vi "Periodic Tasks.vi"(8 "error in":errorcluster) -> ()   [LabVIEW 2020]
doc: "This VI runs in parallel to other tasks. It can contain as many user-defined periodic loops as you need. These can carry out PID or other sorts of timed response."
uses:
  State Machine.ctl
  Auto State Machine.ctl
  <vilib>/Rock Robotics/WPI/DriverStation/WPI_DriverStationRobotMode2.ctl
  <vilib>/Rock Robotics/WPI/DriverStation/WPI_DriverStationAllianceInfo.ctl
  <vilib>/Rock Robotics/WPI/ThirdParty/Phoenix-LabVIEW/Motor Controller/Controls/CTRE_Phoenix_MotorControl_NeutralMode.ctl
  <vilib>/Rock Robotics/WPI/ThirdParty/Phoenix-LabVIEW/Motor Controller/Controls/CTRE_Phoenix_MotorControl_ControlMode.ctl
  <vilib>/Rock Robotics/WPI/Solenoid/WPI_SolenoidValue.ctl
  <vilib>/Rock Robotics/WPI/Utilities/WPI_GetSetVariantRefNum.vi
  <vilib>/Rock Robotics/WPI/ThirdParty/Phoenix-LabVIEW/Motor Controller/Get/CTRE_Phoenix_MotorController_GetSupplyAndStatorCurrent_Enhanced.vi
  Lime.vi
  <vilib>/Rock Robotics/Network Tables/NT Read Number.vi
  <vilib>/Rock Robotics/WPI/ThirdParty/Phoenix-LabVIEW/Motor Controller/Get/CTRE_Phoenix_MotorController_GetSelectedSensorData.vi
  <vilib>/Rock Robotics/WPI/ThirdParty/Phoenix-LabVIEW/Motor Controller/Sensor/CTRE_Phoenix_MotorControl_SetIntegratedSensorPosition_TalonFX.vi
  <vilib>/Rock Robotics/WPI/ThirdParty/Phoenix-LabVIEW/Motor Controller/Get/CTRE_Phoenix_MotorController_IntegratedSensorData_TalonFX.vi
  <vilib>/Rock Robotics/WPI/Solenoid/WPI_SolenoidSetEnum.vi
  <vilib>/Rock Robotics/Network Tables/NT Read String.vi
  <vilib>/Rock Robotics/WPI/RobotDrive/WPI_RobotDriveMecanumDrive_Cartesian.vi
  <vilib>/Rock Robotics/Network Tables/NT Write Number.vi
  <vilib>/Rock Robotics/WPI/ThirdParty/Phoenix-LabVIEW/Pigeon IMU/CTRE_PigeonIMU_GetYPR.vi
  <vilib>/addons/control/pid/pid.llb/PID (DBL).vi
  <vilib>/Rock Robotics/Network Tables/NT Write Boolean.vi
  <vilib>/Rock Robotics/Network Tables/NT Read Boolean.vi
  <vilib>/addons/control/pid/NI_PID_pid.lvlib
panel:
  in  "setpoint 8":dbl=80.0 format="%.2f"
  in  "PID gains 9":T1={"proportional gain (Kc)"=1.0, "integral time (Ti, min)"=0.016, "derivative time (Td, min)"=0.0} {"derivative time (Td, min)" format="%.3f"; "integral time (Ti, min)" format="%.3f"; "proportional gain (Kc)" format="%.3f"}
  out "Yaw 9":dbl=80.3759765625
  in  "setpoint 7":dbl=80.0 format="%.2f"
  in  "PID gains 8":T1={"proportional gain (Kc)"=1.0, "integral time (Ti, min)"=0.016, "derivative time (Td, min)"=0.0} {"derivative time (Td, min)" format="%.3f"; "integral time (Ti, min)" format="%.3f"; "proportional gain (Kc)" format="%.3f"}
  out "Yaw 8":dbl=78.8818359375
  in  "Total Time":dbl=0.9 format="%#_13g"
  in  "Time Low":dbl=0.6 format="%#_13g"
  in  "x 3":dbl=0.5
  in  "setpoint 6":dbl=60.0 format="%.2f"
  in  "PID gains 7":T1={"proportional gain (Kc)"=1.0, "integral time (Ti, min)"=0.016, "derivative time (Td, min)"=0.0} {"derivative time (Td, min)" format="%.3f"; "integral time (Ti, min)" format="%.3f"; "proportional gain (Kc)" format="%.3f"}
  out "Yaw 7":dbl=60.029296875
  in  "setpoint 5":dbl=80.0 format="%.2f"
  in  "PID gains 6":T1={"proportional gain (Kc)"=1.0, "integral time (Ti, min)"=0.016, "derivative time (Td, min)"=0.0} {"derivative time (Td, min)" format="%.3f"; "integral time (Ti, min)" format="%.3f"; "proportional gain (Kc)" format="%.3f"}
  out "Yaw 6":dbl=80.3759765625
  in  "LL Deadband":dbl=4.0
  in  "Steering K 4":dbl=0.01
  in  "Min Steer 3":dbl=0.2
  in  "Aim Deadband 3":dbl=0.5
  in  "Steering K 2":dbl=0.02
  in  "Min Steer":dbl=0.2
  in  "Aim Deadband":dbl=0.01
  in  "setpoint 4":dbl format="%.2f"
  in  "PID gains 5":T1={"proportional gain (Kc)"=1.0, "integral time (Ti, min)"=0.016, "derivative time (Td, min)"=0.0} {"derivative time (Td, min)" format="%.3f"; "integral time (Ti, min)" format="%.3f"; "proportional gain (Kc)" format="%.3f"}
  out "Yaw 5":dbl=1.3623046875
  in  "Steering K 3":dbl=0.01
  in  "Min Steer 2":dbl=0.1
  in  "Aim Deadband 2":dbl=0.01
  in  "setpoint 2":dbl format="%.2f"
  in  "PID gains 3":T1={"proportional gain (Kc)"=1.0, "integral time (Ti, min)"=0.016, "derivative time (Td, min)"=0.0} {"derivative time (Td, min)" format="%.3f"; "integral time (Ti, min)" format="%.3f"; "proportional gain (Kc)" format="%.3f"}
  out "Yaw 3":dbl=1.3623046875
  in  "setpoint":dbl format="%.2f"
  in  "PID gains 2":T1={"proportional gain (Kc)"=1.0, "integral time (Ti, min)"=0.016, "derivative time (Td, min)"=0.0} {"derivative time (Td, min)" format="%.3f"; "integral time (Ti, min)" format="%.3f"; "proportional gain (Kc)" format="%.3f"}
  out "Yaw 2":dbl=0.263671875
  in  "Time Target (s)":dbl=0.1
  out "Timer":dbl
  out "Yaw":dbl
  in  "Oncontact 2 RPM 3":dbl=1100.0
  in  "Oncontact 2 RPM 2":dbl=1100.0
  in  "Auto On Contact RPM":dbl=1100.0
  out "Present (s)":dbl
  in  "Shooter Speed while intake":dbl=0.4
  out "Mag Current":dbl
  in  "Current Limit":dbl=25.0
  out "Mag Limit":bool
  out "Missed Mag":bool=TRUE
  in  "PID gains":T1={"proportional gain (Kc)"=1.0, "integral time (Ti, min)"=0.01, "derivative time (Td, min)"=0.0} {"derivative time (Td, min)" format="%.3f"; "integral time (Ti, min)" format="%.3f"; "proportional gain (Kc)" format="%.3f"}
  in  "Desired Mag Position":dbl format="%.2f"
  out "BB2":bool=TRUE
  out "BB1":bool
  out "Position":i32=403426
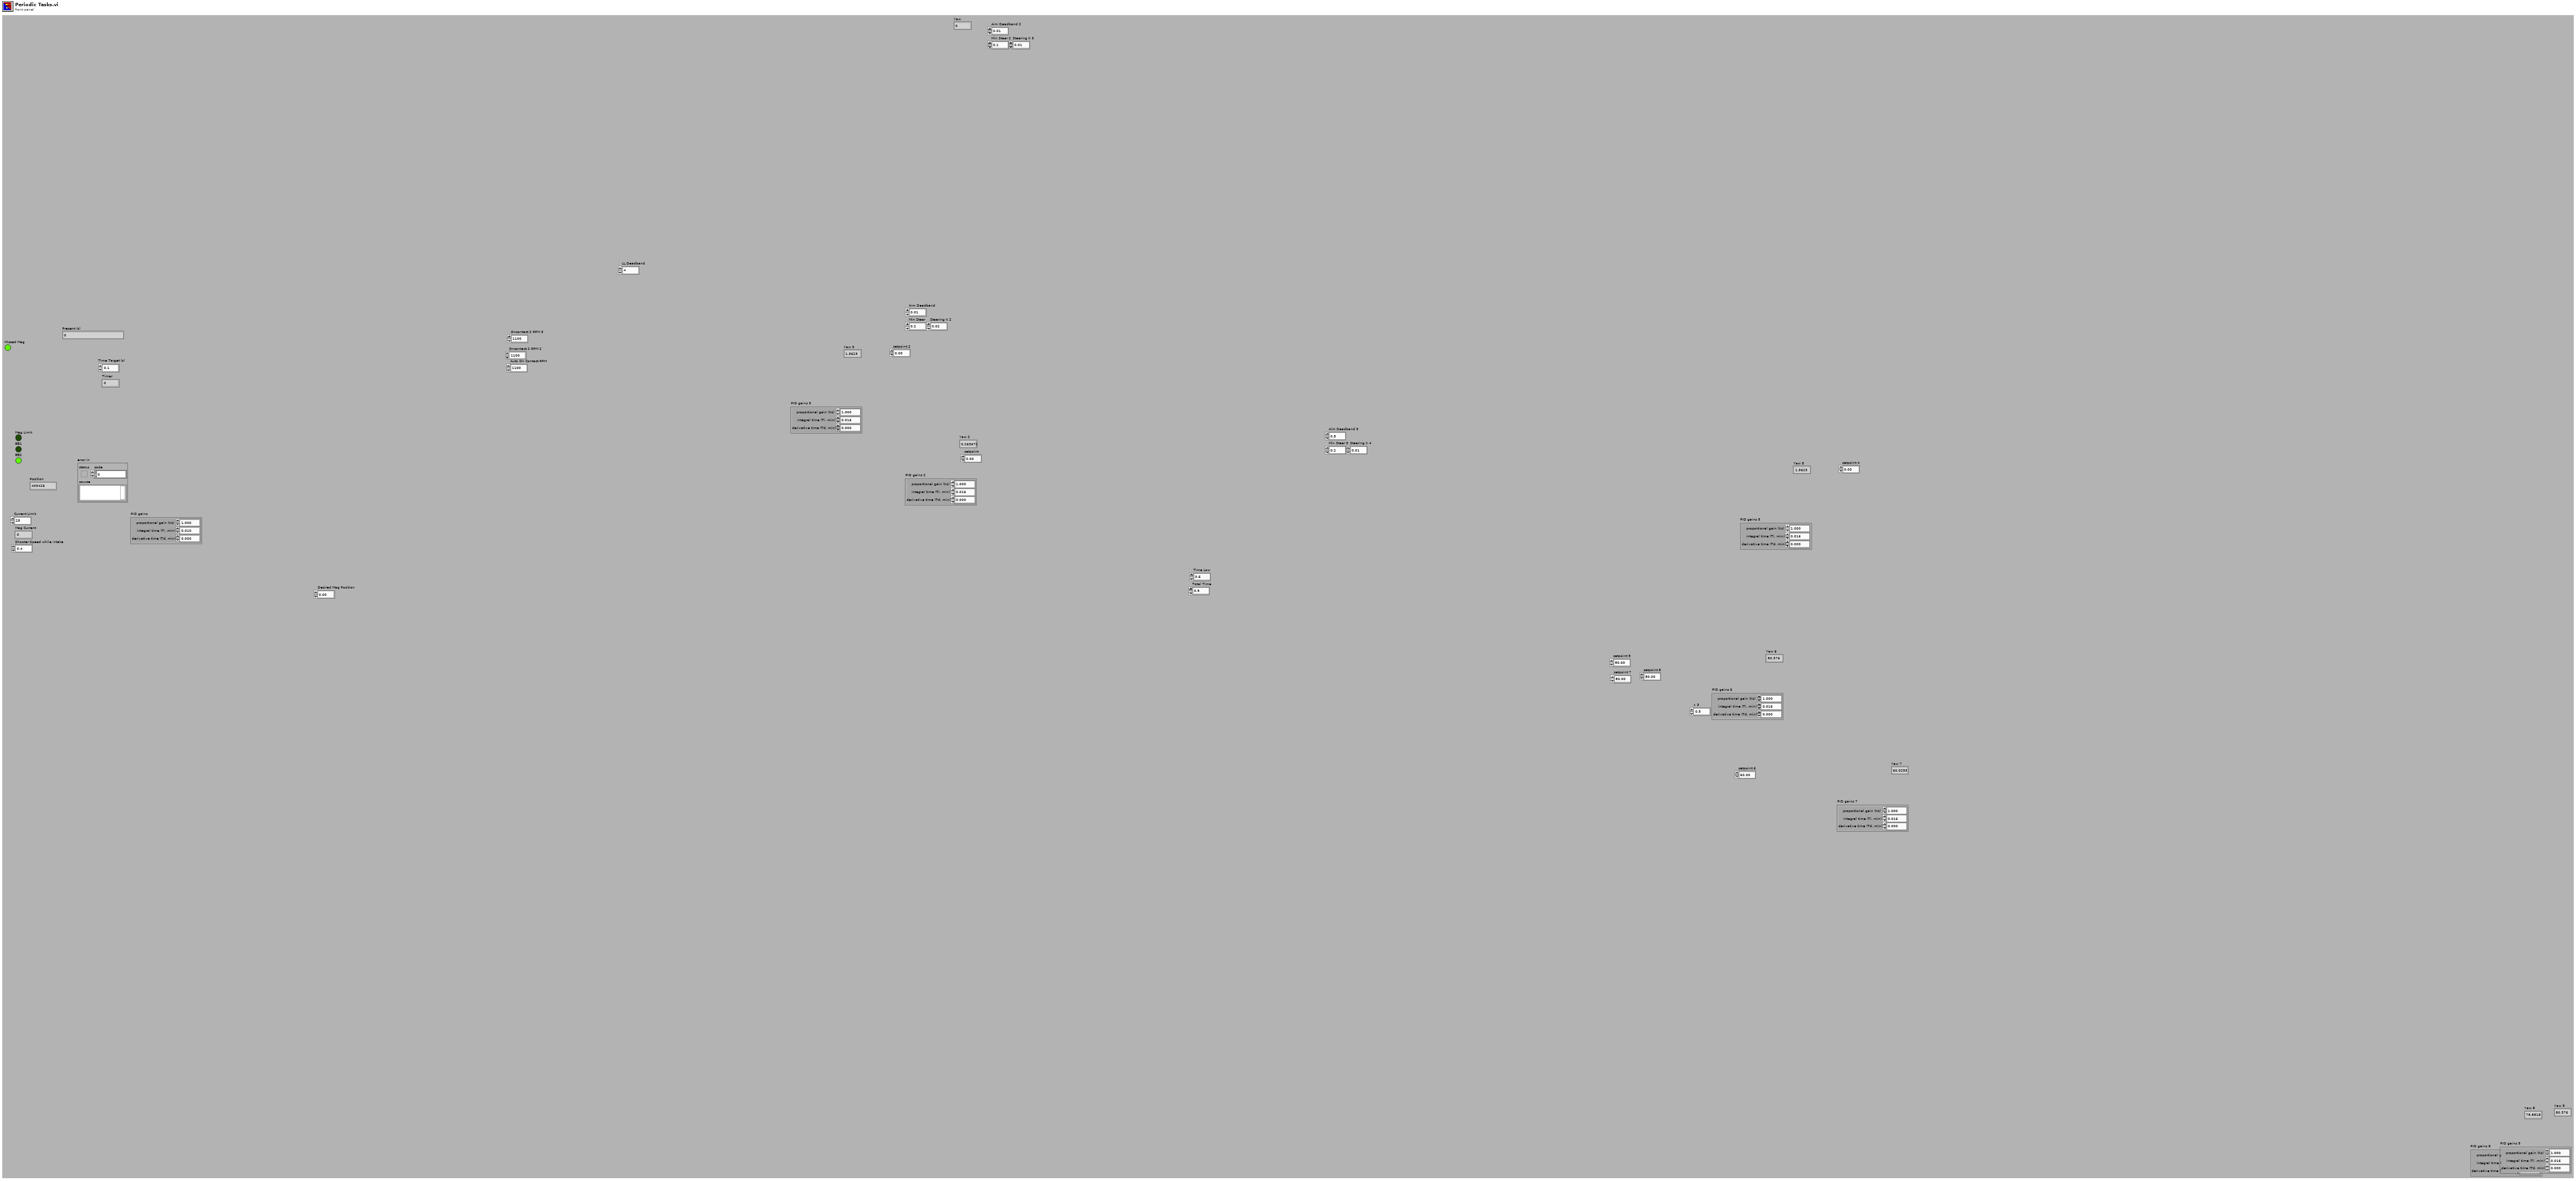
[diagram p1: front panel]
types:
  T1 = cluster{"proportional gain (Kc)":dbl, "integral time (Ti, min)":dbl, "derivative time (Td, min)":dbl}
  T2 = typedef "Auto State Machine.ctl" = enum16{"Auto Wait", "Shoot OC 1", "Shoot OC 2", "Shoot OC 3", "OC Reverse", "Cam Swap 1", "Cam Swap 2", "Cam Swap 3", "Go To Ball", "Intake", "Intake Up", "Rotate & Auger", "Limelight Happy?", "LL Shoot 1", "LL Shoot 2", "Pigeon Rotate", "Pigeon Shoot 1", "Pigeon Shoot 2", "Reverse", "Stop"}
  T3 = typedef "State Machine.ctl" = enum16{"Wait", "Conveyor 1", "Conveyor 2", "Dash Shoot 1", "Dash Shoot 2", "Low Goal Shoot 1", "Low Goal Shoot 2", "Launch Pad Shoot 1", "Launch Pad Shoot 2", "Wall Shoot 1", "Wall Shoot 2", "Mag Overcurrent"}
  T4 = typedef "CTRE_Phoenix_MotorControl_NeutralMode.ctl" = enum8{"EEPROMSetting", "Override to Coast", "Override to Brake"}
  T5 = typedef "WPI_DigitalInputDevRef.ctl" = cluster{"DevStatus":errorcluster, "DIO Channel":T6}
  T6 = typedef "FPGA_DIOChannel.ctl" = enum8{"DIO 0", "DIO 1", "DIO 2", "DIO 3", "DIO 4", "DIO 5", "DIO 6", "DIO 7", "DIO 8", "DIO 9", "DIO MXP 0", "DIO MXP 1", "DIO MXP 2", "DIO MXP 3", "DIO MXP 4", "DIO MXP 5", "DIO MXP 6", "DIO MXP 7", "DIO MXP 8", "DIO MXP 9", "DIO MXP 10", "DIO MXP 11", "DIO MXP 12", "DIO MXP 13", "DIO MXP 14", "DIO MXP 15", "SPI Port CS1", "SPI Port CS2", "SPI Port CS3", "SPI Port MISO", "SPI Port MOSI", "Invalid"}
  T7 = typedef "WPI_MotorControlDeviceRef.ctl" = cluster{"DeviceStatus":errorcluster, "Type":T8, "PWM":cluster{"PWM Channel":T9, "DeadBand":T10}, "CAN":cluster{"Device Number":u8, "SetOutput VI Ref":variant, "GetOutput VI Ref":variant, "Enable VI Ref":variant, "Disable VI Ref":variant, "Data":variant}, "Invert":bool, "DIO PWM":cluster{"PWM \"Enable\" Channel":T9, "DIOChannel":T6, "PWM Rate":dbl}}
  T8 = typedef "WPI_MotorControlType.ctl" = enum16{"PWM", "CAN", "DIO PWM"}
  T9 = typedef "FPGA_DIOPWMChannel.ctl" = enum8{"PWM 0", "PWM 1", "PWM 2", "PWM 3", "PWM 4", "PWM 5", "PWM 6", "PWM 7", "PWM 8", "PWM 9", "PWM MXP 0", "PWM MXP 1", "PWM MXP 2", "PWM MXP 3", "PWM MXP 4", "PWM MXP 5", "PWM MXP 6", "PWM MXP 7", "PWM MXP 8", "PWM MXP 9", "Invalid"}
  T10 = typedef "WPI_PWMDeadband.ctl" = cluster{"Name":string, "maxPositivePwm":i32, "minPositivePwm":i32, "centerPwm":i32, "maxNegativePwm":i32, "minNegativePwm":i32, "angularRange":u16}
  T11 = typedef "CTRE_PigeonIMU_DeviceRef.ctl" = cluster{"DeviceStatus":errorcluster, "Device Number":u8, "Type":T12, "Device ID":u32, "Handle":u64, "UsageFrame":u32, "Library Path":path}
  T12 = typedef "CTRE_PigeonIMU_ConnectionType.ctl" = u32
  T13 = typedef "WPI_DriverStationRobotMode2.ctl" = enum16{"Autonomous Disabled", "Autonomous Enabled", "Teleop Disabled", "Teleop Enabled", "Disconnected", "Finish", "Test Disabled", "Test Enabled", "Emergency Stopped"}
  T14 = typedef "WPI_JoystickDevRef.ctl" = cluster{"Device":T15}
  T15 = typedef "WPI_JoystickDeviceEnum.ctl" = enum16{"USB 0", "USB 1", "USB 2", "USB 3", "USB 4", "USB 5"}
  T16 = typedef "CTRE_Phoenix_MotorControl_ControlMode.ctl" = u16
  T17 = typedef "WPI_DriverStationAllianceInfo.ctl" = enum16{"Red", "Blue", "Invalid"}
  T18 = typedef "WPI_SolenoidValue.ctl" = enum16{"Off", "On", "Forward", "Reverse"}
  T19 = typedef "WPI_SolenoidDevRef.ctl" = cluster{"DevStatus":errorcluster, "Pneumatics Control Module":u8, "Forward Solenoid Channel":T20, "Reverse Solenoid Channel":T20}
  T20 = typedef "WPI_SolenoidChannel.ctl" = enum8{"Solenoid 0", "Solenoid 1", "Solenoid 2", "Solenoid 3", "Solenoid 4", "Solenoid 5", "Solenoid 6", "Solenoid 7", "Solenoid 8", "Solenoid 9", "Solenoid 10", "Solenoid 11", "Solenoid 12", "Solenoid 13", "Solenoid 14", "Solenoid 15", "Invalid"}
  T21 = typedef "WPI_RobotDriveDevRef.ctl" = cluster{"DevStatus":errorcluster, "Motors[]":T7[], "Square Inputs":bool, "Max Output":dbl}
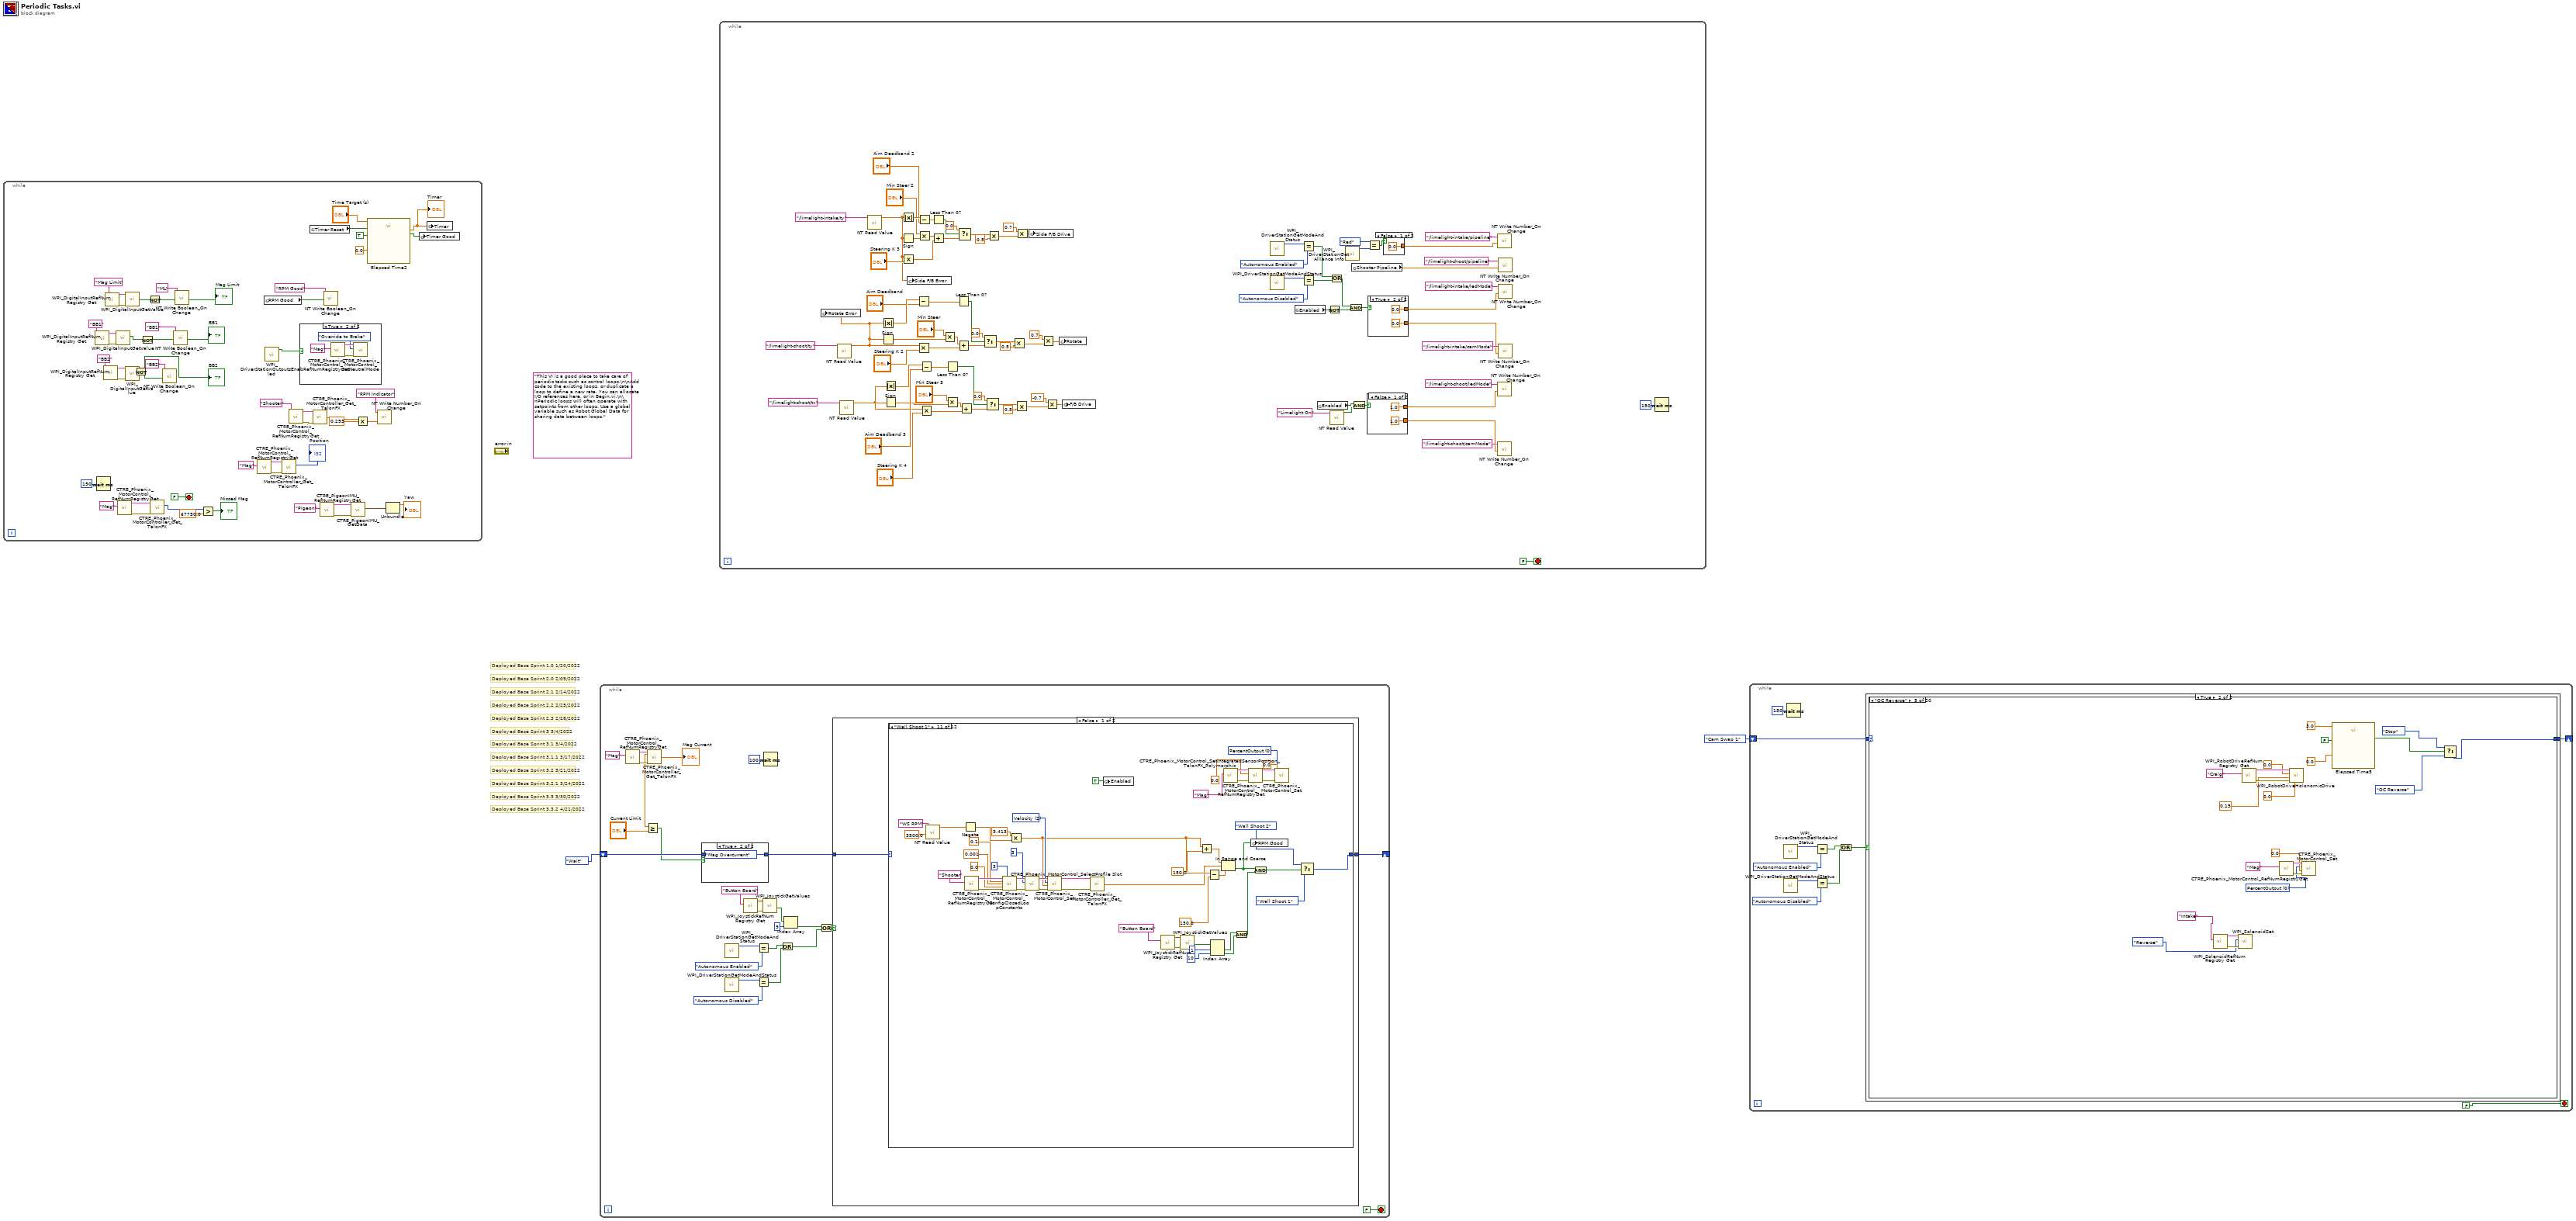
[diagram p0: block diagram]
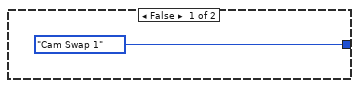
[diagram p2: hidden frame]
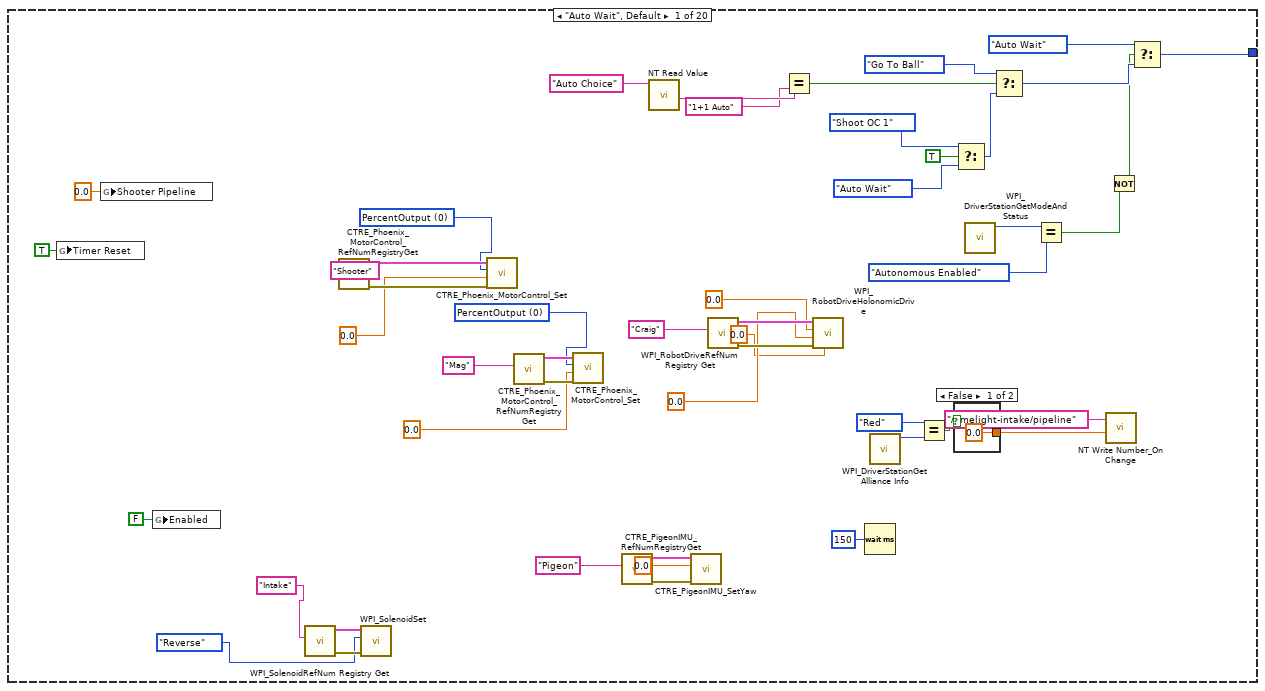
[diagram p3: hidden frame]
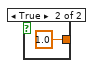
[diagram p4: hidden frame]
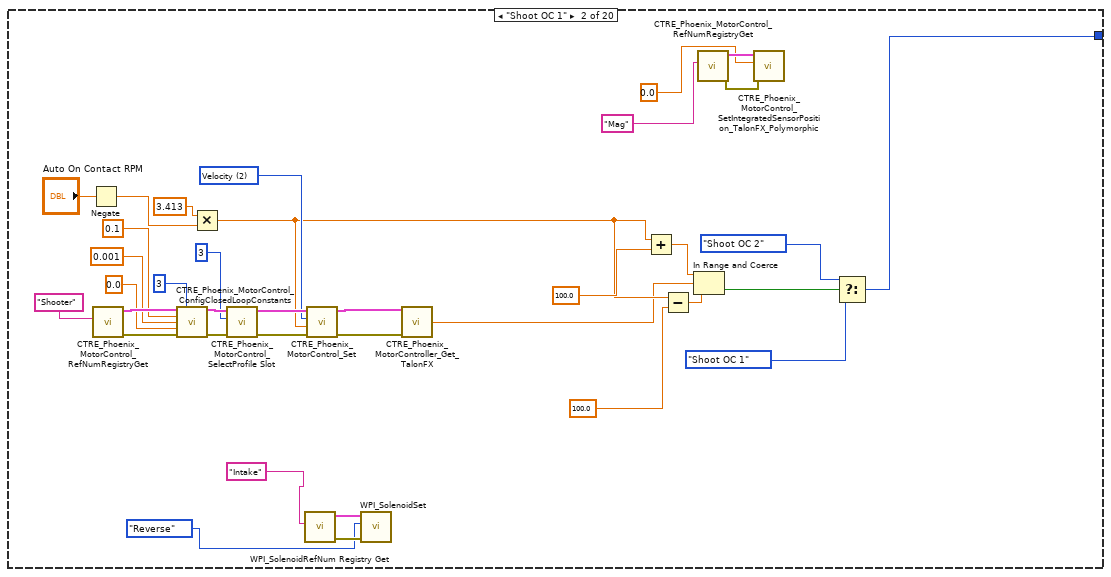
[diagram p5: hidden frame]
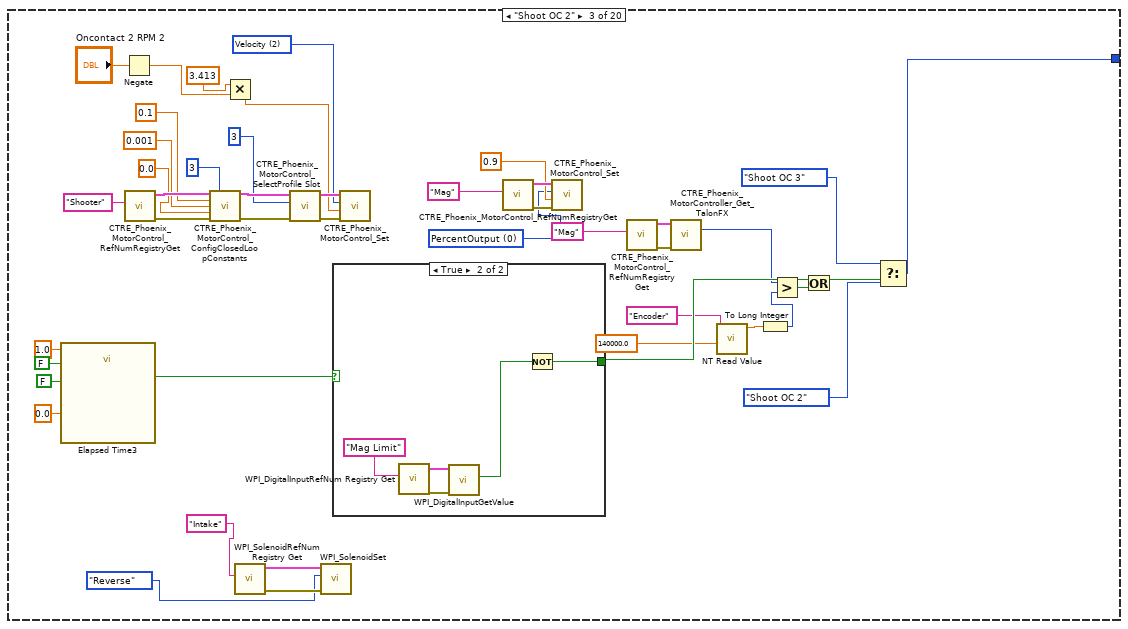
[diagram p6: hidden frame]
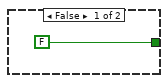
[diagram p7: hidden frame]
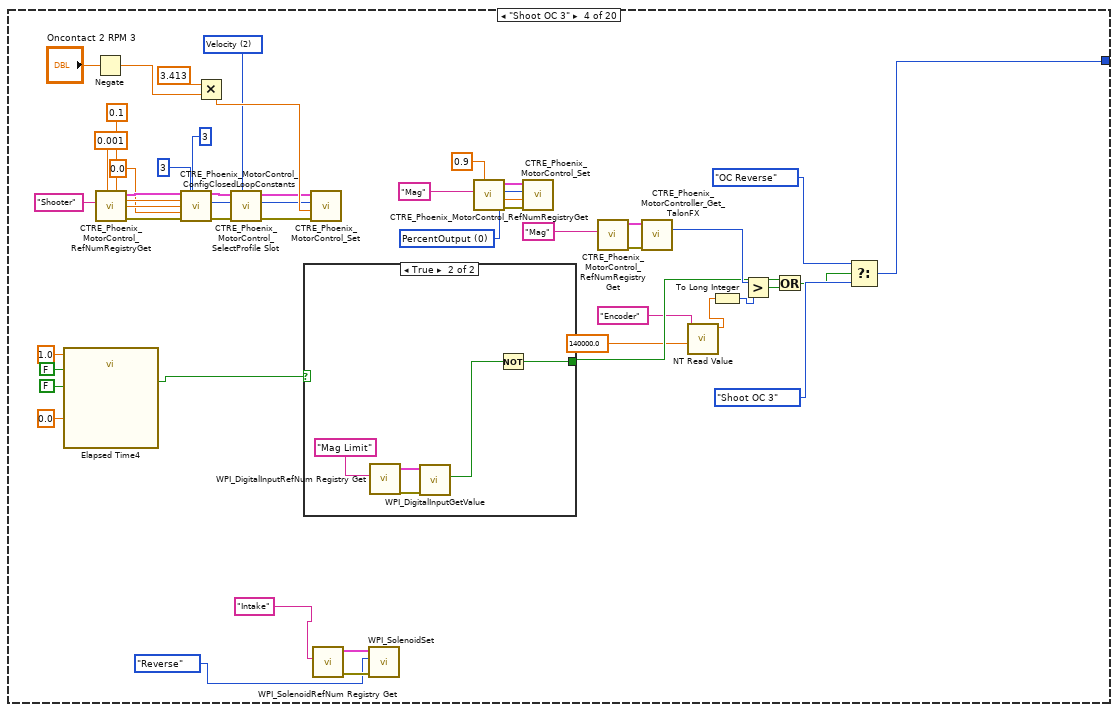
[diagram p8: hidden frame]
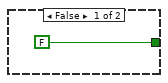
[diagram p9: hidden frame]
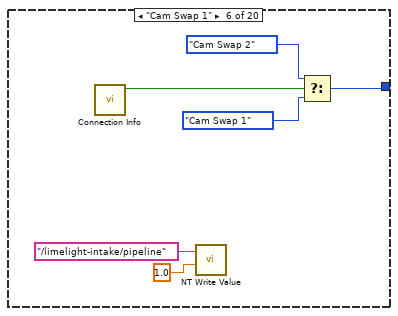
[diagram p10: hidden frame]
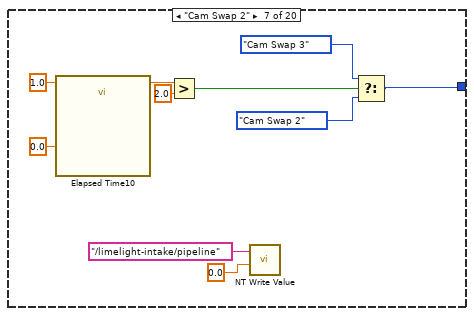
[diagram p11: hidden frame]
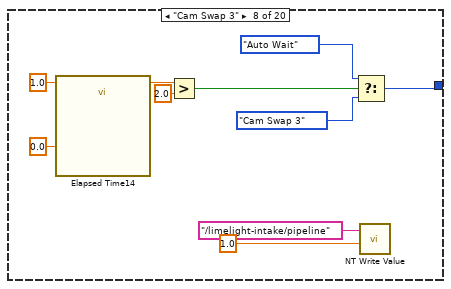
[diagram p12: hidden frame]
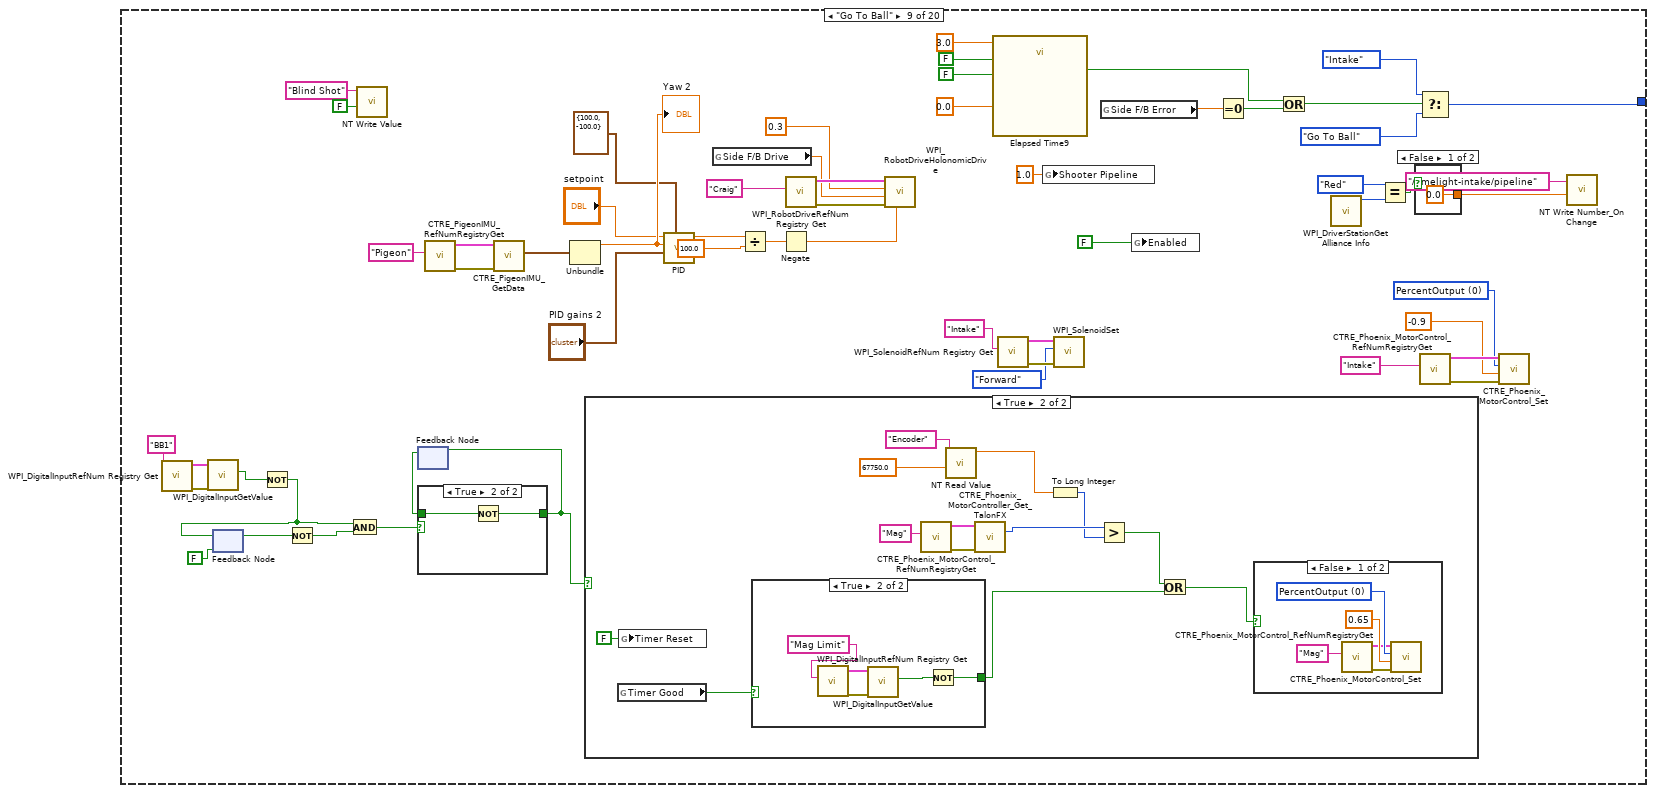
[diagram p13: hidden frame]
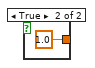
[diagram p14: hidden frame]
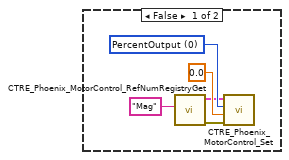
[diagram p16: hidden frame]
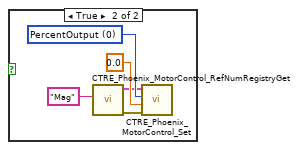
[diagram p17: hidden frame]
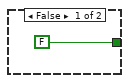
[diagram p18: hidden frame]
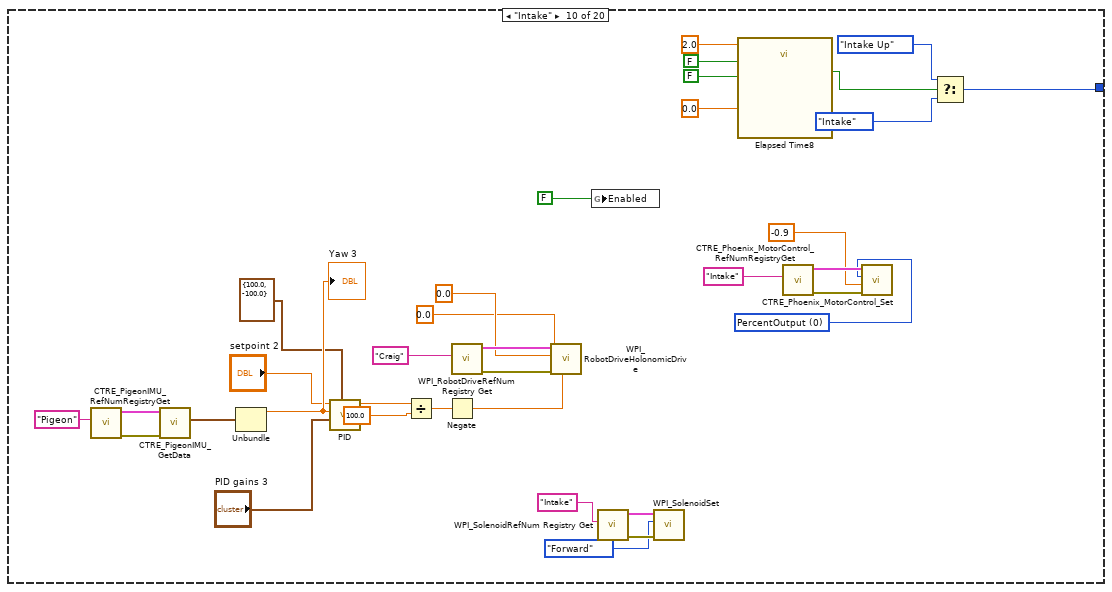
[diagram p19: hidden frame]
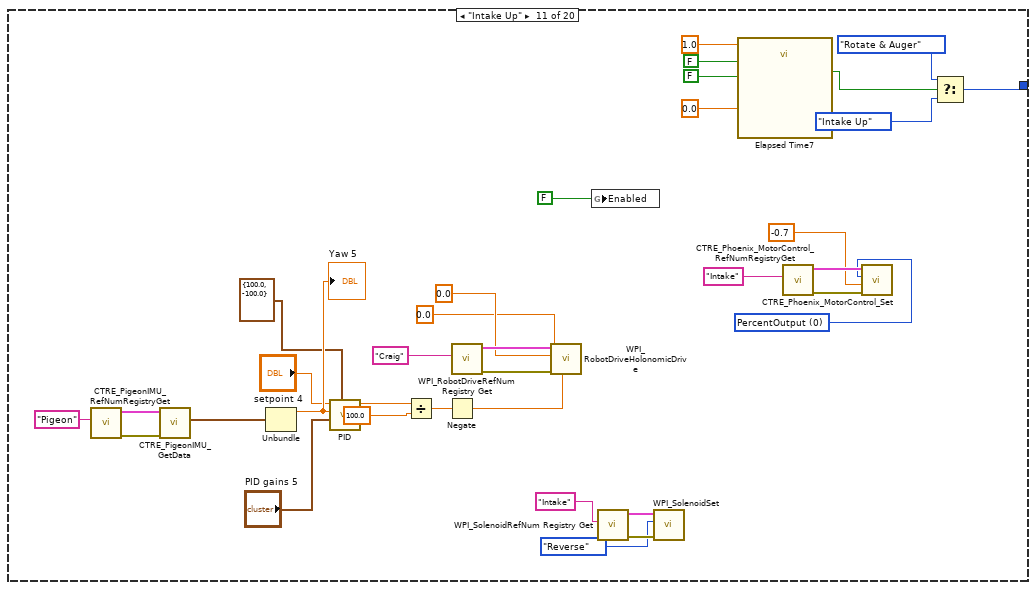
[diagram p20: hidden frame]
diagram:
  (unwired) "This VI is a good place to take care of periodic tasks such as control loops.\n\nAdd code to the existing loops, or duplicate a loop to define a new rate. You can allocate I/O references here, or in Begin.vi.\n\nPeriodic loops will often operate with setpoints from other loops. Use a global variable such as Robot Global Data for sharing data between loops."
  # "Deployed Base Sprint 3.3.2 4/21/2022"
  # "Deployed Base Sprint 3.3 3/30/2022"
  # "Deployed Base Sprint 3.2.1 3/24/2022"
  # "Deployed Base Sprint 3.2 3/21/2022"
  # "Deployed Base Sprint 3.1.1 3/17/2022"
  # "Deployed Base Sprint 3.1 3/4/2022"
  # "Deployed Base Sprint 3 3/4/2022"
  # "Deployed Base Sprint 2.3 2/28/2022"
  # "Deployed Base Sprint 2.2 2/25/2022"
  # "Deployed Base Sprint 2.1 2/14/2022"
  # "Deployed Base Sprint 2.0 2/09/2022"
  # "Deployed Base Sprint 1.0 1/20/2022"
  n1 = while {
    stop <- FALSE stop-if-true
    n2 = call <vilib>:"WPI_DigitalInputRefNum Registry Get.vi"("refnum name"="BB1") -> ("error out"=w48:errorcluster, "DigitalInputDevRef"=w47:T5)  [unwired: 9 in]
    n3 = Wait (ms)(milliseconds to wait=u32 150) -> ()  [unwired: 1 out]
    n4 = call <vilib>:"WPI_DigitalInputRefNum Registry Get.vi"("refnum name"="BB2") -> ("error out"=w45:errorcluster, "DigitalInputDevRef"=w46:T5)  [unwired: 9 in]
    n5 = call <vilib>:"WPI_DigitalInputRefNum Registry Get.vi"("refnum name"="Mag Limit") -> ("error out"=w20:errorcluster, "DigitalInputDevRef"=w21:T5)  [unwired: 9 in]
    n6 = call <vilib>:"WPI_DigitalInputGetValue.vi"("error in (no error)"=w48, "DigitalInputDevRef"=w47) -> ("Value"=w44:bool)  [unwired: 7 in, 2 out]
    n7 = call <vilib>:"CTRE_Phoenix_MotorControl_RefNumRegistryGet.vi"("refnum name"="Mag") -> ("error out"=w28:errorcluster, "PhoenixMotorControlDevRef"=w27:T7)  [unwired: 9 in]
    n8 = call <vilib>:"WPI_DigitalInputGetValue.vi"("error in (no error)"=w45, "DigitalInputDevRef"=w46) -> ("Value"=w37:bool)  [unwired: 7 in, 2 out]
    n9 = call <vilib>:"WPI_DigitalInputGetValue.vi"("error in (no error)"=w20, "DigitalInputDevRef"=w21) -> ("Value"=w22:bool)  [unwired: 7 in, 2 out]
    n10 = Not(x=w37) -> (.not. x?=w36:bool)
    "BB2" <- w36
    n11 = Not(x=w44) -> (.not. x?=w38:bool)
    "BB1" <- w38
    n12 = Not(x=w22) -> (.not. x?=w17:bool)
    "Mag Limit" <- w17
    n13 = call-poly <vilib>:"CTRE_Phoenix_MotorController_Get_TalonFX.vi"("PhoenixMotorControlDevRef"=w27, "error in"=w28) -> ("Position (Raw Sensor Units)"=w25:i32)  [unwired: 10 in, 3 out]
    n14 = call "NT Write Boolean_On Change.vi"("Boolean"=w36, "Name"="BB2") -> ()  [unwired: 9 in, 1 out]
    n15 = call "NT Write Boolean_On Change.vi"("Boolean"=w38, "Name"="BB1") -> ()  [unwired: 9 in, 1 out]
    n16 = call "NT Write Boolean_On Change.vi"("Boolean"=w17, "Name"="ML") -> ()  [unwired: 9 in, 1 out]
    n17 = Greater?(x=w25, y=67750.0) -> (0:→"Missed Mag":bool)
    n18 = call <vilib>:"CTRE_Phoenix_MotorControl_RefNumRegistryGet.vi"("refnum name"="Mag") -> ("error out"=w41:errorcluster, "PhoenixMotorControlDevRef"=w42:T7)  [unwired: 9 in]
    n19 = global read "Lime.vi" "RPM Good"() -> (w11:bool)
    n20 = call <vilib>:"WPI_DriverStationOutputsEnabled.vi"() -> ("OutputsEnabled?"=w39:bool)  [unwired: 10 in, 1 out]
    n21 = call-poly <vilib>:"CTRE_Phoenix_MotorController_Get_TalonFX.vi"("PhoenixMotorControlDevRef"=w42, "error in"=w41) -> ("Position (Raw Sensor Units)"=→"Position":i32)  [unwired: 10 in, 3 out]
    n22 = call <vilib>:"CTRE_Phoenix_MotorControl_RefNumRegistryGet.vi"("refnum name"="Shooter") -> ("error out"=w30:errorcluster, "PhoenixMotorControlDevRef"=w29:T7)  [unwired: 9 in]
    n23 = case shown="True" w39 {
      frame False {
        n24 = call <vilib>:"CTRE_Phoenix_MotorControl_RefNumRegistryGet.vi"("refnum name"="Mag") -> ("error out"=w56:errorcluster, "PhoenixMotorControlDevRef"=w55:T7)  [unwired: 9 in]
        n25 = call <vilib>:"CTRE_Phoenix_MotorControl_SetNeutralMode.vi"("error in (no error)"=w56, "Motor Control Neutral Mode"=CTRE_Phoenix_MotorControl_NeutralMode."Override to Coast", "PhoenixMotorControlDevRef"=w55) -> ()  [unwired: 7 in, 2 out]
      }
      frame True {
        n26 = call <vilib>:"CTRE_Phoenix_MotorControl_RefNumRegistryGet.vi"("refnum name"="Mag") -> ("error out"=w60:errorcluster, "PhoenixMotorControlDevRef"=w59:T7)  [unwired: 9 in]
        n27 = call <vilib>:"CTRE_Phoenix_MotorControl_SetNeutralMode.vi"("error in (no error)"=w60, "Motor Control Neutral Mode"=CTRE_Phoenix_MotorControl_NeutralMode."Override to Brake", "PhoenixMotorControlDevRef"=w59) -> ()  [unwired: 7 in, 2 out]
      }
    }
    n28 = global read "Lime.vi" "Timer Reset"() -> (w8:bool)
    n29 = call-poly <vilib>:"CTRE_Phoenix_MotorController_Get_TalonFX.vi"("PhoenixMotorControlDevRef"=w29, "error in"=w30) -> ("Velocity"=w34:dbl)  [unwired: 9 in, 4 out]
    n30 = call <vilib>:"CTRE_PigeonIMU_RefNumRegistryGet.vi"("refnum name"="Pigeon") -> ("error out"=w15:errorcluster, "PigeonIMUDevRef"=w16:T11)  [unwired: 9 in]
    n31 = call "NT Write Boolean_On Change.vi"("Boolean"=w11, "Name"="RPM Good") -> ()  [unwired: 9 in, 1 out]
    n32 = call-poly <vilib>:"CTRE_PigeonIMU_GetData.vi"("error in (no error)"=w15, "PigeonIMUDevRef"=w16) -> ("Yaw Pitch Roll"=w13:cluster{"Yaw":dbl, "Pitch":dbl, "Roll":dbl})  [unwired: 7 in, 2 out]
    n33 = Multiply(x=w34, y=0.293) -> (x*y=w31:dbl)
    n34 = call "Elapsed Time2"("Time Target (s)"="Time Target (s)", "Reset"=w8, "Auto Reset"=TRUE, "Set Start Time (s)"=0.0) -> ("Elapsed Time (s)"=w4:dbl, "Time has Elapsed"=w7:bool)  [unwired: 8 in, 6 out]
    "Timer" <- w4
    n35 = call "NT Write Number_On Change.vi"("Numeric"=w31, "Name"="RPM Indicator") -> ()  [unwired: 9 in, 1 out]
    n36 = Unbundle(w13) -> ("Yaw"=→"Yaw":dbl)  [unwired: 2 out]
    n37 = global write "Lime.vi" "Timer Good"(w7) -> ()
    n38 = global write "Lime.vi" "Timer"(w4) -> ()
  }
  n39 = while {
    shift-right: [w81] -> _
    shift-left: State_Machine."Wait" -> [w77]
    stop <- FALSE stop-if-true
    n40 = call <vilib>:"CTRE_Phoenix_MotorControl_RefNumRegistryGet.vi"("refnum name"="Mag") -> ("error out"=w74:errorcluster, "PhoenixMotorControlDevRef"=w75:T7)  [unwired: 9 in]
    n41 = call-poly <vilib>:"CTRE_Phoenix_MotorController_Get_TalonFX.vi"("PhoenixMotorControlDevRef"=w75, "error in"=w74) -> ("Supply Current"=w73:dbl, "Stator Current"=→"Mag Current":dbl)  [unwired: 10 in, 2 out]
    n42 = Greater Or Equal?(x=w73, y="Current Limit") -> (x >= y?=w70:bool)
    n43 = case shown="True" w70 {
      tunnel: [w88 State_Machine."Mag Overcurrent"] -> w78
      tunnel: w77 -> [w88 _]
      frame False {
      }
      frame True {
      }
    }
    n44 = call <vilib>:"WPI_DriverStationGetModeAndStatus.vi"() -> ("Robot Mode"=w68:T13)  [unwired: 10 in, 1 out]
    n45 = call <vilib>:"WPI_DriverStationGetModeAndStatus.vi"() -> ("Robot Mode"=w66:T13)  [unwired: 10 in, 1 out]
    n46 = call <vilib>:"WPI_JoystickRefNum Registry Get.vi"("refnum name"="Button Board") -> ("error out"=w87:errorcluster, "JoystickDevRef"=w86:T14)  [unwired: 9 in]
    n47 = Equal?(x=w68, y=WPI_DriverStationRobotMode2."Autonomous Enabled") -> (x = y?=w64:bool)
    n48 = Equal?(x=w66, y=WPI_DriverStationRobotMode2."Autonomous Disabled") -> (x = y?=w63:bool)
    n49 = call <vilib>:"WPI_JoystickGetValues.vi"("error in (no error)"=w87, "JoystickDevRef"=w86) -> ("Buttons"=w84:bool[])  [unwired: 5 in, 4 out]
    n50 = Wait (ms)(milliseconds to wait=u32 100) -> ()  [unwired: 1 out]
    n51 = Or(x=w64, y=w63) -> (x .or. y?=w62:bool)
    n52 = Index Array(array=w84, index=9) -> (element=w80:bool)
    n53 = Or(x=w80, y=w62) -> (x .or. y?=w69:bool)
    n54 = case shown="False" w69 {
      tunnel: w78 -> [w91 _]
      tunnel: [w90 State_Machine."Wait"] -> w81
      frame False {
        n55 = case shown="\"Wall Shoot 1\"" w91 {
          tunnel: [w110 w153 w184 w239 w296 w329 w349 w396 w441 w489 w533 w583] -> w90
          frame "Wait", Default {
            w104 = T16 0 items=["PercentOutput"=0, "Position"=1, "Velocity"=2, "Current"=3, "Follower"=5, "MotionProfile"=6, "MotionMagic"=7, "MotionProfileArc"=10, "Disabled"=15] ("Control Mode")
            w101 = T16 0 items=["PercentOutput"=0, "Position"=1, "Velocity"=2, "Current"=3, "Follower"=5, "MotionProfile"=6, "MotionMagic"=7, "MotionProfileArc"=10, "Disabled"=15] ("Control Mode")
            n56 = call <vilib>:"WPI_JoystickRefNum Registry Get.vi"("refnum name"="Button Board") -> ("error out"=w144:errorcluster, "JoystickDevRef"=w145:T14)  [unwired: 9 in]
            n57 = call <vilib>:"WPI_JoystickGetValues.vi"("error in (no error)"=w144, "JoystickDevRef"=w145) -> ("Buttons"=w141:bool[])  [unwired: 5 in, 4 out]
            n58 = Index Array(array=w141, index #1=0 ("index"), index #2=3 ("index"), index #3=6 ("index"), index #4=1 ("index")) -> (element #1=w140:bool, element #2=w117:bool, element #3=w118:bool, element #4=w93:bool)
            n59 = call <vilib>:"WPI_DigitalInputRefNum Registry Get.vi"("refnum name"="BB2") -> ("error out"=w130:errorcluster, "DigitalInputDevRef"=w129:T5)  [unwired: 9 in]
            n60 = call <vilib>:"WPI_DigitalInputRefNum Registry Get.vi"("refnum name"="BB1") -> ("error out"=w133:errorcluster, "DigitalInputDevRef"=w134:T5)  [unwired: 9 in]
            n61 = call <vilib>:"WPI_JoystickRefNum Registry Get.vi"("refnum name"="Joystick 0") -> ("error out"=w135:errorcluster, "JoystickDevRef"=w136:T14)  [unwired: 9 in]
            n62 = call <vilib>:"WPI_DigitalInputGetValue.vi"("error in (no error)"=w130, "DigitalInputDevRef"=w129) -> ("Value"=w127:bool)  [unwired: 7 in, 2 out]
            n63 = call <vilib>:"WPI_DigitalInputGetValue.vi"("error in (no error)"=w133, "DigitalInputDevRef"=w134) -> ("Value"=w128:bool)  [unwired: 7 in, 2 out]
            n64 = Select(t=State_Machine."Wall Shoot 1", s=w93, f=State_Machine."Wait") -> (s? t:f=w96:T3)
            n65 = Not(x=w127) -> (.not. x?=w123:bool)
            n66 = Not(x=w128) -> (.not. x?=w126:bool)
            n67 = Select(t=State_Machine."Launch Pad Shoot 1", s=w118, f=w96) -> (s? t:f=w115:T3)
            n68 = call <vilib>:"WPI_JoystickGetValues.vi"("error in (no error)"=w135, "JoystickDevRef"=w136) -> ("Buttons"=w138:bool[])  [unwired: 5 in, 4 out]
            n69 = Select(t=State_Machine."Low Goal Shoot 1", s=w117, f=w115) -> (s? t:f=w116:T3)
            n70 = Index Array(array=w138, index=1) -> (element=w121:bool)
            n71 = Select(t=FALSE, s=w123, f=w126) -> (s? t:f=w125:bool)
            n72 = call <vilib>:"CTRE_Phoenix_MotorControl_RefNumRegistryGet.vi"("refnum name"="Shooter") -> ("error out"=w108:errorcluster, "PhoenixMotorControlDevRef"=w109:T7)  [unwired: 9 in]
            n73 = Or(x=w121, y=w125) -> (x .or. y?=w122:bool)
            n74 = Select(t=State_Machine."Dash Shoot 1", s=w140, f=w116) -> (s? t:f=w146:T3)
            n75 = Select(t=State_Machine."Conveyor 1", s=w122, f=w146) -> (s? t:f=w110:T3)
            n76 = call <vilib>:"CTRE_Phoenix_MotorControl_Set.vi"("error in (no error)"=w108, "Output"=0.0, "Control Mode"=w104, "PhoenixMotorControlDevRef"=w109) -> ()  [unwired: 6 in, 2 out]
            n77 = call <vilib>:"CTRE_Phoenix_MotorControl_RefNumRegistryGet.vi"("refnum name"="Mag") -> ("error out"=w106:errorcluster, "PhoenixMotorControlDevRef"=w107:T7)  [unwired: 9 in]
            n78 = call <vilib>:"CTRE_Phoenix_MotorControl_Set.vi"("error in (no error)"=w106, "Output"=0.0, "Control Mode"=w101, "PhoenixMotorControlDevRef"=w107) -> ()  [unwired: 6 in, 2 out]
            n79 = global write "Lime.vi" "Timer Reset"(TRUE ("RPM Good")) -> ()
            n80 = global write "Lime.vi" "RPM Good"(FALSE ("RPM Good")) -> ()
            n81 = global write "Lime.vi" "Enabled"(FALSE ("Enabled")) -> ()
          }
          frame "Conveyor 1" {
            w162 = u32 15 ("milliseconds to wait")
            n82 = call <vilib>:"CTRE_Phoenix_MotorControl_RefNumRegistryGet.vi"("refnum name"="Mag") -> ("error out"=w150:errorcluster, "PhoenixMotorControlDevRef"=w151:T7)  [unwired: 9 in]
            n83 = call <vilib>:"CTRE_Phoenix_MotorControl_SetSelectedSensorPosition.vi"("error in (no error)"=w150, "New Sensor Position"=0, "PhoenixMotorControlDevRef"=w151) -> ()  [unwired: 7 in, 2 out]
            n84 = Wait (ms)(milliseconds to wait=w162) -> (millisecond timer value=w163:u32)
            n85 = call <vilib>:"WPI_DigitalInputRefNum Registry Get.vi"("refnum name"="BB2") -> ("error out"=w155:errorcluster, "DigitalInputDevRef"=w154:T5)  [unwired: 9 in]
            n86 = Greater?(x=w163, y=w162) -> (0:w159:bool)
            n87 = call <vilib>:"WPI_DigitalInputGetValue.vi"("error in (no error)"=w155, "DigitalInputDevRef"=w154) -> ("Value"=w148:bool)  [unwired: 7 in, 2 out]
            n88 = Not(x=w148) -> (.not. x?=w147:bool)
            n89 = Select(t=State_Machine."Conveyor 2", s=w159, f=State_Machine."Conveyor 1") -> (s? t:f=w158:T3)
            n90 = Select(t=State_Machine."Wait", s=w147, f=w158) -> (s? t:f=w153:T3)
          }
          frame "Conveyor 2" {
            w180 = T16 0 items=["PercentOutput"=0, "Position"=1, "Velocity"=2, "Current"=3, "Follower"=5, "MotionProfile"=6, "MotionMagic"=7, "MotionProfileArc"=10, "Disabled"=15] ("Control Mode")
            w187 = T16 0 items=["PercentOutput"=0, "Position"=1, "Velocity"=2, "Current"=3, "Follower"=5, "MotionProfile"=6, "MotionMagic"=7, "MotionProfileArc"=10, "Disabled"=15] ("Control Mode")
            n91 = disable-structure shown="Disabled" {
              disable-tunnel: [w193 _] -> _
              frame Disabled {
                w201 = T16 0 items=["PercentOutput"=0, "Position"=1, "Velocity"=2, "Current"=3, "Follower"=5, "MotionProfile"=6, "MotionMagic"=7, "MotionProfileArc"=10, "Disabled"=15] ("Control Mode")
                n92 = call <vilib>:"CTRE_Phoenix_MotorControl_RefNumRegistryGet.vi"("refnum name"="Mag") -> ("error out"=w200:errorcluster, "PhoenixMotorControlDevRef"=w199:T7)  [unwired: 9 in]
                n93 = call-poly <vilib>:"CTRE_Phoenix_MotorController_Get_TalonFX.vi"("PhoenixMotorControlDevRef"=w199, "error in"=w200) -> ("Position"=w207:dbl)  [unwired: 9 in, 4 out]
                n94 = call-poly <vilib>:"PID.vi"("PID gains"="PID gains", "process variable"=w207, "setpoint"="Desired Mag Position") -> ("output"=w204:dbl)  [unwired: 7 in, 1 out]
                n95 = call <vilib>:"CTRE_Phoenix_MotorControl_RefNumRegistryGet.vi"("refnum name"="Mag") -> ("error out"=w203:errorcluster, "PhoenixMotorControlDevRef"=w202:T7)  [unwired: 9 in]
                n96 = call <vilib>:"CTRE_Phoenix_MotorControl_Set.vi"("error in (no error)"=w203, "Output"=w204, "Control Mode"=w201, "PhoenixMotorControlDevRef"=w202) -> ()  [unwired: 6 in, 2 out]
                n97 = Add(x="Desired Mag Position", y=1000.0) -> (x+y=w205:dbl)
                n98 = Subtract(x="Desired Mag Position", y=1000.0) -> (x-y=w206:dbl)
                n99 = In Range and Coerce(upper limit=w205, x=w207, lower limit=w206) -> (In Range?=w193:bool)  [unwired: 1 out]
              }
              frame Enabled {
              }
            }
            n100 = disable-structure shown="Disabled" {
              frame Disabled {
                w191 = u32 125 ("milliseconds to wait")
                n101 = Wait (ms)(milliseconds to wait=w191) -> (millisecond timer value=w192:u32)
                n102 = Greater?(x=w192, y=w191) -> ()  [unwired: 1 out]
              }
              frame Enabled {
              }
            }
            n103 = global read "Lime.vi" "Timer Good"() -> (w165:bool)
            n104 = call <vilib>:"CTRE_Phoenix_MotorControl_RefNumRegistryGet.vi"("refnum name"="Mag") -> ("error out"=w178:errorcluster, "PhoenixMotorControlDevRef"=w179:T7)  [unwired: 9 in]
            n105 = case shown="False" w165 {
              tunnel: [FALSE w210] -> w176
              frame False {
              }
              frame True {
                n106 = call <vilib>:"WPI_DigitalInputRefNum Registry Get.vi"("refnum name"="Mag Limit") -> ("error out"=w213:errorcluster, "DigitalInputDevRef"=w214:T5)  [unwired: 9 in]
                n107 = call <vilib>:"WPI_DigitalInputGetValue.vi"("error in (no error)"=w213, "DigitalInputDevRef"=w214) -> ("Value"=w211:bool)  [unwired: 7 in, 2 out]
                n108 = Not(x=w211) -> (.not. x?=w210:bool)
              }
            }
            n109 = call <vilib>:"CTRE_Phoenix_MotorControl_RefNumRegistryGet.vi"("refnum name"="Shooter") -> ("error out"=w190:errorcluster, "PhoenixMotorControlDevRef"=w189:T7)  [unwired: 9 in]
            n110 = call <vilib>:"CTRE_Phoenix_MotorControl_Set.vi"("error in (no error)"=w178, "Output"=0.65, "Control Mode"=w180, "PhoenixMotorControlDevRef"=w179) -> ()  [unwired: 6 in, 2 out]
            n111 = Negate(x="Shooter Speed while intake") -> (-x=w173:dbl)
            n112 = call <vilib>:"CTRE_Phoenix_MotorControl_Set.vi"("error in (no error)"=w190, "Output"=w173, "Control Mode"=w187, "PhoenixMotorControlDevRef"=w189) -> ()  [unwired: 6 in, 2 out]
            n113 = call <vilib>:"CTRE_Phoenix_MotorControl_RefNumRegistryGet.vi"("refnum name"="Mag") -> ("error out"=w170:errorcluster, "PhoenixMotorControlDevRef"=w171:T7)  [unwired: 9 in]
            n114 = call-poly <vilib>:"NT Read Value.vi"("Default Value"=69000.0, "Name"="Encoder") -> ("Numeric"=w168:dbl)  [unwired: 8 in, 1 out]
            n115 = call-poly <vilib>:"CTRE_Phoenix_MotorController_Get_TalonFX.vi"("PhoenixMotorControlDevRef"=w171, "error in"=w170) -> ("Position (Raw Sensor Units)"=w169:i32)  [unwired: 10 in, 3 out]
            n116 = global write "Lime.vi" "Timer Reset"(FALSE ("RPM Good")) -> ()
            n117 = To Long Integer(number=w168) -> (32bit integer=w167:i32)
            n118 = Greater?(x=w169, y=w167) -> (0:w183:bool)
            n119 = Or(x=w183, y=w176) -> (x .or. y?=w166:bool)
            n120 = Select(t=State_Machine."Wait", s=w166, f=State_Machine."Conveyor 2") -> (s? t:f=w184:T3)
          }
          frame "Dash Shoot 1" {
            w218 = T16 0 items=["PercentOutput"=0, "Position"=1, "Velocity"=2, "Current"=3, "Follower"=5, "MotionProfile"=6, "MotionMagic"=7, "MotionProfileArc"=10, "Disabled"=15] ("Control Mode")
            w257 = T16 2 items=["PercentOutput"=0, "Position"=1, "Velocity"=2, "Current"=3, "Follower"=5, "MotionProfile"=6, "MotionMagic"=7, "MotionProfileArc"=10, "Disabled"=15] ("Control Mode")
            n121 = call-poly <vilib>:"NT Read Value.vi"("Default Value"=4550.0, "Name"="RPM") -> ("Numeric"=w235:dbl)  [unwired: 8 in, 1 out]
            n122 = global write "Lime.vi" "Enabled"(TRUE ("Enabled")) -> ()
            n123 = Negate(x=w235) -> (-x=w234:dbl)
            n124 = call <vilib>:"CTRE_Phoenix_MotorControl_RefNumRegistryGet.vi"("refnum name"="Shooter") -> ("error out"=w263:errorcluster, "PhoenixMotorControlDevRef"=w264:T7)  [unwired: 9 in]
            n125 = call <vilib>:"CTRE_Phoenix_MotorControl_ConfigClosedLoopConstants.vi"("PhoenixMotorControlDevRef"=w264, "slotIdx"=3, "P"=0.1, "I"=0.001, "D"=0.0, "error in (no error)"=w263) -> ("PhoenixMotorControlDevRef"=w260:T7, "error out"=w261:errorcluster)  [unwired: 8 in]
            n126 = Multiply(x=3.413, y=w234) -> (x*y=w241:dbl)
            n127 = call <vilib>:"CTRE_Phoenix_MotorControl_SelectProfile Slot.vi"("error in (no error)"=w261, "slotIdx"=3, "PhoenixMotorControlDevRef"=w260) -> ("error out"=w259:errorcluster, "PhoenixMotorControlDevRef"=w258:T7)  [unwired: 7 in]
            n128 = call <vilib>:"CTRE_Phoenix_MotorControl_Set.vi"("error in (no error)"=w259, "Output"=w241, "Control Mode"=w257, "PhoenixMotorControlDevRef"=w258) -> ("error out"=w250:errorcluster, "PhoenixMotorControlDevRef"=w251:T7)  [unwired: 6 in]
            n129 = global write "Lime.vi" "Enabled"(TRUE ("Enabled")) -> ()
            n130 = call-poly <vilib>:"CTRE_Phoenix_MotorController_Get_TalonFX.vi"("PhoenixMotorControlDevRef"=w251, "error in"=w250) -> ("Velocity"=w237:dbl)  [unwired: 9 in, 4 out]
            n131 = disable-structure shown="Disabled" {
              disable-tunnel: [w266 _] -> _
              frame Disabled {
                n132 = call "Elapsed Time"("Time Target (s)"=0.5, "Reset"=FALSE, "Auto Reset"=TRUE, "Set Start Time (s)"=0.0) -> ("Elapsed Time (s)"=→"Present (s)":dbl, "Time has Elapsed"=w266:bool)  [unwired: 8 in, 6 out]
              }
              frame Enabled {
              }
            }
            n133 = call <vilib>:"WPI_JoystickRefNum Registry Get.vi"("refnum name"="Button Board") -> ("error out"=w232:errorcluster, "JoystickDevRef"=w231:T14)  [unwired: 9 in]
            n134 = call <vilib>:"WPI_JoystickGetValues.vi"("error in (no error)"=w232, "JoystickDevRef"=w231) -> ("Buttons"=w230:bool[])  [unwired: 5 in, 4 out]
            n135 = Add(x=w241, y=100.0) -> (x+y=w248:dbl)
            n136 = Subtract(x=w241, y=100.0) -> (x-y=w249:dbl)
            n137 = Index Array(array=w230, index #1=10 ("index"), index #2=0 ("index")) -> (element #1=w226:bool, element #2=w225:bool)
            n138 = In Range and Coerce(upper limit=w248, x=w237, lower limit=w249) -> (In Range?=w217:bool)  [unwired: 1 out]
            n139 = call <vilib>:"CTRE_Phoenix_MotorControl_RefNumRegistryGet.vi"("refnum name"="Mag") -> ("error out"=w244:errorcluster, "PhoenixMotorControlDevRef"=w243:T7)  [unwired: 9 in]
            n140 = And(x=w226, y=w225) -> (x .and. y?=w224:bool)
            n141 = call-poly <vilib>:"CTRE_Phoenix_MotorControl_SetIntegratedSensorPosition_TalonFX_Polymorphic.vi"("error in (no error)"=w244, "New Position"=0.0, "PhoenixMotorControlDevRef"=w243) -> ("error out"=w220:errorcluster, "PhoenixMotorControlDevRef"=w221:T7)  [unwired: 7 in]
            n142 = global write "Lime.vi" "RPM Good"(w217) -> ()
            n143 = And(x=w217, y=w224) -> (x .and. y?=w223:bool)
            n144 = call <vilib>:"CTRE_Phoenix_MotorControl_Set.vi"("error in (no error)"=w220, "Output"=0.0, "Control Mode"=w218, "PhoenixMotorControlDevRef"=w221) -> ()  [unwired: 6 in, 2 out]
            n145 = Select(t=State_Machine."Dash Shoot 2", s=w223, f=State_Machine."Dash Shoot 1") -> (s? t:f=w239:T3)
          }
          frame "Dash Shoot 2" {
            w291 = T16 0 items=["PercentOutput"=0, "Position"=1, "Velocity"=2, "Current"=3, "Follower"=5, "MotionProfile"=6, "MotionMagic"=7, "MotionProfileArc"=10, "Disabled"=15] ("Control Mode")
            w304 = T16 2 items=["PercentOutput"=0, "Position"=1, "Velocity"=2, "Current"=3, "Follower"=5, "MotionProfile"=6, "MotionMagic"=7, "MotionProfileArc"=10, "Disabled"=15] ("Control Mode")
            n146 = disable-structure shown="Disabled" {
              frame Disabled {
                w312 = u32 125 ("milliseconds to wait")
                n147 = Wait (ms)(milliseconds to wait=w312) -> (millisecond timer value=w313:u32)
                n148 = Greater?(x=w313, y=w312) -> ()  [unwired: 1 out]
              }
              frame Enabled {
              }
            }
            n149 = call-poly <vilib>:"NT Read Value.vi"("Default Value"=4550.0, "Name"="RPM") -> ("Numeric"=w286:dbl)  [unwired: 8 in, 1 out]
            n150 = global write "Lime.vi" "Timer Reset"(FALSE ("RPM Good")) -> ()
            n151 = Negate(x=w286) -> (-x=w285:dbl)
            n152 = call <vilib>:"CTRE_Phoenix_MotorControl_RefNumRegistryGet.vi"("refnum name"="Shooter") -> ("error out"=w310:errorcluster, "PhoenixMotorControlDevRef"=w311:T7)  [unwired: 9 in]
            n153 = global write "Lime.vi" "Enabled"(TRUE ("Enabled")) -> ()
            n154 = global read "Lime.vi" "Timer Good"() -> (w273:bool)
            n155 = call <vilib>:"CTRE_Phoenix_MotorControl_ConfigClosedLoopConstants.vi"("PhoenixMotorControlDevRef"=w311, "slotIdx"=3, "P"=0.1, "I"=0.001, "D"=0.0, "error in (no error)"=w310) -> ("PhoenixMotorControlDevRef"=w307:T7, "error out"=w308:errorcluster)  [unwired: 8 in]
            n156 = Multiply(x=3.413, y=w285) -> (x*y=w295:dbl)
            n157 = call <vilib>:"CTRE_Phoenix_MotorControl_SelectProfile Slot.vi"("error in (no error)"=w308, "slotIdx"=3, "PhoenixMotorControlDevRef"=w307) -> ("error out"=w306:errorcluster, "PhoenixMotorControlDevRef"=w305:T7)  [unwired: 7 in]
            n158 = case shown="True" w273 {
              tunnel: [FALSE w315] -> w288
              frame False {
              }
              frame True {
                n159 = disable-structure shown="Disabled" {
                  disable-tunnel: [w320 _] -> _
                  frame Disabled {
                    n160 = call <vilib>:"WPI_DigitalInputRefNum Registry Get.vi"("refnum name"="LS2") -> ("error out"=w327:errorcluster, "DigitalInputDevRef"=w328:T5)  [unwired: 9 in]
                    n161 = call <vilib>:"WPI_DigitalInputRefNum Registry Get.vi"("refnum name"="LS1") -> ("error out"=w323:errorcluster, "DigitalInputDevRef"=w322:T5)  [unwired: 9 in]
                    n162 = call <vilib>:"WPI_DigitalInputGetValue.vi"("error in (no error)"=w327, "DigitalInputDevRef"=w328) -> ("Value"=w325:bool)  [unwired: 7 in, 2 out]
                    n163 = call <vilib>:"WPI_DigitalInputGetValue.vi"("error in (no error)"=w323, "DigitalInputDevRef"=w322) -> ("Value"=w321:bool)  [unwired: 7 in, 2 out]
                    n164 = Or(x=w325, y=w321) -> (x .or. y?=w320:bool)
                  }
                  frame Enabled {
                  }
                }
                n165 = call <vilib>:"WPI_DigitalInputRefNum Registry Get.vi"("refnum name"="Mag Limit") -> ("error out"=w319:errorcluster, "DigitalInputDevRef"=w318:T5)  [unwired: 9 in]
                n166 = call <vilib>:"WPI_DigitalInputGetValue.vi"("error in (no error)"=w319, "DigitalInputDevRef"=w318) -> ("Value"=w316:bool)  [unwired: 7 in, 2 out]
                n167 = Not(x=w316) -> (.not. x?=w315:bool)
              }
            }
            n168 = call <vilib>:"CTRE_Phoenix_MotorControl_Set.vi"("error in (no error)"=w306, "Output"=w295, "Control Mode"=w304, "PhoenixMotorControlDevRef"=w305) -> ()  [unwired: 6 in, 2 out]
            n169 = call <vilib>:"CTRE_Phoenix_MotorControl_RefNumRegistryGet.vi"("refnum name"="Mag") -> ("error out"=w293:errorcluster, "PhoenixMotorControlDevRef"=w292:T7)  [unwired: 9 in]
            n170 = call <vilib>:"CTRE_Phoenix_MotorControl_Set.vi"("error in (no error)"=w293, "Output"=0.9, "Control Mode"=w291, "PhoenixMotorControlDevRef"=w292) -> ()  [unwired: 6 in, 2 out]
            n171 = call <vilib>:"CTRE_Phoenix_MotorControl_RefNumRegistryGet.vi"("refnum name"="Mag") -> ("error out"=w277:errorcluster, "PhoenixMotorControlDevRef"=w278:T7)  [unwired: 9 in]
            n172 = call-poly <vilib>:"CTRE_Phoenix_MotorController_Get_TalonFX.vi"("PhoenixMotorControlDevRef"=w278, "error in"=w277) -> ("Position (Raw Sensor Units)"=w276:i32)  [unwired: 10 in, 3 out]
            n173 = call-poly <vilib>:"NT Read Value.vi"("Default Value"=140000.0, "Name"="Encoder") -> ("Numeric"=w274:dbl)  [unwired: 8 in, 1 out]
            n174 = To Long Integer(number=w274) -> (32bit integer=w275:i32)
            n175 = Greater?(x=w276, y=w275) -> (0:w282:bool)
            n176 = Or(x=w288, y=w282) -> (x .or. y?=w283:bool)
            n177 = Select(t=State_Machine."Wait", s=w283, f=State_Machine."Dash Shoot 2") -> (s? t:f=w296:T3)
          }
          frame "Mag Overcurrent" {
            w340 = T16 0 items=["PercentOutput"=0, "Position"=1, "Velocity"=2, "Current"=3, "Follower"=5, "MotionProfile"=6, "MotionMagic"=7, "MotionProfileArc"=10, "Disabled"=15] ("Control Mode")
            n178 = call <vilib>:"CTRE_Phoenix_MotorControl_RefNumRegistryGet.vi"("refnum name"="Mag") -> ("error out"=w342:errorcluster, "PhoenixMotorControlDevRef"=w341:T7)  [unwired: 9 in]
            n179 = call <vilib>:"CTRE_Phoenix_MotorControl_Set.vi"("error in (no error)"=w342, "Output"=-0.5, "Control Mode"=w340, "PhoenixMotorControlDevRef"=w341) -> ()  [unwired: 6 in, 2 out]
            n180 = call <vilib>:"CTRE_Phoenix_MotorControl_RefNumRegistryGet.vi"("refnum name"="Mag") -> ("error out"=w335:errorcluster, "PhoenixMotorControlDevRef"=w336:T7)  [unwired: 9 in]
            n181 = call-poly <vilib>:"CTRE_Phoenix_MotorController_Get_TalonFX.vi"("PhoenixMotorControlDevRef"=w336, "error in"=w335) -> ("Position"=w334:dbl)  [unwired: 9 in, 4 out]
            n182 = Less Or Equal?(x=w334, y=3000.0) -> (x <= y?=w330:bool)
            n183 = Select(t=State_Machine."Wait", s=w330, f=State_Machine."Mag Overcurrent") -> (s? t:f=w329:T3)
          }
          frame "Low Goal Shoot 1" {
            w381 = T16 2 items=["PercentOutput"=0, "Position"=1, "Velocity"=2, "Current"=3, "Follower"=5, "MotionProfile"=6, "MotionMagic"=7, "MotionProfileArc"=10, "Disabled"=15] ("Control Mode")
            n184 = call-poly <vilib>:"NT Read Value.vi"("Default Value"=900.0, "Name"="OC RPM") -> ("Numeric"=w344:dbl)  [unwired: 8 in, 1 out]
            n185 = Negate(x=w344) -> (-x=w361:dbl)
            n186 = call <vilib>:"CTRE_Phoenix_MotorControl_RefNumRegistryGet.vi"("refnum name"="Shooter") -> ("error out"=w387:errorcluster, "PhoenixMotorControlDevRef"=w388:T7)  [unwired: 9 in]
            n187 = call <vilib>:"CTRE_Phoenix_MotorControl_ConfigClosedLoopConstants.vi"("PhoenixMotorControlDevRef"=w388, "slotIdx"=3, "P"=0.1, "I"=0.001, "D"=0.0, "error in (no error)"=w387) -> ("PhoenixMotorControlDevRef"=w384:T7, "error out"=w385:errorcluster)  [unwired: 8 in]
            n188 = Multiply(x=3.413, y=w361) -> (x*y=w366:dbl)
            n189 = call <vilib>:"CTRE_Phoenix_MotorControl_SelectProfile Slot.vi"("error in (no error)"=w385, "slotIdx"=3, "PhoenixMotorControlDevRef"=w384) -> ("error out"=w383:errorcluster, "PhoenixMotorControlDevRef"=w382:T7)  [unwired: 7 in]
            n190 = call <vilib>:"CTRE_Phoenix_MotorControl_Set.vi"("error in (no error)"=w383, "Output"=w366, "Control Mode"=w381, "PhoenixMotorControlDevRef"=w382) -> ("error out"=w374:errorcluster, "PhoenixMotorControlDevRef"=w375:T7)  [unwired: 6 in]
            n191 = call-poly <vilib>:"CTRE_Phoenix_MotorController_Get_TalonFX.vi"("PhoenixMotorControlDevRef"=w375, "error in"=w374) -> ("Velocity"=w362:dbl)  [unwired: 9 in, 4 out]
            n192 = call <vilib>:"WPI_JoystickRefNum Registry Get.vi"("refnum name"="Button Board") -> ("error out"=w360:errorcluster, "JoystickDevRef"=w359:T14)  [unwired: 9 in]
            n193 = call <vilib>:"WPI_JoystickGetValues.vi"("error in (no error)"=w360, "JoystickDevRef"=w359) -> ("Buttons"=w358:bool[])  [unwired: 5 in, 4 out]
            n194 = Add(x=w366, y=300.0) -> (x+y=w372:dbl)
            n195 = Subtract(x=w366, y=300.0) -> (x-y=w373:dbl)
            n196 = Index Array(array=w358, index #1=3 ("index"), index #2=10 ("index")) -> (element #1=w355:bool, element #2=w354:bool)
            n197 = In Range and Coerce(upper limit=w372, x=w362, lower limit=w373) -> (In Range?=w343:bool)  [unwired: 1 out]
            n198 = call <vilib>:"CTRE_Phoenix_MotorControl_RefNumRegistryGet.vi"("refnum name"="Mag") -> ("error out"=w369:errorcluster, "PhoenixMotorControlDevRef"=w368:T7)  [unwired: 9 in]
            n199 = And(x=w355, y=w354) -> (x .and. y?=w353:bool)
            n200 = call-poly <vilib>:"CTRE_Phoenix_MotorControl_SetIntegratedSensorPosition_TalonFX_Polymorphic.vi"("error in (no error)"=w369, "New Position"=0.0, "PhoenixMotorControlDevRef"=w368) -> ()  [unwired: 7 in, 2 out]
            n201 = global write "Lime.vi" "RPM Good"(w343) -> ()
            n202 = And(x=w343, y=w353) -> (x .and. y?=w363:bool)
            n203 = And(x=w363, y=TRUE) -> (x .and. y?=w352:bool)
            n204 = Select(t=State_Machine."Low Goal Shoot 2", s=w352, f=State_Machine."Low Goal Shoot 1") -> (s? t:f=w349:T3)
          }
          frame "Low Goal Shoot 2" {
            w400 = T16 0 items=["PercentOutput"=0, "Position"=1, "Velocity"=2, "Current"=3, "Follower"=5, "MotionProfile"=6, "MotionMagic"=7, "MotionProfileArc"=10, "Disabled"=15] ("Control Mode")
            w404 = T16 2 items=["PercentOutput"=0, "Position"=1, "Velocity"=2, "Current"=3, "Follower"=5, "MotionProfile"=6, "MotionMagic"=7, "MotionProfileArc"=10, "Disabled"=15] ("Control Mode")
            n205 = global write "Lime.vi" "Timer Reset"(FALSE ("RPM Good")) -> ()
            n206 = call-poly <vilib>:"NT Read Value.vi"("Default Value"=900.0, "Name"="OC RPM") -> ("Numeric"=w391:dbl)  [unwired: 8 in, 1 out]
            n207 = Negate(x=w391) -> (-x=w421:dbl)
            n208 = call <vilib>:"CTRE_Phoenix_MotorControl_RefNumRegistryGet.vi"("refnum name"="Shooter") -> ("error out"=w412:errorcluster, "PhoenixMotorControlDevRef"=w411:T7)  [unwired: 9 in]
            n209 = global read "Lime.vi" "Timer Good"() -> (w390:bool)
            n210 = call <vilib>:"CTRE_Phoenix_MotorControl_ConfigClosedLoopConstants.vi"("PhoenixMotorControlDevRef"=w411, "slotIdx"=3, "P"=0.1, "I"=0.001, "D"=0.0, "error in (no error)"=w412) -> ("PhoenixMotorControlDevRef"=w414:T7, "error out"=w413:errorcluster)  [unwired: 8 in]
            n211 = Multiply(x=3.413, y=w421) -> (x*y=w417:dbl)
            n212 = call <vilib>:"CTRE_Phoenix_MotorControl_SelectProfile Slot.vi"("error in (no error)"=w413, "slotIdx"=3, "PhoenixMotorControlDevRef"=w414) -> ("error out"=w415:errorcluster, "PhoenixMotorControlDevRef"=w416:T7)  [unwired: 7 in]
            n213 = case shown="True" w390 {
              tunnel: [FALSE w429] -> w420
              frame False {
              }
              frame True {
                n214 = call <vilib>:"WPI_DigitalInputRefNum Registry Get.vi"("refnum name"="Mag Limit") -> ("error out"=w433:errorcluster, "DigitalInputDevRef"=w432:T5)  [unwired: 9 in]
                n215 = call <vilib>:"WPI_DigitalInputGetValue.vi"("error in (no error)"=w433, "DigitalInputDevRef"=w432) -> ("Value"=w430:bool)  [unwired: 7 in, 2 out]
                n216 = Not(x=w430) -> (.not. x?=w429:bool)
              }
            }
            n217 = call <vilib>:"CTRE_Phoenix_MotorControl_Set.vi"("error in (no error)"=w415, "Output"=w417, "Control Mode"=w404, "PhoenixMotorControlDevRef"=w416) -> ()  [unwired: 6 in, 2 out]
            n218 = call <vilib>:"CTRE_Phoenix_MotorControl_RefNumRegistryGet.vi"("refnum name"="Mag") -> ("error out"=w418:errorcluster, "PhoenixMotorControlDevRef"=w419:T7)  [unwired: 9 in]
            n219 = call <vilib>:"CTRE_Phoenix_MotorControl_Set.vi"("error in (no error)"=w418, "Output"=0.9, "Control Mode"=w400, "PhoenixMotorControlDevRef"=w419) -> ()  [unwired: 6 in, 2 out]
            n220 = call <vilib>:"CTRE_Phoenix_MotorControl_RefNumRegistryGet.vi"("refnum name"="Mag") -> ("error out"=w423:errorcluster, "PhoenixMotorControlDevRef"=w422:T7)  [unwired: 9 in]
            n221 = call-poly <vilib>:"CTRE_Phoenix_MotorController_Get_TalonFX.vi"("PhoenixMotorControlDevRef"=w422, "error in"=w423) -> ("Position"=w426:dbl)  [unwired: 9 in, 4 out]
            n222 = call-poly <vilib>:"NT Read Value.vi"("Default Value"=140000.0, "Name"="Encoder") -> ("Numeric"=w427:dbl)  [unwired: 8 in, 1 out]
            n223 = Greater?(x=w426, y=w427) -> (0:w425:bool)
            n224 = Or(x=w420, y=w425) -> (x .or. y?=w424:bool)
            n225 = Select(t=State_Machine."Wait", s=w424, f=State_Machine."Low Goal Shoot 2") -> (s? t:f=w396:T3)
          }
          frame "Launch Pad Shoot 1" {
            w451 = T16 2 items=["PercentOutput"=0, "Position"=1, "Velocity"=2, "Current"=3, "Follower"=5, "MotionProfile"=6, "MotionMagic"=7, "MotionProfileArc"=10, "Disabled"=15] ("Control Mode")
            n226 = call-poly <vilib>:"NT Read Value.vi"("Default Value"=3900.0, "Name"="LP RPM") -> ("Numeric"=w436:dbl)  [unwired: 8 in, 1 out]
            n227 = Negate(x=w436) -> (-x=w473:dbl)
            n228 = call <vilib>:"CTRE_Phoenix_MotorControl_RefNumRegistryGet.vi"("refnum name"="Shooter") -> ("error out"=w459:errorcluster, "PhoenixMotorControlDevRef"=w458:T7)  [unwired: 9 in]
            n229 = call <vilib>:"WPI_JoystickRefNum Registry Get.vi"("refnum name"="Button Board") -> ("error out"=w474:errorcluster, "JoystickDevRef"=w475:T14)  [unwired: 9 in]
            n230 = call <vilib>:"CTRE_Phoenix_MotorControl_ConfigClosedLoopConstants.vi"("PhoenixMotorControlDevRef"=w458, "slotIdx"=3, "P"=0.1, "I"=0.001, "D"=0.0, "error in (no error)"=w459) -> ("PhoenixMotorControlDevRef"=w461:T7, "error out"=w460:errorcluster)  [unwired: 8 in]
            n231 = Multiply(x=3.413, y=w473) -> (x*y=w470:dbl)
            n232 = call <vilib>:"CTRE_Phoenix_MotorControl_SelectProfile Slot.vi"("error in (no error)"=w460, "slotIdx"=3, "PhoenixMotorControlDevRef"=w461) -> ("error out"=w462:errorcluster, "PhoenixMotorControlDevRef"=w463:T7)  [unwired: 7 in]
            n233 = call <vilib>:"WPI_JoystickGetValues.vi"("error in (no error)"=w474, "JoystickDevRef"=w475) -> ("Buttons"=w476:bool[])  [unwired: 5 in, 4 out]
            n234 = global write "Lime.vi" "Enabled"(TRUE ("Enabled")) -> ()
            n235 = call <vilib>:"CTRE_Phoenix_MotorControl_Set.vi"("error in (no error)"=w462, "Output"=w470, "Control Mode"=w451, "PhoenixMotorControlDevRef"=w463) -> ("error out"=w465:errorcluster, "PhoenixMotorControlDevRef"=w464:T7)  [unwired: 6 in]
            n236 = Add(x=w470, y=100.0) -> (x+y=w467:dbl)
            n237 = Index Array(array=w476, index #1=10 ("index"), index #2=6 ("index")) -> (element #1=w477:bool, element #2=w478:bool)
            n238 = call-poly <vilib>:"CTRE_Phoenix_MotorController_Get_TalonFX.vi"("PhoenixMotorControlDevRef"=w464, "error in"=w465) -> ("Velocity"=w472:dbl)  [unwired: 9 in, 4 out]
            n239 = Subtract(x=w470, y=100.0) -> (x-y=w466:dbl)
            n240 = And(x=w477, y=w478) -> (x .and. y?=w479:bool)
            n241 = In Range and Coerce(upper limit=w467, x=w472, lower limit=w466) -> (In Range?=w435:bool)  [unwired: 1 out]
            n242 = And(x=w435, y=w479) -> (x .and. y?=w471:bool)
            n243 = global write "Lime.vi" "RPM Good"(w435) -> ()
            n244 = And(x=w471, y=TRUE) -> (x .and. y?=w480:bool)
            n245 = Select(t=State_Machine."Launch Pad Shoot 2", s=w480, f=State_Machine."Launch Pad Shoot 1") -> (s? t:f=w441:T3)
            n246 = call <vilib>:"CTRE_Phoenix_MotorControl_RefNumRegistryGet.vi"("refnum name"="Mag") -> ("error out"=w468:errorcluster, "PhoenixMotorControlDevRef"=w469:T7)  [unwired: 9 in]
            n247 = call-poly <vilib>:"CTRE_Phoenix_MotorControl_SetIntegratedSensorPosition_TalonFX_Polymorphic.vi"("error in (no error)"=w468, "New Position"=0.0, "PhoenixMotorControlDevRef"=w469) -> ()  [unwired: 7 in, 2 out]
          }
          frame "Launch Pad Shoot 2" {
            w493 = T16 0 items=["PercentOutput"=0, "Position"=1, "Velocity"=2, "Current"=3, "Follower"=5, "MotionProfile"=6, "MotionMagic"=7, "MotionProfileArc"=10, "Disabled"=15] ("Control Mode")
            w497 = T16 2 items=["PercentOutput"=0, "Position"=1, "Velocity"=2, "Current"=3, "Follower"=5, "MotionProfile"=6, "MotionMagic"=7, "MotionProfileArc"=10, "Disabled"=15] ("Control Mode")
            n248 = disable-structure shown="Disabled" {
              frame Disabled {
                w521 = u32 125 ("milliseconds to wait")
                n249 = Wait (ms)(milliseconds to wait=w521) -> (millisecond timer value=w522:u32)
                n250 = Greater?(x=w522, y=w521) -> ()  [unwired: 1 out]
              }
              frame Enabled {
              }
            }
            n251 = call-poly <vilib>:"NT Read Value.vi"("Default Value"=3900.0, "Name"="LP RPM") -> ("Numeric"=w486:dbl)  [unwired: 8 in, 1 out]
            n252 = global write "Lime.vi" "Timer Reset"(FALSE ("RPM Good")) -> ()
            n253 = Negate(x=w486) -> (-x=w514:dbl)
            n254 = call <vilib>:"CTRE_Phoenix_MotorControl_RefNumRegistryGet.vi"("refnum name"="Shooter") -> ("error out"=w505:errorcluster, "PhoenixMotorControlDevRef"=w504:T7)  [unwired: 9 in]
            n255 = global read "Lime.vi" "Timer Good"() -> (w483:bool)
            n256 = call <vilib>:"CTRE_Phoenix_MotorControl_ConfigClosedLoopConstants.vi"("PhoenixMotorControlDevRef"=w504, "slotIdx"=3, "P"=0.1, "I"=0.001, "D"=0.0, "error in (no error)"=w505) -> ("PhoenixMotorControlDevRef"=w507:T7, "error out"=w506:errorcluster)  [unwired: 8 in]
            n257 = Multiply(x=3.413, y=w514) -> (x*y=w510:dbl)
            n258 = call <vilib>:"CTRE_Phoenix_MotorControl_SelectProfile Slot.vi"("error in (no error)"=w506, "slotIdx"=3, "PhoenixMotorControlDevRef"=w507) -> ("error out"=w508:errorcluster, "PhoenixMotorControlDevRef"=w509:T7)  [unwired: 7 in]
            n259 = case shown="True" w483 {
              tunnel: [FALSE w524] -> w513
              frame False {
              }
              frame True {
                n260 = call <vilib>:"WPI_DigitalInputRefNum Registry Get.vi"("refnum name"="Mag Limit") -> ("error out"=w528:errorcluster, "DigitalInputDevRef"=w527:T5)  [unwired: 9 in]
                n261 = call <vilib>:"WPI_DigitalInputGetValue.vi"("error in (no error)"=w528, "DigitalInputDevRef"=w527) -> ("Value"=w525:bool)  [unwired: 7 in, 2 out]
                n262 = Not(x=w525) -> (.not. x?=w524:bool)
              }
            }
            n263 = call <vilib>:"CTRE_Phoenix_MotorControl_Set.vi"("error in (no error)"=w508, "Output"=w510, "Control Mode"=w497, "PhoenixMotorControlDevRef"=w509) -> ()  [unwired: 6 in, 2 out]
            n264 = global write "Lime.vi" "Enabled"(TRUE ("Enabled")) -> ()
            n265 = call <vilib>:"CTRE_Phoenix_MotorControl_RefNumRegistryGet.vi"("refnum name"="Mag") -> ("error out"=w511:errorcluster, "PhoenixMotorControlDevRef"=w512:T7)  [unwired: 9 in]
            n266 = call <vilib>:"CTRE_Phoenix_MotorControl_Set.vi"("error in (no error)"=w511, "Output"=0.9, "Control Mode"=w493, "PhoenixMotorControlDevRef"=w512) -> ()  [unwired: 6 in, 2 out]
            n267 = call <vilib>:"CTRE_Phoenix_MotorControl_RefNumRegistryGet.vi"("refnum name"="Mag") -> ("error out"=w516:errorcluster, "PhoenixMotorControlDevRef"=w515:T7)  [unwired: 9 in]
            n268 = call-poly <vilib>:"CTRE_Phoenix_MotorController_Get_TalonFX.vi"("PhoenixMotorControlDevRef"=w515, "error in"=w516) -> ("Position"=w519:dbl)  [unwired: 9 in, 4 out]
            n269 = call-poly <vilib>:"NT Read Value.vi"("Default Value"=140000.0, "Name"="Encoder") -> ("Numeric"=w520:dbl)  [unwired: 8 in, 1 out]
            n270 = Greater?(x=w519, y=w520) -> (0:w518:bool)
            n271 = Or(x=w513, y=w518) -> (x .or. y?=w517:bool)
            n272 = Select(t=State_Machine."Wait", s=w517, f=State_Machine."Launch Pad Shoot 2") -> (s? t:f=w489:T3)
          }
          frame "Wall Shoot 1" {
            w535 = T16 0 items=["PercentOutput"=0, "Position"=1, "Velocity"=2, "Current"=3, "Follower"=5, "MotionProfile"=6, "MotionMagic"=7, "MotionProfileArc"=10, "Disabled"=15] ("Control Mode")
            w570 = T16 2 items=["PercentOutput"=0, "Position"=1, "Velocity"=2, "Current"=3, "Follower"=5, "MotionProfile"=6, "MotionMagic"=7, "MotionProfileArc"=10, "Disabled"=15] ("Control Mode")
            n273 = call-poly <vilib>:"NT Read Value.vi"("Default Value"=3500.0, "Name"="WS RPM") -> ("Numeric"=w529:dbl)  [unwired: 8 in, 1 out]
            n274 = Negate(x=w529) -> (-x=w550:dbl)
            n275 = call <vilib>:"CTRE_Phoenix_MotorControl_RefNumRegistryGet.vi"("refnum name"="Shooter") -> ("error out"=w576:errorcluster, "PhoenixMotorControlDevRef"=w577:T7)  [unwired: 9 in]
            n276 = call <vilib>:"CTRE_Phoenix_MotorControl_ConfigClosedLoopConstants.vi"("PhoenixMotorControlDevRef"=w577, "slotIdx"=3, "P"=0.1, "I"=0.001, "D"=0.0, "error in (no error)"=w576) -> ("PhoenixMotorControlDevRef"=w573:T7, "error out"=w574:errorcluster)  [unwired: 8 in]
            n277 = Multiply(x=3.413, y=w550) -> (x*y=w554:dbl)
            n278 = call <vilib>:"CTRE_Phoenix_MotorControl_SelectProfile Slot.vi"("error in (no error)"=w574, "slotIdx"=3, "PhoenixMotorControlDevRef"=w573) -> ("error out"=w572:errorcluster, "PhoenixMotorControlDevRef"=w571:T7)  [unwired: 7 in]
            n279 = call <vilib>:"CTRE_Phoenix_MotorControl_Set.vi"("error in (no error)"=w572, "Output"=w554, "Control Mode"=w570, "PhoenixMotorControlDevRef"=w571) -> ("error out"=w563:errorcluster, "PhoenixMotorControlDevRef"=w564:T7)  [unwired: 6 in]
            n280 = call-poly <vilib>:"CTRE_Phoenix_MotorController_Get_TalonFX.vi"("PhoenixMotorControlDevRef"=w564, "error in"=w563) -> ("Velocity"=w551:dbl)  [unwired: 9 in, 4 out]
            n281 = global write "Lime.vi" "Enabled"(TRUE ("Enabled")) -> ()
            n282 = call <vilib>:"WPI_JoystickRefNum Registry Get.vi"("refnum name"="Button Board") -> ("error out"=w549:errorcluster, "JoystickDevRef"=w548:T14)  [unwired: 9 in]
            n283 = call <vilib>:"WPI_JoystickGetValues.vi"("error in (no error)"=w549, "JoystickDevRef"=w548) -> ("Buttons"=w547:bool[])  [unwired: 5 in, 4 out]
            n284 = Add(x=w554, y=150.0) -> (x+y=w561:dbl)
            n285 = Subtract(x=w554, y=150.0) -> (x-y=w562:dbl)
            n286 = Index Array(array=w547, index #1=1 ("index"), index #2=10 ("index")) -> (element #1=w543:bool, element #2=w542:bool)
            n287 = In Range and Coerce(upper limit=w561, x=w551, lower limit=w562) -> (In Range?=w534:bool)  [unwired: 1 out]
            n288 = call <vilib>:"CTRE_Phoenix_MotorControl_RefNumRegistryGet.vi"("refnum name"="Mag") -> ("error out"=w557:errorcluster, "PhoenixMotorControlDevRef"=w556:T7)  [unwired: 9 in]
            n289 = And(x=w543, y=w542) -> (x .and. y?=w541:bool)
            n290 = call-poly <vilib>:"CTRE_Phoenix_MotorControl_SetIntegratedSensorPosition_TalonFX_Polymorphic.vi"("error in (no error)"=w557, "New Position"=0.0, "PhoenixMotorControlDevRef"=w556) -> ("error out"=w537:errorcluster, "PhoenixMotorControlDevRef"=w538:T7)  [unwired: 7 in]
            n291 = global write "Lime.vi" "RPM Good"(w534) -> ()
            n292 = And(x=w534, y=w541) -> (x .and. y?=w540:bool)
            n293 = call <vilib>:"CTRE_Phoenix_MotorControl_Set.vi"("error in (no error)"=w537, "Output"=0.0, "Control Mode"=w535, "PhoenixMotorControlDevRef"=w538) -> ()  [unwired: 6 in, 2 out]
            n294 = Select(t=State_Machine."Wall Shoot 2", s=w540, f=State_Machine."Wall Shoot 1") -> (s? t:f=w533:T3)
          }
          frame "Wall Shoot 2" {
            w599 = T16 0 items=["PercentOutput"=0, "Position"=1, "Velocity"=2, "Current"=3, "Follower"=5, "MotionProfile"=6, "MotionMagic"=7, "MotionProfileArc"=10, "Disabled"=15] ("Control Mode")
            w611 = T16 2 items=["PercentOutput"=0, "Position"=1, "Velocity"=2, "Current"=3, "Follower"=5, "MotionProfile"=6, "MotionMagic"=7, "MotionProfileArc"=10, "Disabled"=15] ("Control Mode")
            n295 = call-poly <vilib>:"NT Read Value.vi"("Default Value"=3500.0, "Name"="WS RPM") -> ("Numeric"=w578:dbl)  [unwired: 8 in, 1 out]
            n296 = global write "Lime.vi" "Timer Reset"(FALSE ("RPM Good")) -> ()
            n297 = Negate(x=w578) -> (-x=w595:dbl)
            n298 = call <vilib>:"CTRE_Phoenix_MotorControl_RefNumRegistryGet.vi"("refnum name"="Shooter") -> ("error out"=w617:errorcluster, "PhoenixMotorControlDevRef"=w618:T7)  [unwired: 9 in]
            n299 = global read "Lime.vi" "Timer Good"() -> (w584:bool)
            n300 = call <vilib>:"CTRE_Phoenix_MotorControl_ConfigClosedLoopConstants.vi"("PhoenixMotorControlDevRef"=w618, "slotIdx"=3, "P"=0.1, "I"=0.001, "D"=0.0, "error in (no error)"=w617) -> ("PhoenixMotorControlDevRef"=w614:T7, "error out"=w615:errorcluster)  [unwired: 8 in]
            n301 = Multiply(x=3.413, y=w595) -> (x*y=w603:dbl)
            n302 = call <vilib>:"CTRE_Phoenix_MotorControl_SelectProfile Slot.vi"("error in (no error)"=w615, "slotIdx"=3, "PhoenixMotorControlDevRef"=w614) -> ("error out"=w613:errorcluster, "PhoenixMotorControlDevRef"=w612:T7)  [unwired: 7 in]
            n303 = case shown="True" w584 {
              tunnel: [FALSE w620] -> w596
              frame False {
              }
              frame True {
                n304 = disable-structure shown="Disabled" {
                  disable-tunnel: [w625 _] -> _
                  frame Disabled {
                    n305 = call <vilib>:"WPI_DigitalInputRefNum Registry Get.vi"("refnum name"="LS2") -> ("error out"=w632:errorcluster, "DigitalInputDevRef"=w633:T5)  [unwired: 9 in]
                    n306 = call <vilib>:"WPI_DigitalInputRefNum Registry Get.vi"("refnum name"="LS1") -> ("error out"=w628:errorcluster, "DigitalInputDevRef"=w627:T5)  [unwired: 9 in]
                    n307 = call <vilib>:"WPI_DigitalInputGetValue.vi"("error in (no error)"=w632, "DigitalInputDevRef"=w633) -> ("Value"=w630:bool)  [unwired: 7 in, 2 out]
                    n308 = call <vilib>:"WPI_DigitalInputGetValue.vi"("error in (no error)"=w628, "DigitalInputDevRef"=w627) -> ("Value"=w626:bool)  [unwired: 7 in, 2 out]
                    n309 = Or(x=w630, y=w626) -> (x .or. y?=w625:bool)
                  }
                  frame Enabled {
                  }
                }
                n310 = call <vilib>:"WPI_DigitalInputRefNum Registry Get.vi"("refnum name"="Mag Limit") -> ("error out"=w624:errorcluster, "DigitalInputDevRef"=w623:T5)  [unwired: 9 in]
                n311 = call <vilib>:"WPI_DigitalInputGetValue.vi"("error in (no error)"=w624, "DigitalInputDevRef"=w623) -> ("Value"=w621:bool)  [unwired: 7 in, 2 out]
                n312 = Not(x=w621) -> (.not. x?=w620:bool)
              }
            }
            n313 = call <vilib>:"CTRE_Phoenix_MotorControl_Set.vi"("error in (no error)"=w613, "Output"=w603, "Control Mode"=w611, "PhoenixMotorControlDevRef"=w612) -> ()  [unwired: 6 in, 2 out]
            n314 = global write "Lime.vi" "Enabled"(TRUE ("Enabled")) -> ()
            n315 = call <vilib>:"CTRE_Phoenix_MotorControl_RefNumRegistryGet.vi"("refnum name"="Mag") -> ("error out"=w601:errorcluster, "PhoenixMotorControlDevRef"=w600:T7)  [unwired: 9 in]
            n316 = call <vilib>:"CTRE_Phoenix_MotorControl_Set.vi"("error in (no error)"=w601, "Output"=0.9, "Control Mode"=w599, "PhoenixMotorControlDevRef"=w600) -> ()  [unwired: 6 in, 2 out]
            n317 = call <vilib>:"CTRE_Phoenix_MotorControl_RefNumRegistryGet.vi"("refnum name"="Mag") -> ("error out"=w588:errorcluster, "PhoenixMotorControlDevRef"=w589:T7)  [unwired: 9 in]
            n318 = call-poly <vilib>:"CTRE_Phoenix_MotorController_Get_TalonFX.vi"("PhoenixMotorControlDevRef"=w589, "error in"=w588) -> ("Position (Raw Sensor Units)"=w587:i32)  [unwired: 10 in, 3 out]
            n319 = call-poly <vilib>:"NT Read Value.vi"("Default Value"=140000.0, "Name"="Encoder") -> ("Numeric"=w585:dbl)  [unwired: 8 in, 1 out]
            n320 = To Long Integer(number=w585) -> (32bit integer=w586:i32)
            n321 = Greater?(x=w587, y=w586) -> (0:w593:bool)
            n322 = Or(x=w596, y=w593) -> (x .or. y?=w594:bool)
            n323 = Select(t=State_Machine."Wait", s=w594, f=State_Machine."Wall Shoot 2") -> (s? t:f=w583:T3)
          }
        }
      }
      frame True {
      }
    }
  }
  n324 = while {
    stop <- FALSE stop-if-true
    n325 = call-poly <vilib>:"NT Read Value.vi"("Name"="/limelight-shoot/ty") -> ("Numeric"=w652:dbl)  [unwired: 9 in, 1 out]
    n326 = global write "Lime.vi" "Rotate Error"(w652) -> ()
    n327 = call-poly <vilib>:"NT Read Value.vi"("Name"="/limelight-shoot/tx") -> ("Numeric"=w656:dbl)  [unwired: 9 in, 1 out]
    n328 = call-poly <vilib>:"NT Read Value.vi"("Name"="/limelight-intake/ty") -> ("Numeric"=w662:dbl)  [unwired: 9 in, 1 out]
    n329 = Absolute Value(x=w652) -> (abs(x)=w715:dbl)
    n330 = Sign(1:w652) -> (0:w710:dbl)
    n331 = Absolute Value(x=w656) -> (abs(x)=w694:dbl)
    n332 = Sign(1:w656) -> (0:w689:dbl)
    n333 = Absolute Value(x=w662) -> (abs(x)=w677:dbl)
    n334 = Sign(1:w662) -> (0:w671:dbl)
    n335 = Multiply(x=w662, y="Steering K 3") -> (x*y=w669:dbl)
    n336 = global write "Lime.vi" "Side F/B Error"(w662) -> ()
    n337 = Subtract(x=w715, y="Aim Deadband") -> (x-y=w716:dbl)
    n338 = Multiply(x=w652, y="Steering K 2") -> (x*y=w708:dbl)
    n339 = Subtract(x=w677, y="Aim Deadband 2") -> (x-y=w678:dbl)
    n340 = Multiply(x="Min Steer 2", y=w671) -> (x*y=w670:dbl)
    n341 = Subtract(x=w694, y="Aim Deadband 3") -> (x-y=w695:dbl)
    n342 = Multiply(x=w656, y="Steering K 4") -> (x*y=w687:dbl)
    n343 = Less Than 0?(x=w678) -> (x < 0?=w675:bool)
    n344 = Add(x=w670, y=w669) -> (x+y=w668:dbl)
    n345 = Multiply(x="Min Steer", y=w710) -> (x*y=w709:dbl)
    n346 = Less Than 0?(x=w695) -> (x < 0?=w693:bool)
    n347 = Multiply(x="Min Steer 3", y=w689) -> (x*y=w688:dbl)
    n348 = Less Than 0?(x=w716) -> (x < 0?=w714:bool)
    n349 = Add(x=w709, y=w708) -> (x+y=w707:dbl)
    n350 = Select(t=0.0, s=w675, f=w668) -> (s? t:f=w667:dbl)
    n351 = Add(x=w688, y=w687) -> (x+y=w686:dbl)
    n352 = Select(t=0.0, s=w714, f=w707) -> (s? t:f=w706:dbl)
    n353 = Select(t=0.0, s=w693, f=w686) -> (s? t:f=w685:dbl)
    n354 = Multiply(x=w667, y=0.5) -> (x*y=w665:dbl)
    n355 = Multiply(x=w706, y=0.5) -> (x*y=w704:dbl)
    n356 = Multiply(x=w685, y=0.5) -> (x*y=w683:dbl)
    n357 = Multiply(x=0.7, y=w665) -> (x*y=w663:dbl)
    n358 = global write "Lime.vi" "Side F/B Drive"(w663) -> ()
    n359 = Multiply(x=0.7, y=w704) -> (x*y=w702:dbl)
    n360 = Multiply(x=-0.7, y=w683) -> (x*y=w681:dbl)
    n361 = global write "Lime.vi" "Rotate"(w702) -> ()
    n362 = global write "Lime.vi" "F/B Drive"(w681) -> ()
    n363 = call <vilib>:"WPI_DriverStationGetModeAndStatus.vi"() -> ("Robot Mode"=w651:T13)  [unwired: 10 in, 1 out]
    n364 = call <vilib>:"WPI_DriverStationGetModeAndStatus.vi"() -> ("Robot Mode"=w649:T13)  [unwired: 10 in, 1 out]
    n365 = global read "Lime.vi" "Enabled"() -> (w645:bool)
    n366 = Equal?(x=w651, y=WPI_DriverStationRobotMode2."Autonomous Enabled") -> (x = y?=w647:bool)
    n367 = Equal?(x=w649, y=WPI_DriverStationRobotMode2."Autonomous Disabled") -> (x = y?=w646:bool)
    n368 = global read "Lime.vi" "Enabled"() -> (w641:bool)
    n369 = Not(x=w645) -> (.not. x?=w643:bool)
    n370 = Or(x=w647, y=w646) -> (x .or. y?=w642:bool)
    n371 = call-poly <vilib>:"NT Read Value.vi"("Name"="Limelight On") -> ("Boolean"=w639:bool)  [unwired: 9 in, 1 out]
    n372 = call <vilib>:"WPI_DriverStationGet Alliance Info.vi"() -> ("Alliance"=w637:T17)  [unwired: 6 in, 5 out]
    n373 = And(x=w642, y=w643) -> (x .and. y?=w644:bool)
    n374 = global read "Lime.vi" "Shooter Pipeline"() -> (w654:dbl)
    n375 = And(x=w641, y=w639) -> (x .and. y?=w640:bool)
    n376 = case shown="False" w640 {
      tunnel: [1.0 ("Numeric") 3.0 ("Numeric")] -> w699
      tunnel: [1.0 ("Numeric") 0.0 ("Numeric")] -> w697
      frame False {
      }
      frame True {
      }
    }
    n377 = Equal?(x=WPI_DriverStationAllianceInfo."Red", y=w637) -> (x = y?=w636:bool)
    n378 = case shown="True" w644 {
      tunnel: [1.0 ("Numeric") 0.0 ("Numeric")] -> w660
      tunnel: [1.0 ("Numeric") 0.0 ("Numeric")] -> w658
      frame False {
      }
      frame True {
      }
    }
    n379 = case shown="False" w636 {
      tunnel: [0.0 ("Numeric") 1.0 ("Numeric")] -> w653
      frame False {
      }
      frame True {
      }
    }
    n380 = call "NT Write Number_On Change.vi"("Numeric"=w699, "Name"="/limelight-shoot/ledMode") -> ()  [unwired: 9 in, 1 out]
    n381 = call "NT Write Number_On Change.vi"("Numeric"=w697, "Name"="/limelight-shoot/camMode") -> ()  [unwired: 9 in, 1 out]
    n382 = call "NT Write Number_On Change.vi"("Numeric"=w653, "Name"="/limelight-intake/pipeline") -> ()  [unwired: 9 in, 1 out]
    n383 = call "NT Write Number_On Change.vi"("Numeric"=w654, "Name"="/limelight-shoot/pipeline") -> ()  [unwired: 9 in, 1 out]
    n384 = call "NT Write Number_On Change.vi"("Numeric"=w660, "Name"="/limelight-intake/ledMode") -> ()  [unwired: 9 in, 1 out]
    n385 = call "NT Write Number_On Change.vi"("Numeric"=w658, "Name"="/limelight-intake/camMode") -> ()  [unwired: 9 in, 1 out]
    n386 = Wait (ms)(milliseconds to wait=u32 150) -> ()  [unwired: 1 out]
  }
  n387 = while {
    shift-right: [w739] -> _
    shift-left: Auto_State_Machine."Cam Swap 1" -> [w740]
    stop <- FALSE stop-if-true
    n388 = call <vilib>:"WPI_DriverStationGetModeAndStatus.vi"() -> ("Robot Mode"=w737:T13)  [unwired: 10 in, 1 out]
    n389 = call <vilib>:"WPI_DriverStationGetModeAndStatus.vi"() -> ("Robot Mode"=w735:T13)  [unwired: 10 in, 1 out]
    n390 = Wait (ms)(milliseconds to wait=u32 150) -> ()  [unwired: 1 out]
    n391 = Equal?(x=w737, y=WPI_DriverStationRobotMode2."Autonomous Enabled") -> (x = y?=w733:bool)
    n392 = Equal?(x=w735, y=WPI_DriverStationRobotMode2."Autonomous Disabled") -> (x = y?=w732:bool)
    n393 = Or(x=w733, y=w732) -> (x .or. y?=w731:bool)
    n394 = case shown="True" w731 {
      tunnel: w740 -> [_ w743]
      tunnel: [Auto_State_Machine."Cam Swap 1" w742] -> w739
      frame False {
      }
      frame True {
        n395 = case shown="\"OC Reverse\"" w743 {
          tunnel: [w765 w799 w839 w890 w947 w958 w962 w974 w1015 w1093 w1112 w1205 w1258 w1315 w1373 w1428 w1503 w1564 w1620 Auto_State_Machine."Stop"] -> w742
          frame "Auto Wait", Default {
            w785 = T16 0 items=["PercentOutput"=0, "Position"=1, "Velocity"=2, "Current"=3, "Follower"=5, "MotionProfile"=6, "MotionMagic"=7, "MotionProfileArc"=10, "Disabled"=15] ("Control Mode")
            w789 = T16 0 items=["PercentOutput"=0, "Position"=1, "Velocity"=2, "Current"=3, "Follower"=5, "MotionProfile"=6, "MotionMagic"=7, "MotionProfileArc"=10, "Disabled"=15] ("Control Mode")
            n396 = global write "Lime.vi" "Timer Reset"(TRUE ("RPM Good")) -> ()
            n397 = global write "Lime.vi" "Shooter Pipeline"(0.0 ("Shooter Pipeline")) -> ()
            n398 = global write "Lime.vi" "Enabled"(FALSE ("Enabled")) -> ()
            n399 = call <vilib>:"WPI_SolenoidRefNum Registry Get.vi"("refnum name"="Intake") -> ("error out"=w760:errorcluster, "SolenoidDevRef"=w759:T19)  [unwired: 9 in]
            n400 = call <vilib>:"CTRE_Phoenix_MotorControl_RefNumRegistryGet.vi"("refnum name"="Shooter") -> ("error out"=w787:errorcluster, "PhoenixMotorControlDevRef"=w786:T7)  [unwired: 9 in]
            n401 = call-poly <vilib>:"WPI_SolenoidSet.vi"("error in (no error)"=w760, "Value"=WPI_SolenoidValue."Reverse", "SolenoidDevRef"=w759) -> ()  [unwired: 7 in, 2 out]
            n402 = call <vilib>:"CTRE_Phoenix_MotorControl_Set.vi"("error in (no error)"=w787, "Output"=0.0, "Control Mode"=w785, "PhoenixMotorControlDevRef"=w786) -> ()  [unwired: 6 in, 2 out]
            n403 = call <vilib>:"CTRE_Phoenix_MotorControl_RefNumRegistryGet.vi"("refnum name"="Mag") -> ("error out"=w791:errorcluster, "PhoenixMotorControlDevRef"=w790:T7)  [unwired: 9 in]
            n404 = call <vilib>:"CTRE_Phoenix_MotorControl_Set.vi"("error in (no error)"=w791, "Output"=0.0, "Control Mode"=w789, "PhoenixMotorControlDevRef"=w790) -> ()  [unwired: 6 in, 2 out]
            n405 = call <vilib>:"CTRE_PigeonIMU_RefNumRegistryGet.vi"("refnum name"="Pigeon") -> ("error out"=w772:errorcluster, "PigeonIMUDevRef"=w773:T11)  [unwired: 9 in]
            n406 = call-poly <vilib>:"NT Read Value.vi"("Name"="Auto Choice") -> ("String"=w747:string)  [unwired: 9 in, 1 out]
            n407 = call <vilib>:"CTRE_PigeonIMU_SetYaw.vi"("error in (no error)"=w772, "Value"=0.0, "PigeonIMUDevRef"=w773) -> ()  [unwired: 7 in, 2 out]
            n408 = call <vilib>:"WPI_RobotDriveRefNum Registry Get.vi"("refnum name"="Craig") -> ("error out"=w780:errorcluster, "RobotDriveDevRef"=w781:T21)  [unwired: 9 in]
            n409 = Equal?(x=w747, y="1+1 Auto") -> (x = y?=w744:bool)
            n410 = call-poly <vilib>:"WPI_RobotDriveHolonomicDrive.vi"("Rotation"=0.0, "error in (no error)"=w780, "Y"=0.0, "X"=0.0, "RobotDriveDevRef"=w781) -> ()  [unwired: 4 in, 3 out]
            n411 = Wait (ms)(milliseconds to wait=u32 150) -> ()  [unwired: 1 out]
            n412 = call <vilib>:"WPI_DriverStationGet Alliance Info.vi"() -> ("Alliance"=w750:T17)  [unwired: 6 in, 5 out]
            n413 = Equal?(x=WPI_DriverStationAllianceInfo."Red", y=w750) -> (x = y?=w749:bool)
            n414 = case shown="False" w749 {
              tunnel: [0.0 ("Numeric") 1.0 ("Numeric")] -> w751
              frame False {
              }
              frame True {
              }
            }
            n415 = Select(t=Auto_State_Machine."Shoot OC 1", s=TRUE, f=Auto_State_Machine."Auto Wait") -> (s? t:f=w774:T2)
            n416 = call <vilib>:"WPI_DriverStationGetModeAndStatus.vi"() -> ("Robot Mode"=w764:T13)  [unwired: 10 in, 1 out]
            n417 = Select(t=Auto_State_Machine."Go To Ball", s=w744, f=w774) -> (s? t:f=w767:T2)
            n418 = Equal?(x=w764, y=WPI_DriverStationRobotMode2."Autonomous Enabled") -> (x = y?=w762:bool)
            n419 = call "NT Write Number_On Change.vi"("Numeric"=w751, "Name"="/limelight-intake/pipeline") -> ()  [unwired: 9 in, 1 out]
            n420 = Not(x=w762) -> (.not. x?=w761:bool)
            n421 = Select(t=Auto_State_Machine."Auto Wait", s=w761, f=w767) -> (s? t:f=w765:T2)
          }
          frame "Shoot OC 1" {
            w823 = T16 2 items=["PercentOutput"=0, "Position"=1, "Velocity"=2, "Current"=3, "Follower"=5, "MotionProfile"=6, "MotionMagic"=7, "MotionProfileArc"=10, "Disabled"=15] ("Control Mode")
            n422 = Negate(x="Auto On Contact RPM") -> (-x=w803:dbl)
            n423 = call <vilib>:"CTRE_Phoenix_MotorControl_RefNumRegistryGet.vi"("refnum name"="Shooter") -> ("error out"=w829:errorcluster, "PhoenixMotorControlDevRef"=w830:T7)  [unwired: 9 in]
            n424 = call <vilib>:"CTRE_Phoenix_MotorControl_ConfigClosedLoopConstants.vi"("PhoenixMotorControlDevRef"=w830, "slotIdx"=3, "P"=0.1, "I"=0.001, "D"=0.0, "error in (no error)"=w829) -> ("PhoenixMotorControlDevRef"=w826:T7, "error out"=w827:errorcluster)  [unwired: 8 in]
            n425 = Multiply(x=3.413, y=w803) -> (x*y=w808:dbl)
            n426 = call <vilib>:"CTRE_Phoenix_MotorControl_SelectProfile Slot.vi"("error in (no error)"=w827, "slotIdx"=3, "PhoenixMotorControlDevRef"=w826) -> ("error out"=w825:errorcluster, "PhoenixMotorControlDevRef"=w824:T7)  [unwired: 7 in]
            n427 = call <vilib>:"WPI_SolenoidRefNum Registry Get.vi"("refnum name"="Intake") -> ("error out"=w798:errorcluster, "SolenoidDevRef"=w797:T19)  [unwired: 9 in]
            n428 = call <vilib>:"CTRE_Phoenix_MotorControl_Set.vi"("error in (no error)"=w825, "Output"=w808, "Control Mode"=w823, "PhoenixMotorControlDevRef"=w824) -> ("error out"=w816:errorcluster, "PhoenixMotorControlDevRef"=w817:T7)  [unwired: 6 in]
            n429 = call-poly <vilib>:"WPI_SolenoidSet.vi"("error in (no error)"=w798, "Value"=WPI_SolenoidValue."Reverse", "SolenoidDevRef"=w797) -> ()  [unwired: 7 in, 2 out]
            n430 = call-poly <vilib>:"CTRE_Phoenix_MotorController_Get_TalonFX.vi"("PhoenixMotorControlDevRef"=w817, "error in"=w816) -> ("Velocity"=w804:dbl)  [unwired: 9 in, 4 out]
            n431 = Add(x=w808, y=100.0) -> (x+y=w814:dbl)
            n432 = Subtract(x=w808, y=100.0) -> (x-y=w815:dbl)
            n433 = In Range and Coerce(upper limit=w814, x=w804, lower limit=w815) -> (In Range?=w805:bool)  [unwired: 1 out]
            n434 = call <vilib>:"CTRE_Phoenix_MotorControl_RefNumRegistryGet.vi"("refnum name"="Mag") -> ("error out"=w811:errorcluster, "PhoenixMotorControlDevRef"=w810:T7)  [unwired: 9 in]
            n435 = call-poly <vilib>:"CTRE_Phoenix_MotorControl_SetIntegratedSensorPosition_TalonFX_Polymorphic.vi"("error in (no error)"=w811, "New Position"=0.0, "PhoenixMotorControlDevRef"=w810) -> ()  [unwired: 7 in, 2 out]
            n436 = Select(t=Auto_State_Machine."Shoot OC 2", s=w805, f=Auto_State_Machine."Shoot OC 1") -> (s? t:f=w799:T2)
          }
          frame "Shoot OC 2" {
            w848 = T16 0 items=["PercentOutput"=0, "Position"=1, "Velocity"=2, "Current"=3, "Follower"=5, "MotionProfile"=6, "MotionMagic"=7, "MotionProfileArc"=10, "Disabled"=15] ("Control Mode")
            w852 = T16 2 items=["PercentOutput"=0, "Position"=1, "Velocity"=2, "Current"=3, "Follower"=5, "MotionProfile"=6, "MotionMagic"=7, "MotionProfileArc"=10, "Disabled"=15] ("Control Mode")
            n437 = call "Elapsed Time3"("Time Target (s)"=1.0, "Reset"=FALSE, "Auto Reset"=FALSE, "Set Start Time (s)"=0.0) -> ("Time has Elapsed"=w840:bool)  [unwired: 8 in, 7 out]
            n438 = Negate(x="Oncontact 2 RPM 2") -> (-x=w864:dbl)
            n439 = call <vilib>:"CTRE_Phoenix_MotorControl_RefNumRegistryGet.vi"("refnum name"="Shooter") -> ("error out"=w873:errorcluster, "PhoenixMotorControlDevRef"=w874:T7)  [unwired: 9 in]
            n440 = call <vilib>:"CTRE_Phoenix_MotorControl_ConfigClosedLoopConstants.vi"("PhoenixMotorControlDevRef"=w874, "slotIdx"=3, "P"=0.1, "I"=0.001, "D"=0.0, "error in (no error)"=w873) -> ("PhoenixMotorControlDevRef"=w871:T7, "error out"=w872:errorcluster)  [unwired: 8 in]
            n441 = Multiply(x=3.413, y=w864) -> (x*y=w868:dbl)
            n442 = call <vilib>:"WPI_SolenoidRefNum Registry Get.vi"("refnum name"="Intake") -> ("error out"=w834:errorcluster, "SolenoidDevRef"=w833:T19)  [unwired: 9 in]
            n443 = call <vilib>:"CTRE_Phoenix_MotorControl_SelectProfile Slot.vi"("error in (no error)"=w872, "slotIdx"=3, "PhoenixMotorControlDevRef"=w871) -> ("error out"=w870:errorcluster, "PhoenixMotorControlDevRef"=w869:T7)  [unwired: 7 in]
            n444 = call-poly <vilib>:"WPI_SolenoidSet.vi"("error in (no error)"=w834, "Value"=WPI_SolenoidValue."Reverse", "SolenoidDevRef"=w833) -> ()  [unwired: 7 in, 2 out]
            n445 = case shown="True" w840 {
              tunnel: [FALSE w877] -> w865
              frame False {
              }
              frame True {
                n446 = call <vilib>:"WPI_DigitalInputRefNum Registry Get.vi"("refnum name"="Mag Limit") -> ("error out"=w881:errorcluster, "DigitalInputDevRef"=w880:T5)  [unwired: 9 in]
                n447 = call <vilib>:"WPI_DigitalInputGetValue.vi"("error in (no error)"=w881, "DigitalInputDevRef"=w880) -> ("Value"=w878:bool)  [unwired: 7 in, 2 out]
                n448 = Not(x=w878) -> (.not. x?=w877:bool)
              }
            }
            n449 = call <vilib>:"CTRE_Phoenix_MotorControl_Set.vi"("error in (no error)"=w870, "Output"=w868, "Control Mode"=w852, "PhoenixMotorControlDevRef"=w869) -> ()  [unwired: 6 in, 2 out]
            n450 = call <vilib>:"CTRE_Phoenix_MotorControl_RefNumRegistryGet.vi"("refnum name"="Mag") -> ("error out"=w867:errorcluster, "PhoenixMotorControlDevRef"=w866:T7)  [unwired: 9 in]
            n451 = call <vilib>:"CTRE_Phoenix_MotorControl_Set.vi"("error in (no error)"=w867, "Output"=0.9, "Control Mode"=w848, "PhoenixMotorControlDevRef"=w866) -> ()  [unwired: 6 in, 2 out]
            n452 = call <vilib>:"CTRE_Phoenix_MotorControl_RefNumRegistryGet.vi"("refnum name"="Mag") -> ("error out"=w862:errorcluster, "PhoenixMotorControlDevRef"=w863:T7)  [unwired: 9 in]
            n453 = call-poly <vilib>:"CTRE_Phoenix_MotorController_Get_TalonFX.vi"("PhoenixMotorControlDevRef"=w863, "error in"=w862) -> ("Position (Raw Sensor Units)"=w859:i32)  [unwired: 10 in, 3 out]
            n454 = call-poly <vilib>:"NT Read Value.vi"("Default Value"=140000.0, "Name"="Encoder") -> ("Numeric"=w836:dbl)  [unwired: 8 in, 1 out]
            n455 = To Long Integer(number=w836) -> (32bit integer=w835:i32)
            n456 = Greater?(x=w859, y=w835) -> (0:w860:bool)
            n457 = Or(x=w865, y=w860) -> (x .or. y?=w861:bool)
            n458 = Select(t=Auto_State_Machine."Shoot OC 3", s=w861, f=Auto_State_Machine."Shoot OC 2") -> (s? t:f=w839:T2)
          }
          frame "Shoot OC 3" {
            w897 = T16 0 items=["PercentOutput"=0, "Position"=1, "Velocity"=2, "Current"=3, "Follower"=5, "MotionProfile"=6, "MotionMagic"=7, "MotionProfileArc"=10, "Disabled"=15] ("Control Mode")
            w903 = T16 2 items=["PercentOutput"=0, "Position"=1, "Velocity"=2, "Current"=3, "Follower"=5, "MotionProfile"=6, "MotionMagic"=7, "MotionProfileArc"=10, "Disabled"=15] ("Control Mode")
            n459 = call "Elapsed Time4"("Time Target (s)"=1.0, "Reset"=FALSE, "Auto Reset"=FALSE, "Set Start Time (s)"=0.0) -> ("Time has Elapsed"=w926:bool)  [unwired: 8 in, 7 out]
            n460 = Negate(x="Oncontact 2 RPM 3") -> (-x=w921:dbl)
            n461 = call <vilib>:"CTRE_Phoenix_MotorControl_RefNumRegistryGet.vi"("refnum name"="Shooter") -> ("error out"=w912:errorcluster, "PhoenixMotorControlDevRef"=w911:T7)  [unwired: 9 in]
            n462 = call <vilib>:"CTRE_Phoenix_MotorControl_ConfigClosedLoopConstants.vi"("PhoenixMotorControlDevRef"=w911, "slotIdx"=3, "P"=0.1, "I"=0.001, "D"=0.0, "error in (no error)"=w912) -> ("PhoenixMotorControlDevRef"=w914:T7, "error out"=w913:errorcluster)  [unwired: 8 in]
            n463 = Multiply(x=3.413, y=w921) -> (x*y=w917:dbl)
            n464 = call <vilib>:"CTRE_Phoenix_MotorControl_SelectProfile Slot.vi"("error in (no error)"=w913, "slotIdx"=3, "PhoenixMotorControlDevRef"=w914) -> ("error out"=w915:errorcluster, "PhoenixMotorControlDevRef"=w916:T7)  [unwired: 7 in]
            n465 = case shown="True" w926 {
              tunnel: [FALSE w928] -> w920
              frame False {
              }
              frame True {
                n466 = call <vilib>:"WPI_DigitalInputRefNum Registry Get.vi"("refnum name"="Mag Limit") -> ("error out"=w932:errorcluster, "DigitalInputDevRef"=w931:T5)  [unwired: 9 in]
                n467 = call <vilib>:"WPI_DigitalInputGetValue.vi"("error in (no error)"=w932, "DigitalInputDevRef"=w931) -> ("Value"=w929:bool)  [unwired: 7 in, 2 out]
                n468 = Not(x=w929) -> (.not. x?=w928:bool)
              }
            }
            n469 = call <vilib>:"CTRE_Phoenix_MotorControl_Set.vi"("error in (no error)"=w915, "Output"=w917, "Control Mode"=w903, "PhoenixMotorControlDevRef"=w916) -> ()  [unwired: 6 in, 2 out]
            n470 = call <vilib>:"WPI_SolenoidRefNum Registry Get.vi"("refnum name"="Intake") -> ("error out"=w885:errorcluster, "SolenoidDevRef"=w884:T19)  [unwired: 9 in]
            n471 = call-poly <vilib>:"WPI_SolenoidSet.vi"("error in (no error)"=w885, "Value"=WPI_SolenoidValue."Reverse", "SolenoidDevRef"=w884) -> ()  [unwired: 7 in, 2 out]
            n472 = call <vilib>:"CTRE_Phoenix_MotorControl_RefNumRegistryGet.vi"("refnum name"="Mag") -> ("error out"=w918:errorcluster, "PhoenixMotorControlDevRef"=w919:T7)  [unwired: 9 in]
            n473 = call <vilib>:"CTRE_Phoenix_MotorControl_Set.vi"("error in (no error)"=w918, "Output"=0.9, "Control Mode"=w897, "PhoenixMotorControlDevRef"=w919) -> ()  [unwired: 6 in, 2 out]
            n474 = call <vilib>:"CTRE_Phoenix_MotorControl_RefNumRegistryGet.vi"("refnum name"="Mag") -> ("error out"=w923:errorcluster, "PhoenixMotorControlDevRef"=w922:T7)  [unwired: 9 in]
            n475 = call-poly <vilib>:"CTRE_Phoenix_MotorController_Get_TalonFX.vi"("PhoenixMotorControlDevRef"=w922, "error in"=w923) -> ("Position (Raw Sensor Units)"=w925:i32)  [unwired: 10 in, 3 out]
            n476 = call-poly <vilib>:"NT Read Value.vi"("Default Value"=140000.0, "Name"="Encoder") -> ("Numeric"=w887:dbl)  [unwired: 8 in, 1 out]
            n477 = To Long Integer(number=w887) -> (32bit integer=w886:i32)
            n478 = Greater?(x=w925, y=w886) -> (0:w924:bool)
            n479 = Or(x=w920, y=w924) -> (x .or. y?=w891:bool)
            n480 = Select(t=Auto_State_Machine."OC Reverse", s=w891, f=Auto_State_Machine."Shoot OC 3") -> (s? t:f=w890:T2)
          }
          frame "OC Reverse" {
            w939 = T16 0 items=["PercentOutput"=0, "Position"=1, "Velocity"=2, "Current"=3, "Follower"=5, "MotionProfile"=6, "MotionMagic"=7, "MotionProfileArc"=10, "Disabled"=15] ("Control Mode")
            n481 = call <vilib>:"WPI_SolenoidRefNum Registry Get.vi"("refnum name"="Intake") -> ("error out"=w938:errorcluster, "SolenoidDevRef"=w937:T19)  [unwired: 9 in]
            n482 = call-poly <vilib>:"WPI_SolenoidSet.vi"("error in (no error)"=w938, "Value"=WPI_SolenoidValue."Reverse", "SolenoidDevRef"=w937) -> ()  [unwired: 7 in, 2 out]
            n483 = call <vilib>:"WPI_RobotDriveRefNum Registry Get.vi"("refnum name"="Craig") -> ("error out"=w953:errorcluster, "RobotDriveDevRef"=w954:T21)  [unwired: 9 in]
            n484 = call <vilib>:"CTRE_Phoenix_MotorControl_RefNumRegistryGet.vi"("refnum name"="Mag") -> ("error out"=w943:errorcluster, "PhoenixMotorControlDevRef"=w942:T7)  [unwired: 9 in]
            n485 = call-poly <vilib>:"WPI_RobotDriveHolonomicDrive.vi"("Rotation"=0.0, "error in (no error)"=w953, "Y"=0.15, "X"=0.0, "RobotDriveDevRef"=w954) -> ()  [unwired: 4 in, 3 out]
            n486 = call <vilib>:"CTRE_Phoenix_MotorControl_Set.vi"("error in (no error)"=w943, "Output"=0.0, "Control Mode"=w939, "PhoenixMotorControlDevRef"=w942) -> ()  [unwired: 6 in, 2 out]
            n487 = call "Elapsed Time5"("Time Target (s)"=3.0, "Auto Reset"=FALSE, "Set Start Time (s)"=0.0) -> ("Time has Elapsed"=w933:bool)  [unwired: 9 in, 7 out]
            n488 = Select(t=Auto_State_Machine."Stop", s=w933, f=Auto_State_Machine."OC Reverse") -> (s? t:f=w947:T2)
          }
          frame "Cam Swap 1" {
            n489 = call <vilib>:"Connection Info.vi"() -> ("Connected"=w955:bool)  [unwired: 10 in, 1 out]
            n490 = call-poly <vilib>:"NT Write Value.vi"("Numeric"=1.0, "Name"="/limelight-intake/pipeline") -> ()  [unwired: 9 in, 1 out]
            n491 = Select(t=Auto_State_Machine."Cam Swap 2", s=w955, f=Auto_State_Machine."Cam Swap 1") -> (s? t:f=w958:T2)
          }
          frame "Cam Swap 2" {
            n492 = call "Elapsed Time10"("Time Target (s)"=1.0, "Set Start Time (s)"=0.0) -> ("Present (s)"=w969:dbl)  [unwired: 10 in, 7 out]
            n493 = Greater?(x=w969, y=2.0) -> (0:w965:bool)
            n494 = call-poly <vilib>:"NT Write Value.vi"("Numeric"=0.0, "Name"="/limelight-intake/pipeline") -> ()  [unwired: 9 in, 1 out]
            n495 = Select(t=Auto_State_Machine."Cam Swap 3", s=w965, f=Auto_State_Machine."Cam Swap 2") -> (s? t:f=w962:T2)
          }
          frame "Cam Swap 3" {
            n496 = call "Elapsed Time14"("Time Target (s)"=1.0, "Set Start Time (s)"=0.0) -> ("Present (s)"=w979:dbl)  [unwired: 10 in, 7 out]
            n497 = Greater?(x=w979, y=2.0) -> (0:w975:bool)
            n498 = Select(t=Auto_State_Machine."Auto Wait", s=w975, f=Auto_State_Machine."Cam Swap 3") -> (s? t:f=w974:T2)
            n499 = call-poly <vilib>:"NT Write Value.vi"("Numeric"=1.0, "Name"="/limelight-intake/pipeline") -> ()  [unwired: 9 in, 1 out]
          }
          frame "Go To Ball" {
            w995 = T16 0 items=["PercentOutput"=0, "Position"=1, "Velocity"=2, "Current"=3, "Follower"=5, "MotionProfile"=6, "MotionMagic"=7, "MotionProfileArc"=10, "Disabled"=15] ("Control Mode")
            n500 = call <vilib>:"WPI_DigitalInputRefNum Registry Get.vi"("refnum name"="BB1") -> ("error out"=w999:errorcluster, "DigitalInputDevRef"=w998:T5)  [unwired: 9 in]
            n501 = call <vilib>:"WPI_DigitalInputGetValue.vi"("error in (no error)"=w999, "DigitalInputDevRef"=w998) -> ("Value"=w997:bool)  [unwired: 7 in, 2 out]
            n502 = feedback #1(FALSE) -> (w1003:bool)
            n503 = Not(x=w997) -> (.not. x?=w996:bool)
            n504 = feedback-in #1(w996) -> ()
            n505 = Not(x=w1003) -> (.not. x?=w1004:bool)
            n506 = And(x=w996, y=w1004) -> (x .and. y?=w1005:bool)
            n507 = call-poly <vilib>:"NT Write Value.vi"("Boolean"=FALSE, "Name"="Blind Shot") -> ()  [unwired: 9 in, 1 out]
            n508 = feedback #2() -> (w1006:bool)  [unwired: 1 in]
            n509 = case shown="True" w1005 {
              tunnel: w1006 -> [w1040 w1042]
              tunnel: [w1040 w1041] -> w1001
              frame False {
              }
              frame True {
                n510 = Not(x=w1042) -> (.not. x?=w1041:bool)
              }
            }
            n511 = feedback-in #2(w1001) -> ()
            n512 = call <vilib>:"CTRE_PigeonIMU_RefNumRegistryGet.vi"("refnum name"="Pigeon") -> ("error out"=w1033:errorcluster, "PigeonIMUDevRef"=w1034:T11)  [unwired: 9 in]
            n513 = call-poly <vilib>:"CTRE_PigeonIMU_GetData.vi"("error in (no error)"=w1033, "PigeonIMUDevRef"=w1034) -> ("Yaw Pitch Roll"=w1031:cluster{"Yaw":dbl, "Pitch":dbl, "Roll":dbl})  [unwired: 7 in, 2 out]
            n514 = Unbundle(w1031) -> ("Yaw"=w1030:dbl)  [unwired: 2 out]
            "Yaw 2" <- w1030
            n515 = case shown="True" w1001 {
              frame False {
                w1045 = T16 0 items=["PercentOutput"=0, "Position"=1, "Velocity"=2, "Current"=3, "Follower"=5, "MotionProfile"=6, "MotionMagic"=7, "MotionProfileArc"=10, "Disabled"=15] ("Control Mode")
                n516 = call <vilib>:"CTRE_Phoenix_MotorControl_RefNumRegistryGet.vi"("refnum name"="Mag") -> ("error out"=w1043:errorcluster, "PhoenixMotorControlDevRef"=w1044:T7)  [unwired: 9 in]
                n517 = call <vilib>:"CTRE_Phoenix_MotorControl_Set.vi"("error in (no error)"=w1043, "Output"=0.0, "Control Mode"=w1045, "PhoenixMotorControlDevRef"=w1044) -> ()  [unwired: 6 in, 2 out]
              }
              frame True {
                n518 = global read "Lime.vi" "Timer Good"() -> (w1050:bool)
                n519 = global write "Lime.vi" "Timer Reset"(FALSE ("RPM Good")) -> ()
                n520 = case shown="True" w1050 {
                  tunnel: [FALSE w1072] -> w1059
                  frame False {
                  }
                  frame True {
                    n521 = call <vilib>:"WPI_DigitalInputRefNum Registry Get.vi"("refnum name"="Mag Limit") -> ("error out"=w1075:errorcluster, "DigitalInputDevRef"=w1076:T5)  [unwired: 9 in]
                    n522 = call <vilib>:"WPI_DigitalInputGetValue.vi"("error in (no error)"=w1075, "DigitalInputDevRef"=w1076) -> ("Value"=w1073:bool)  [unwired: 7 in, 2 out]
                    n523 = Not(x=w1073) -> (.not. x?=w1072:bool)
                  }
                }
                n524 = call <vilib>:"CTRE_Phoenix_MotorControl_RefNumRegistryGet.vi"("refnum name"="Mag") -> ("error out"=w1054:errorcluster, "PhoenixMotorControlDevRef"=w1055:T7)  [unwired: 9 in]
                n525 = call-poly <vilib>:"NT Read Value.vi"("Default Value"=67750.0, "Name"="Encoder") -> ("Numeric"=w1052:dbl)  [unwired: 8 in, 1 out]
                n526 = call-poly <vilib>:"CTRE_Phoenix_MotorController_Get_TalonFX.vi"("PhoenixMotorControlDevRef"=w1055, "error in"=w1054) -> ("Position (Raw Sensor Units)"=w1053:i32)  [unwired: 10 in, 3 out]
                n527 = To Long Integer(number=w1052) -> (32bit integer=w1051:i32)
                n528 = Greater?(x=w1053, y=w1051) -> (0:w1060:bool)
                n529 = Or(x=w1060, y=w1059) -> (x .or. y?=w1048:bool)
                n530 = case shown="False" w1048 {
                  frame False {
                    w1063 = T16 0 items=["PercentOutput"=0, "Position"=1, "Velocity"=2, "Current"=3, "Follower"=5, "MotionProfile"=6, "MotionMagic"=7, "MotionProfileArc"=10, "Disabled"=15] ("Control Mode")
                    n531 = call <vilib>:"CTRE_Phoenix_MotorControl_RefNumRegistryGet.vi"("refnum name"="Mag") -> ("error out"=w1061:errorcluster, "PhoenixMotorControlDevRef"=w1062:T7)  [unwired: 9 in]
                    n532 = call <vilib>:"CTRE_Phoenix_MotorControl_Set.vi"("error in (no error)"=w1061, "Output"=0.65, "Control Mode"=w1063, "PhoenixMotorControlDevRef"=w1062) -> ()  [unwired: 6 in, 2 out]
                  }
                  frame True {
                    w1068 = T16 0 items=["PercentOutput"=0, "Position"=1, "Velocity"=2, "Current"=3, "Follower"=5, "MotionProfile"=6, "MotionMagic"=7, "MotionProfileArc"=10, "Disabled"=15] ("Control Mode")
                    n533 = call <vilib>:"CTRE_Phoenix_MotorControl_RefNumRegistryGet.vi"("refnum name"="Mag") -> ("error out"=w1066:errorcluster, "PhoenixMotorControlDevRef"=w1067:T7)  [unwired: 9 in]
                    n534 = call <vilib>:"CTRE_Phoenix_MotorControl_Set.vi"("error in (no error)"=w1066, "Output"=0.0, "Control Mode"=w1068, "PhoenixMotorControlDevRef"=w1067) -> ()  [unwired: 6 in, 2 out]
                  }
                }
              }
            }
            n535 = call-poly <vilib>:"PID.vi"("output range"=cluster{"output high":dbl, "output low":dbl} {"output high"=100.0, "output low"=-100.0}, "PID gains"="PID gains 2", "process variable"=w1030, "setpoint"="setpoint") -> ("output"=w1025:dbl)  [unwired: 6 in, 1 out]
            n536 = global read "Lime.vi" "Side F/B Drive"() -> (w1009:dbl)
            n537 = Divide(x=w1025, y=100.0) -> (x/y=w1026:dbl)
            n538 = Negate(x=w1026) -> (-x=w1023:dbl)
            n539 = call <vilib>:"WPI_RobotDriveRefNum Registry Get.vi"("refnum name"="Craig") -> ("error out"=w1036:errorcluster, "RobotDriveDevRef"=w1037:T21)  [unwired: 9 in]
            n540 = call-poly <vilib>:"WPI_RobotDriveHolonomicDrive.vi"("Rotation"=w1023, "error in (no error)"=w1036, "Y"=w1009, "X"=0.3, "RobotDriveDevRef"=w1037) -> ()  [unwired: 4 in, 3 out]
            n541 = call "Elapsed Time9"("Time Target (s)"=3.0, "Reset"=FALSE, "Auto Reset"=FALSE, "Set Start Time (s)"=0.0) -> ("Time has Elapsed"=w983:bool)  [unwired: 8 in, 7 out]
            n542 = call <vilib>:"WPI_SolenoidRefNum Registry Get.vi"("refnum name"="Intake") -> ("error out"=w1021:errorcluster, "SolenoidDevRef"=w1020:T19)  [unwired: 9 in]
            n543 = global write "Lime.vi" "Shooter Pipeline"(1.0 ("Shooter Pipeline")) -> ()
            n544 = call-poly <vilib>:"WPI_SolenoidSet.vi"("error in (no error)"=w1021, "Value"=WPI_SolenoidValue."Forward", "SolenoidDevRef"=w1020) -> ()  [unwired: 7 in, 2 out]
            n545 = global read "Lime.vi" "Side F/B Error"() -> (w1007:dbl)
            n546 = global write "Lime.vi" "Enabled"(FALSE ("Enabled")) -> ()
            n547 = Equal To 0?(x=w1007) -> (x = 0?=w1008:bool)
            n548 = Or(x=w983, y=w1008) -> (x .or. y?=w988:bool)
            n549 = call <vilib>:"WPI_DriverStationGet Alliance Info.vi"() -> ("Alliance"=w991:T17)  [unwired: 6 in, 5 out]
            n550 = Equal?(x=WPI_DriverStationAllianceInfo."Red", y=w991) -> (x = y?=w990:bool)
            n551 = case shown="False" w990 {
              tunnel: [0.0 ("Numeric") 1.0 ("Numeric")] -> w992
              frame False {
              }
              frame True {
              }
            }
            n552 = Select(t=Auto_State_Machine."Intake", s=w988, f=Auto_State_Machine."Go To Ball") -> (s? t:f=w1015:T2)
            n553 = call <vilib>:"CTRE_Phoenix_MotorControl_RefNumRegistryGet.vi"("refnum name"="Intake") -> ("error out"=w1014:errorcluster, "PhoenixMotorControlDevRef"=w1013:T7)  [unwired: 9 in]
            n554 = call <vilib>:"CTRE_Phoenix_MotorControl_Set.vi"("error in (no error)"=w1014, "Output"=-0.9, "Control Mode"=w995, "PhoenixMotorControlDevRef"=w1013) -> ()  [unwired: 6 in, 2 out]
            n555 = call "NT Write Number_On Change.vi"("Numeric"=w992, "Name"="/limelight-intake/pipeline") -> ()  [unwired: 9 in, 1 out]
          }
          frame "Intake" {
            w1086 = T16 0 items=["PercentOutput"=0, "Position"=1, "Velocity"=2, "Current"=3, "Follower"=5, "MotionProfile"=6, "MotionMagic"=7, "MotionProfileArc"=10, "Disabled"=15] ("Control Mode")
            n556 = call <vilib>:"CTRE_PigeonIMU_RefNumRegistryGet.vi"("refnum name"="Pigeon") -> ("error out"=w1107:errorcluster, "PigeonIMUDevRef"=w1108:T11)  [unwired: 9 in]
            n557 = call-poly <vilib>:"CTRE_PigeonIMU_GetData.vi"("error in (no error)"=w1107, "PigeonIMUDevRef"=w1108) -> ("Yaw Pitch Roll"=w1105:cluster{"Yaw":dbl, "Pitch":dbl, "Roll":dbl})  [unwired: 7 in, 2 out]
            n558 = Unbundle(w1105) -> ("Yaw"=w1104:dbl)  [unwired: 2 out]
            "Yaw 3" <- w1104
            n559 = call-poly <vilib>:"PID.vi"("output range"=cluster{"output high":dbl, "output low":dbl} {"output high"=100.0, "output low"=-100.0}, "PID gains"="PID gains 3", "process variable"=w1104, "setpoint"="setpoint 2") -> ("output"=w1099:dbl)  [unwired: 6 in, 1 out]
            n560 = Divide(x=w1099, y=100.0) -> (x/y=w1100:dbl)
            n561 = Negate(x=w1100) -> (-x=w1097:dbl)
            n562 = call <vilib>:"WPI_RobotDriveRefNum Registry Get.vi"("refnum name"="Craig") -> ("error out"=w1110:errorcluster, "RobotDriveDevRef"=w1111:T21)  [unwired: 9 in]
            n563 = call-poly <vilib>:"WPI_RobotDriveHolonomicDrive.vi"("Rotation"=w1097, "error in (no error)"=w1110, "Y"=0.0, "X"=0.0, "RobotDriveDevRef"=w1111) -> ()  [unwired: 4 in, 3 out]
            n564 = global write "Lime.vi" "Enabled"(FALSE ("Enabled")) -> ()
            n565 = call <vilib>:"WPI_SolenoidRefNum Registry Get.vi"("refnum name"="Intake") -> ("error out"=w1092:errorcluster, "SolenoidDevRef"=w1091:T19)  [unwired: 9 in]
            n566 = call-poly <vilib>:"WPI_SolenoidSet.vi"("error in (no error)"=w1092, "Value"=WPI_SolenoidValue."Forward", "SolenoidDevRef"=w1091) -> ()  [unwired: 7 in, 2 out]
            n567 = call "Elapsed Time8"("Time Target (s)"=2.0, "Reset"=FALSE, "Auto Reset"=FALSE, "Set Start Time (s)"=0.0) -> ("Time has Elapsed"=w1079:bool)  [unwired: 8 in, 7 out]
            n568 = call <vilib>:"CTRE_Phoenix_MotorControl_RefNumRegistryGet.vi"("refnum name"="Intake") -> ("error out"=w1088:errorcluster, "PhoenixMotorControlDevRef"=w1087:T7)  [unwired: 9 in]
            n569 = call <vilib>:"CTRE_Phoenix_MotorControl_Set.vi"("error in (no error)"=w1088, "Output"=-0.9, "Control Mode"=w1086, "PhoenixMotorControlDevRef"=w1087) -> ()  [unwired: 6 in, 2 out]
            n570 = Select(t=Auto_State_Machine."Intake Up", s=w1079, f=Auto_State_Machine."Intake") -> (s? t:f=w1093:T2)
          }
          frame "Intake Up" {
            w1122 = T16 0 items=["PercentOutput"=0, "Position"=1, "Velocity"=2, "Current"=3, "Follower"=5, "MotionProfile"=6, "MotionMagic"=7, "MotionProfileArc"=10, "Disabled"=15] ("Control Mode")
            n571 = call <vilib>:"CTRE_PigeonIMU_RefNumRegistryGet.vi"("refnum name"="Pigeon") -> ("error out"=w1142:errorcluster, "PigeonIMUDevRef"=w1143:T11)  [unwired: 9 in]
            n572 = call-poly <vilib>:"CTRE_PigeonIMU_GetData.vi"("error in (no error)"=w1142, "PigeonIMUDevRef"=w1143) -> ("Yaw Pitch Roll"=w1140:cluster{"Yaw":dbl, "Pitch":dbl, "Roll":dbl})  [unwired: 7 in, 2 out]
            n573 = Unbundle(w1140) -> ("Yaw"=w1139:dbl)  [unwired: 2 out]
            "Yaw 5" <- w1139
            n574 = call-poly <vilib>:"PID.vi"("output range"=cluster{"output high":dbl, "output low":dbl} {"output high"=100.0, "output low"=-100.0}, "PID gains"="PID gains 5", "process variable"=w1139, "setpoint"="setpoint 4") -> ("output"=w1134:dbl)  [unwired: 6 in, 1 out]
            n575 = Divide(x=w1134, y=100.0) -> (x/y=w1135:dbl)
            n576 = Negate(x=w1135) -> (-x=w1132:dbl)
            n577 = call <vilib>:"WPI_RobotDriveRefNum Registry Get.vi"("refnum name"="Craig") -> ("error out"=w1145:errorcluster, "RobotDriveDevRef"=w1146:T21)  [unwired: 9 in]
            n578 = call-poly <vilib>:"WPI_RobotDriveHolonomicDrive.vi"("Rotation"=w1132, "error in (no error)"=w1145, "Y"=0.0, "X"=0.0, "RobotDriveDevRef"=w1146) -> ()  [unwired: 4 in, 3 out]
            n579 = global write "Lime.vi" "Enabled"(FALSE ("Enabled")) -> ()
            n580 = call <vilib>:"WPI_SolenoidRefNum Registry Get.vi"("refnum name"="Intake") -> ("error out"=w1128:errorcluster, "SolenoidDevRef"=w1127:T19)  [unwired: 9 in]
            n581 = call-poly <vilib>:"WPI_SolenoidSet.vi"("error in (no error)"=w1128, "Value"=WPI_SolenoidValue."Reverse", "SolenoidDevRef"=w1127) -> ()  [unwired: 7 in, 2 out]
            n582 = call "Elapsed Time7"("Time Target (s)"=1.0, "Reset"=FALSE, "Auto Reset"=FALSE, "Set Start Time (s)"=0.0) -> ("Time has Elapsed"=w1115:bool)  [unwired: 8 in, 7 out]
            n583 = call <vilib>:"CTRE_Phoenix_MotorControl_RefNumRegistryGet.vi"("refnum name"="Intake") -> ("error out"=w1124:errorcluster, "PhoenixMotorControlDevRef"=w1123:T7)  [unwired: 9 in]
            n584 = call <vilib>:"CTRE_Phoenix_MotorControl_Set.vi"("error in (no error)"=w1124, "Output"=-0.7, "Control Mode"=w1122, "PhoenixMotorControlDevRef"=w1123) -> ()  [unwired: 6 in, 2 out]
            n585 = Select(t=Auto_State_Machine."Rotate & Auger", s=w1115, f=Auto_State_Machine."Intake Up") -> (s? t:f=w1112:T2)
          }
          frame "Rotate & Auger" {
            w1151 = 2.0 ("lower limit")
            w1197 = T16 2 items=["PercentOutput"=0, "Position"=1, "Velocity"=2, "Current"=3, "Follower"=5, "MotionProfile"=6, "MotionMagic"=7, "MotionProfileArc"=10, "Disabled"=15] ("Control Mode")
            w1208 = T16 0 items=["PercentOutput"=0, "Position"=1, "Velocity"=2, "Current"=3, "Follower"=5, "MotionProfile"=6, "MotionMagic"=7, "MotionProfileArc"=10, "Disabled"=15] ("Control Mode")
            n586 = call "Elapsed Time13"("Auto Reset"=FALSE) -> ("Time has Elapsed"=w1147:bool)  [unwired: 11 in, 7 out]
            n587 = case shown="False" w1147 {
              frame False {
              }
              frame True {
                n588 = call "Elapsed Time11"("Time Target (s)"="Total Time", "Reset"=FALSE, "Auto Reset"=TRUE, "Set Start Time (s)"=0.0) -> ("Elapsed Time (s)"=w1213:dbl)  [unwired: 8 in, 7 out]
                n589 = Greater Or Equal?(x=w1213, y="Time Low") -> (x >= y?=w1212:bool)
                n590 = case shown="True" w1212 {
                  frame False {
                    n591 = call <vilib>:"WPI_SolenoidRefNum Registry Get.vi"("refnum name"="Intake") -> ("error out"=w1221:errorcluster, "SolenoidDevRef"=w1220:T19)  [unwired: 9 in]
                    n592 = call-poly <vilib>:"WPI_SolenoidSet.vi"("error in (no error)"=w1221, "Value"=WPI_SolenoidValue."Reverse", "SolenoidDevRef"=w1220) -> ()  [unwired: 7 in, 2 out]
                  }
                  frame True {
                    n593 = call <vilib>:"WPI_SolenoidRefNum Registry Get.vi"("refnum name"="Intake") -> ("error out"=w1225:errorcluster, "SolenoidDevRef"=w1224:T19)  [unwired: 9 in]
                    n594 = call-poly <vilib>:"WPI_SolenoidSet.vi"("error in (no error)"=w1225, "Value"=WPI_SolenoidValue."Forward", "SolenoidDevRef"=w1224) -> ()  [unwired: 7 in, 2 out]
                  }
                }
              }
            }
            n595 = call <vilib>:"CTRE_PigeonIMU_RefNumRegistryGet.vi"("refnum name"="Pigeon") -> ("error out"=w1165:errorcluster, "PigeonIMUDevRef"=w1166:T11)  [unwired: 9 in]
            n596 = call-poly <vilib>:"CTRE_PigeonIMU_GetData.vi"("error in (no error)"=w1165, "PigeonIMUDevRef"=w1166) -> ("Yaw Pitch Roll"=w1163:cluster{"Yaw":dbl, "Pitch":dbl, "Roll":dbl})  [unwired: 7 in, 2 out]
            n597 = Unbundle(w1163) -> ("Yaw"=w1154:dbl)  [unwired: 2 out]
            "Yaw 7" <- w1154
            n598 = call-poly <vilib>:"PID.vi"("output range"=cluster{"output high":dbl, "output low":dbl} {"output high"=100.0, "output low"=-100.0}, "PID gains"="PID gains 7", "process variable"=w1154, "setpoint"="setpoint 6") -> ("output"=w1159:dbl)  [unwired: 6 in, 1 out]
            n599 = Add(x="setpoint 6", y=w1151) -> (x+y=w1153:dbl)
            n600 = Subtract(x="setpoint 6", y=w1151) -> (x-y=w1152:dbl)
            n601 = In Range and Coerce(upper limit=w1153, x=w1154, lower limit=w1152) -> (In Range?=w1149:bool)  [unwired: 1 out]
            n602 = Divide(x=w1159, y=100.0) -> (x/y=w1160:dbl)
            n603 = Negate(x=w1160) -> (-x=w1157:dbl)
            n604 = Negate(x=3400.0) -> (-x=w1189:dbl)
            n605 = call <vilib>:"CTRE_Phoenix_MotorControl_RefNumRegistryGet.vi"("refnum name"="Shooter") -> ("error out"=w1203:errorcluster, "PhoenixMotorControlDevRef"=w1204:T7)  [unwired: 9 in]
            n606 = Multiply(x="x 3", y=w1157) -> (x*y=w1170:dbl)
            n607 = Multiply(x=w1170, y=0.6) -> (x*y=w1168:dbl)
            n608 = call <vilib>:"CTRE_Phoenix_MotorControl_ConfigClosedLoopConstants.vi"("PhoenixMotorControlDevRef"=w1204, "slotIdx"=3, "P"=0.1, "I"=0.001, "D"=0.0, "error in (no error)"=w1203) -> ("PhoenixMotorControlDevRef"=w1200:T7, "error out"=w1201:errorcluster)  [unwired: 8 in]
            n609 = Multiply(x=3.413, y=w1189) -> (x*y=w1191:dbl)
            n610 = call <vilib>:"WPI_RobotDriveRefNum Registry Get.vi"("refnum name"="Craig") -> ("error out"=w1172:errorcluster, "RobotDriveDevRef"=w1173:T21)  [unwired: 9 in]
            n611 = call <vilib>:"CTRE_Phoenix_MotorControl_SelectProfile Slot.vi"("error in (no error)"=w1201, "slotIdx"=3, "PhoenixMotorControlDevRef"=w1200) -> ("error out"=w1199:errorcluster, "PhoenixMotorControlDevRef"=w1198:T7)  [unwired: 7 in]
            n612 = call <vilib>:"CTRE_Phoenix_MotorControl_Set.vi"("error in (no error)"=w1199, "Output"=w1191, "Control Mode"=w1197, "PhoenixMotorControlDevRef"=w1198) -> ()  [unwired: 6 in, 2 out]
            n613 = global write "Lime.vi" "Enabled"(TRUE ("Enabled")) -> ()
            n614 = call-poly <vilib>:"WPI_RobotDriveHolonomicDrive.vi"("Rotation"=w1168, "error in (no error)"=w1172, "Y"=0.0, "X"=0.0, "RobotDriveDevRef"=w1173) -> ()  [unwired: 4 in, 3 out]
            n615 = call <vilib>:"WPI_DigitalInputRefNum Registry Get.vi"("refnum name"="BB1") -> ("error out"=w1185:errorcluster, "DigitalInputDevRef"=w1184:T5)  [unwired: 9 in]
            n616 = call <vilib>:"WPI_DigitalInputGetValue.vi"("error in (no error)"=w1185, "DigitalInputDevRef"=w1184) -> ("Value"=w1183:bool)  [unwired: 7 in, 2 out]
            n617 = call "Elapsed Time6"("Time Target (s)"=2.5, "Reset"=FALSE, "Auto Reset"=FALSE, "Set Start Time (s)"=0.0) -> ("Time has Elapsed"=w1175:bool)  [unwired: 8 in, 7 out]
            n618 = Not(x=w1183) -> (.not. x?=w1182:bool)
            n619 = call <vilib>:"CTRE_Phoenix_MotorControl_RefNumRegistryGet.vi"("refnum name"="Intake") -> ("error out"=w1210:errorcluster, "PhoenixMotorControlDevRef"=w1209:T7)  [unwired: 9 in]
            n620 = And(x=w1149, y=w1182) -> (x .and. y?=w1181:bool)
            n621 = call <vilib>:"CTRE_Phoenix_MotorControl_Set.vi"("error in (no error)"=w1210, "Output"=-1.0, "Control Mode"=w1208, "PhoenixMotorControlDevRef"=w1209) -> ()  [unwired: 6 in, 2 out]
            n622 = Or(x=w1181, y=w1175) -> (x .or. y?=w1176:bool)
            n623 = Select(t=Auto_State_Machine."Limelight Happy?", s=w1176, f=Auto_State_Machine."Rotate & Auger") -> (s? t:f=w1205:T2)
          }
          frame "Limelight Happy?" {
            w1239 = 7.0 ("upper limit")
            w1248 = T16 0 items=["PercentOutput"=0, "Position"=1, "Velocity"=2, "Current"=3, "Follower"=5, "MotionProfile"=6, "MotionMagic"=7, "MotionProfileArc"=10, "Disabled"=15] ("Control Mode")
            w1260 = 100.0 ("y")
            w1280 = T16 2 items=["PercentOutput"=0, "Position"=1, "Velocity"=2, "Current"=3, "Follower"=5, "MotionProfile"=6, "MotionMagic"=7, "MotionProfileArc"=10, "Disabled"=15] ("Control Mode")
            w1300 = T16 0 items=["PercentOutput"=0, "Position"=1, "Velocity"=2, "Current"=3, "Follower"=5, "MotionProfile"=6, "MotionMagic"=7, "MotionProfileArc"=10, "Disabled"=15] ("Control Mode")
            n624 = call <vilib>:"CTRE_Phoenix_MotorControl_RefNumRegistryGet.vi"("refnum name"="Mag") -> ("error out"=w1255:errorcluster, "PhoenixMotorControlDevRef"=w1254:T7)  [unwired: 9 in]
            n625 = call-poly <vilib>:"CTRE_Phoenix_MotorControl_SetIntegratedSensorPosition_TalonFX_Polymorphic.vi"("error in (no error)"=w1255, "New Position"=0.0, "PhoenixMotorControlDevRef"=w1254) -> ("error out"=w1250:errorcluster, "PhoenixMotorControlDevRef"=w1251:T7)  [unwired: 7 in]
            n626 = Negate(x=3300.0 ("Default Value")) -> (-x=w1267:dbl)
            n627 = call <vilib>:"CTRE_Phoenix_MotorControl_RefNumRegistryGet.vi"("refnum name"="Shooter") -> ("error out"=w1286:errorcluster, "PhoenixMotorControlDevRef"=w1287:T7)  [unwired: 9 in]
            n628 = call <vilib>:"CTRE_Phoenix_MotorControl_Set.vi"("error in (no error)"=w1250, "Output"=0.0, "Control Mode"=w1248, "PhoenixMotorControlDevRef"=w1251) -> ()  [unwired: 6 in, 2 out]
            n629 = call <vilib>:"CTRE_Phoenix_MotorControl_ConfigClosedLoopConstants.vi"("PhoenixMotorControlDevRef"=w1287, "slotIdx"=3, "P"=0.1, "I"=0.001, "D"=0.0, "error in (no error)"=w1286) -> ("PhoenixMotorControlDevRef"=w1283:T7, "error out"=w1284:errorcluster)  [unwired: 8 in]
            n630 = Multiply(x=3.413, y=w1267) -> (x*y=w1270:dbl)
            n631 = call <vilib>:"CTRE_Phoenix_MotorControl_SelectProfile Slot.vi"("error in (no error)"=w1284, "slotIdx"=3, "PhoenixMotorControlDevRef"=w1283) -> ("error out"=w1282:errorcluster, "PhoenixMotorControlDevRef"=w1281:T7)  [unwired: 7 in]
            n632 = global write "Lime.vi" "Timer Reset"(TRUE ("RPM Good")) -> ()
            n633 = call <vilib>:"CTRE_Phoenix_MotorControl_Set.vi"("error in (no error)"=w1282, "Output"=w1270, "Control Mode"=w1280, "PhoenixMotorControlDevRef"=w1281) -> ("error out"=w1273:errorcluster, "PhoenixMotorControlDevRef"=w1274:T7)  [unwired: 6 in]
            n634 = call-poly <vilib>:"CTRE_Phoenix_MotorController_Get_TalonFX.vi"("PhoenixMotorControlDevRef"=w1274, "error in"=w1273) -> ("Velocity"=w1268:dbl)  [unwired: 9 in, 4 out]
            n635 = call <vilib>:"CTRE_Phoenix_MotorControl_RefNumRegistryGet.vi"("refnum name"="Intake") -> ("error out"=w1302:errorcluster, "PhoenixMotorControlDevRef"=w1301:T7)  [unwired: 9 in]
            n636 = global write "Lime.vi" "Enabled"(TRUE ("Enabled")) -> ()
            n637 = call <vilib>:"WPI_RobotDriveRefNum Registry Get.vi"("refnum name"="Craig") -> ("error out"=w1305:errorcluster, "RobotDriveDevRef"=w1306:T21)  [unwired: 9 in]
            n638 = call <vilib>:"CTRE_Phoenix_MotorControl_Set.vi"("error in (no error)"=w1302, "Output"=-1.0, "Control Mode"=w1300, "PhoenixMotorControlDevRef"=w1301) -> ()  [unwired: 6 in, 2 out]
            n639 = global read "Lime.vi" "Rotate"() -> (w1289:dbl)
            n640 = call-poly <vilib>:"WPI_RobotDriveHolonomicDrive.vi"("Rotation"=w1289, "error in (no error)"=w1305, "Y"=0.0, "X"=0.0, "RobotDriveDevRef"=w1306) -> ()  [unwired: 4 in, 3 out]
            n641 = Add(x=w1270, y=w1260) -> (x+y=w1271:dbl)
            n642 = Subtract(x=w1270, y=w1260) -> (x-y=w1272:dbl)
            n643 = In Range and Coerce(upper limit=w1271, x=w1268, lower limit=w1272) -> (In Range?=w1264:bool)  [unwired: 1 out]
            n644 = global read "Lime.vi" "Rotate Error"() -> (w1241:dbl)
            n645 = global read "Lime.vi" "Rotate Error"() -> (w1288:dbl)
            n646 = Negate(x=w1239) -> (-x=w1240:dbl)
            n647 = In Range and Coerce(upper limit=w1239, x=w1241, lower limit=w1240) -> (In Range?=w1235:bool)  [unwired: 1 out]
            n648 = Negate(x="LL Deadband") -> (-x=w1256:dbl)
            n649 = call-poly <vilib>:"NT Read Value.vi"("Name"="/limelight-shoot/tv") -> ("Numeric"=w1231:dbl)  [unwired: 9 in, 1 out]
            n650 = In Range and Coerce(upper limit="LL Deadband", x=w1288, lower limit=w1256) -> (In Range?=w1265:bool)  [unwired: 1 out]
            n651 = Not(x=w1235) -> (.not. x?=w1229:bool)
            n652 = Equal To 0?(x=w1231) -> (x = 0?=w1228:bool)
            n653 = call <vilib>:"WPI_SolenoidRefNum Registry Get.vi"("refnum name"="Intake") -> ("error out"=w1296:errorcluster, "SolenoidDevRef"=w1295:T19)  [unwired: 9 in]
            n654 = Not Equal To 0?(x=w1231) -> (x != 0?=w1230:bool)
            n655 = call <vilib>:"WPI_DigitalInputRefNum Registry Get.vi"("refnum name"="BB1") -> ("error out"=w1246:errorcluster, "DigitalInputDevRef"=w1245:T5)  [unwired: 9 in]
            n656 = call-poly <vilib>:"WPI_SolenoidSet.vi"("error in (no error)"=w1296, "Value"=WPI_SolenoidValue."Reverse", "SolenoidDevRef"=w1295) -> ()  [unwired: 7 in, 2 out]
            n657 = Or(x=w1228, y=w1229) -> (x .or. y?=w1227:bool)
            n658 = Compound Arithmetic op=AND(w1265, w1264, w1230) -> (w1237:bool)
            n659 = call <vilib>:"WPI_DigitalInputGetValue.vi"("error in (no error)"=w1246, "DigitalInputDevRef"=w1245) -> ("Value"=w1244:bool)  [unwired: 7 in, 2 out]
            n660 = call <vilib>:"WPI_DriverStationGetRemainingMatchTime.vi"() -> ("Match Time(s)"=w1291:sgl)  [unwired: 10 in, 1 out]
            n661 = Not(x=w1244) -> (.not. x?=w1243:bool)
            n662 = Less Or Equal?(x=w1291, y=sgl 4.0 ("Match Time(s)")) -> (x <= y?=w1236:bool)
            n663 = Select(t=Auto_State_Machine."LL Shoot 1", s=w1243, f=Auto_State_Machine."LL Shoot 2") -> (s? t:f=w1238:T2)
            n664 = Compound Arithmetic op=AND(w1227, w1236) -> (w1234:bool)
            n665 = Select(t=Auto_State_Machine."Pigeon Rotate" ("f"), s=w1234, f=Auto_State_Machine."Limelight Happy?") -> (s? t:f=w1232:T2)
            n666 = Select(t=w1238, s=w1237, f=w1232) -> (s? t:f=w1258:T2)
          }
          frame "LL Shoot 1" {
            w1334 = T16 0 items=["PercentOutput"=0, "Position"=1, "Velocity"=2, "Current"=3, "Follower"=5, "MotionProfile"=6, "MotionMagic"=7, "MotionProfileArc"=10, "Disabled"=15] ("Control Mode")
            w1344 = T16 2 items=["PercentOutput"=0, "Position"=1, "Velocity"=2, "Current"=3, "Follower"=5, "MotionProfile"=6, "MotionMagic"=7, "MotionProfileArc"=10, "Disabled"=15] ("Control Mode")
            n667 = global write "Lime.vi" "Timer Reset"(FALSE ("RPM Good")) -> ()
            n668 = Negate(x=3300.0) -> (-x=w1330:dbl)
            n669 = call <vilib>:"CTRE_Phoenix_MotorControl_RefNumRegistryGet.vi"("refnum name"="Shooter") -> ("error out"=w1350:errorcluster, "PhoenixMotorControlDevRef"=w1351:T7)  [unwired: 9 in]
            n670 = global read "Lime.vi" "Timer Good"() -> (w1319:bool)
            n671 = call <vilib>:"CTRE_Phoenix_MotorControl_ConfigClosedLoopConstants.vi"("PhoenixMotorControlDevRef"=w1351, "slotIdx"=3, "P"=0.1, "I"=0.001, "D"=0.0, "error in (no error)"=w1350) -> ("PhoenixMotorControlDevRef"=w1347:T7, "error out"=w1348:errorcluster)  [unwired: 8 in]
            n672 = Multiply(x=3.413, y=w1330) -> (x*y=w1338:dbl)
            n673 = call <vilib>:"CTRE_Phoenix_MotorControl_SelectProfile Slot.vi"("error in (no error)"=w1348, "slotIdx"=3, "PhoenixMotorControlDevRef"=w1347) -> ("error out"=w1346:errorcluster, "PhoenixMotorControlDevRef"=w1345:T7)  [unwired: 7 in]
            n674 = case shown="True" w1319 {
              tunnel: [FALSE w1353] -> w1331
              frame False {
              }
              frame True {
                n675 = disable-structure shown="Disabled" {
                  disable-tunnel: [w1358 _] -> _
                  frame Disabled {
                    n676 = call <vilib>:"WPI_DigitalInputRefNum Registry Get.vi"("refnum name"="LS2") -> ("error out"=w1365:errorcluster, "DigitalInputDevRef"=w1366:T5)  [unwired: 9 in]
                    n677 = call <vilib>:"WPI_DigitalInputRefNum Registry Get.vi"("refnum name"="LS1") -> ("error out"=w1361:errorcluster, "DigitalInputDevRef"=w1360:T5)  [unwired: 9 in]
                    n678 = call <vilib>:"WPI_DigitalInputGetValue.vi"("error in (no error)"=w1365, "DigitalInputDevRef"=w1366) -> ("Value"=w1363:bool)  [unwired: 7 in, 2 out]
                    n679 = call <vilib>:"WPI_DigitalInputGetValue.vi"("error in (no error)"=w1361, "DigitalInputDevRef"=w1360) -> ("Value"=w1359:bool)  [unwired: 7 in, 2 out]
                    n680 = Or(x=w1363, y=w1359) -> (x .or. y?=w1358:bool)
                  }
                  frame Enabled {
                  }
                }
                n681 = call <vilib>:"WPI_DigitalInputRefNum Registry Get.vi"("refnum name"="Mag Limit") -> ("error out"=w1357:errorcluster, "DigitalInputDevRef"=w1356:T5)  [unwired: 9 in]
                n682 = call <vilib>:"WPI_DigitalInputGetValue.vi"("error in (no error)"=w1357, "DigitalInputDevRef"=w1356) -> ("Value"=w1354:bool)  [unwired: 7 in, 2 out]
                n683 = Not(x=w1354) -> (.not. x?=w1353:bool)
              }
            }
            n684 = call <vilib>:"CTRE_Phoenix_MotorControl_Set.vi"("error in (no error)"=w1346, "Output"=w1338, "Control Mode"=w1344, "PhoenixMotorControlDevRef"=w1345) -> ()  [unwired: 6 in, 2 out]
            n685 = global write "Lime.vi" "Enabled"(TRUE ("Enabled")) -> ()
            n686 = call <vilib>:"CTRE_Phoenix_MotorControl_RefNumRegistryGet.vi"("refnum name"="Mag") -> ("error out"=w1336:errorcluster, "PhoenixMotorControlDevRef"=w1335:T7)  [unwired: 9 in]
            n687 = call <vilib>:"CTRE_Phoenix_MotorControl_Set.vi"("error in (no error)"=w1336, "Output"=0.9, "Control Mode"=w1334, "PhoenixMotorControlDevRef"=w1335) -> ()  [unwired: 6 in, 2 out]
            n688 = call <vilib>:"CTRE_Phoenix_MotorControl_RefNumRegistryGet.vi"("refnum name"="Mag") -> ("error out"=w1323:errorcluster, "PhoenixMotorControlDevRef"=w1324:T7)  [unwired: 9 in]
            n689 = call-poly <vilib>:"CTRE_Phoenix_MotorController_Get_TalonFX.vi"("PhoenixMotorControlDevRef"=w1324, "error in"=w1323) -> ("Position (Raw Sensor Units)"=w1322:i32)  [unwired: 10 in, 3 out]
            n690 = call <vilib>:"WPI_RobotDriveRefNum Registry Get.vi"("refnum name"="Craig") -> ("error out"=w1311:errorcluster, "RobotDriveDevRef"=w1312:T21)  [unwired: 9 in]
            n691 = call-poly <vilib>:"NT Read Value.vi"("Default Value"=67750.0, "Name"="Encoder") -> ("Numeric"=w1320:dbl)  [unwired: 8 in, 1 out]
            n692 = global read "Lime.vi" "Rotate"() -> (w1307:dbl)
            n693 = To Long Integer(number=w1320) -> (32bit integer=w1321:i32)
            n694 = Greater?(x=w1322, y=w1321) -> (0:w1328:bool)
            n695 = call-poly <vilib>:"WPI_RobotDriveHolonomicDrive.vi"("Rotation"=w1307, "error in (no error)"=w1311, "Y"=0.0, "X"=0.0, "RobotDriveDevRef"=w1312) -> ()  [unwired: 4 in, 3 out]
            n696 = Or(x=w1331, y=w1328) -> (x .or. y?=w1329:bool)
            n697 = Select(t=Auto_State_Machine."Limelight Happy?", s=w1329, f=Auto_State_Machine."LL Shoot 1") -> (s? t:f=w1315:T2)
          }
          frame "LL Shoot 2" {
            w1393 = T16 0 items=["PercentOutput"=0, "Position"=1, "Velocity"=2, "Current"=3, "Follower"=5, "MotionProfile"=6, "MotionMagic"=7, "MotionProfileArc"=10, "Disabled"=15] ("Control Mode")
            w1403 = T16 2 items=["PercentOutput"=0, "Position"=1, "Velocity"=2, "Current"=3, "Follower"=5, "MotionProfile"=6, "MotionMagic"=7, "MotionProfileArc"=10, "Disabled"=15] ("Control Mode")
            n698 = global write "Lime.vi" "Timer Reset"(FALSE ("RPM Good")) -> ()
            n699 = Negate(x=3300.0) -> (-x=w1389:dbl)
            n700 = call <vilib>:"CTRE_Phoenix_MotorControl_RefNumRegistryGet.vi"("refnum name"="Shooter") -> ("error out"=w1409:errorcluster, "PhoenixMotorControlDevRef"=w1410:T7)  [unwired: 9 in]
            n701 = global read "Lime.vi" "Timer Good"() -> (w1379:bool)
            n702 = call <vilib>:"CTRE_Phoenix_MotorControl_ConfigClosedLoopConstants.vi"("PhoenixMotorControlDevRef"=w1410, "slotIdx"=3, "P"=0.1, "I"=0.001, "D"=0.0, "error in (no error)"=w1409) -> ("PhoenixMotorControlDevRef"=w1406:T7, "error out"=w1407:errorcluster)  [unwired: 8 in]
            n703 = Multiply(x=3.413, y=w1389) -> (x*y=w1397:dbl)
            n704 = call <vilib>:"CTRE_Phoenix_MotorControl_SelectProfile Slot.vi"("error in (no error)"=w1407, "slotIdx"=3, "PhoenixMotorControlDevRef"=w1406) -> ("error out"=w1405:errorcluster, "PhoenixMotorControlDevRef"=w1404:T7)  [unwired: 7 in]
            n705 = case shown="True" w1379 {
              tunnel: [FALSE w1412] -> w1390
              frame False {
              }
              frame True {
                n706 = call <vilib>:"WPI_DigitalInputRefNum Registry Get.vi"("refnum name"="Mag Limit") -> ("error out"=w1416:errorcluster, "DigitalInputDevRef"=w1415:T5)  [unwired: 9 in]
                n707 = call <vilib>:"WPI_DigitalInputGetValue.vi"("error in (no error)"=w1416, "DigitalInputDevRef"=w1415) -> ("Value"=w1413:bool)  [unwired: 7 in, 2 out]
                n708 = Not(x=w1413) -> (.not. x?=w1412:bool)
              }
            }
            n709 = call <vilib>:"CTRE_Phoenix_MotorControl_Set.vi"("error in (no error)"=w1405, "Output"=w1397, "Control Mode"=w1403, "PhoenixMotorControlDevRef"=w1404) -> ()  [unwired: 6 in, 2 out]
            n710 = call <vilib>:"CTRE_Phoenix_MotorControl_RefNumRegistryGet.vi"("refnum name"="Mag") -> ("error out"=w1395:errorcluster, "PhoenixMotorControlDevRef"=w1394:T7)  [unwired: 9 in]
            n711 = call <vilib>:"WPI_RobotDriveRefNum Registry Get.vi"("refnum name"="Craig") -> ("error out"=w1371:errorcluster, "RobotDriveDevRef"=w1372:T21)  [unwired: 9 in]
            n712 = call <vilib>:"CTRE_Phoenix_MotorControl_Set.vi"("error in (no error)"=w1395, "Output"=0.9, "Control Mode"=w1393, "PhoenixMotorControlDevRef"=w1394) -> ()  [unwired: 6 in, 2 out]
            n713 = global read "Lime.vi" "Rotate"() -> (w1367:dbl)
            n714 = call-poly <vilib>:"WPI_RobotDriveHolonomicDrive.vi"("Rotation"=w1367, "error in (no error)"=w1371, "Y"=0.0, "X"=0.0, "RobotDriveDevRef"=w1372) -> ()  [unwired: 4 in, 3 out]
            n715 = call <vilib>:"CTRE_Phoenix_MotorControl_RefNumRegistryGet.vi"("refnum name"="Mag") -> ("error out"=w1383:errorcluster, "PhoenixMotorControlDevRef"=w1384:T7)  [unwired: 9 in]
            n716 = call-poly <vilib>:"CTRE_Phoenix_MotorController_Get_TalonFX.vi"("PhoenixMotorControlDevRef"=w1384, "error in"=w1383) -> ("Position (Raw Sensor Units)"=w1382:i32)  [unwired: 10 in, 3 out]
            n717 = call-poly <vilib>:"NT Read Value.vi"("Default Value"=140000.0, "Name"="Encoder") -> ("Numeric"=w1380:dbl)  [unwired: 8 in, 1 out]
            n718 = To Long Integer(number=w1380) -> (32bit integer=w1381:i32)
            n719 = Greater?(x=w1382, y=w1381) -> (0:w1388:bool)
            n720 = Or(x=w1390, y=w1388) -> (x .or. y?=w1374:bool)
            n721 = Select(t=Auto_State_Machine."Reverse", s=w1374, f=Auto_State_Machine."LL Shoot 2") -> (s? t:f=w1373:T2)
          }
          frame "Pigeon Rotate" {
            w1430 = 100.0 ("y")
            w1451 = T16 2 items=["PercentOutput"=0, "Position"=1, "Velocity"=2, "Current"=3, "Follower"=5, "MotionProfile"=6, "MotionMagic"=7, "MotionProfileArc"=10, "Disabled"=15] ("Control Mode")
            w1466 = T16 0 items=["PercentOutput"=0, "Position"=1, "Velocity"=2, "Current"=3, "Follower"=5, "MotionProfile"=6, "MotionMagic"=7, "MotionProfileArc"=10, "Disabled"=15] ("Control Mode")
            w1470 = 5.0 ("lower limit")
            n722 = Negate(x=3400.0 ("Default Value")) -> (-x=w1438:dbl)
            n723 = call <vilib>:"CTRE_Phoenix_MotorControl_RefNumRegistryGet.vi"("refnum name"="Shooter") -> ("error out"=w1457:errorcluster, "PhoenixMotorControlDevRef"=w1458:T7)  [unwired: 9 in]
            n724 = global write "Lime.vi" "Timer Reset"(TRUE ("RPM Good")) -> ()
            n725 = global write "Lime.vi" "Enabled"(FALSE ("Enabled")) -> ()
            n726 = call <vilib>:"CTRE_PigeonIMU_RefNumRegistryGet.vi"("refnum name"="Pigeon") -> ("error out"=w1481:errorcluster, "PigeonIMUDevRef"=w1482:T11)  [unwired: 9 in]
            n727 = call <vilib>:"CTRE_Phoenix_MotorControl_ConfigClosedLoopConstants.vi"("PhoenixMotorControlDevRef"=w1458, "slotIdx"=3, "P"=0.1, "I"=0.001, "D"=0.0, "error in (no error)"=w1457) -> ("PhoenixMotorControlDevRef"=w1454:T7, "error out"=w1455:errorcluster)  [unwired: 8 in]
            n728 = Multiply(x=3.413, y=w1438) -> (x*y=w1441:dbl)
            n729 = call <vilib>:"CTRE_Phoenix_MotorControl_SelectProfile Slot.vi"("error in (no error)"=w1455, "slotIdx"=3, "PhoenixMotorControlDevRef"=w1454) -> ("error out"=w1453:errorcluster, "PhoenixMotorControlDevRef"=w1452:T7)  [unwired: 7 in]
            n730 = call-poly <vilib>:"CTRE_PigeonIMU_GetData.vi"("error in (no error)"=w1481, "PigeonIMUDevRef"=w1482) -> ("Yaw Pitch Roll"=w1479:cluster{"Yaw":dbl, "Pitch":dbl, "Roll":dbl})  [unwired: 7 in, 2 out]
            n731 = call <vilib>:"CTRE_Phoenix_MotorControl_Set.vi"("error in (no error)"=w1453, "Output"=w1441, "Control Mode"=w1451, "PhoenixMotorControlDevRef"=w1452) -> ("error out"=w1444:errorcluster, "PhoenixMotorControlDevRef"=w1445:T7)  [unwired: 6 in]
            n732 = Unbundle(w1479) -> ("Yaw"=w1473:dbl)  [unwired: 2 out]
            "Yaw 6" <- w1473
            n733 = call-poly <vilib>:"CTRE_Phoenix_MotorController_Get_TalonFX.vi"("PhoenixMotorControlDevRef"=w1445, "error in"=w1444) -> ("Velocity"=w1439:dbl)  [unwired: 9 in, 4 out]
            n734 = call-poly <vilib>:"PID.vi"("output range"=cluster{"output high":dbl, "output low":dbl} {"output high"=100.0, "output low"=-100.0}, "PID gains"="PID gains 6", "process variable"=w1473, "setpoint"="setpoint 5") -> ("output"=w1476:dbl)  [unwired: 6 in, 1 out]
            n735 = Add(x="setpoint 5", y=w1470) -> (x+y=w1472:dbl)
            n736 = Subtract(x="setpoint 5", y=w1470) -> (x-y=w1471:dbl)
            n737 = In Range and Coerce(upper limit=w1472, x=w1473, lower limit=w1471) -> (In Range?=w1427:bool)  [unwired: 1 out]
            n738 = Divide(x=w1476, y=100.0) -> (x/y=w1421:dbl)
            n739 = Negate(x=w1421) -> (-x=w1420:dbl)
            n740 = Add(x=w1441, y=w1430) -> (x+y=w1442:dbl)
            n741 = Subtract(x=w1441, y=w1430) -> (x-y=w1443:dbl)
            n742 = In Range and Coerce(upper limit=w1442, x=w1439, lower limit=w1443) -> (In Range?=w1436:bool)  [unwired: 1 out]
            n743 = call <vilib>:"WPI_RobotDriveRefNum Registry Get.vi"("refnum name"="Craig") -> ("error out"=w1484:errorcluster, "RobotDriveDevRef"=w1485:T21)  [unwired: 9 in]
            n744 = call-poly <vilib>:"NT Write Value.vi"("Boolean"=TRUE, "Name"="Blind Shot") -> ()  [unwired: 9 in, 1 out]
            n745 = call-poly <vilib>:"WPI_RobotDriveHolonomicDrive.vi"("Rotation"=w1420, "error in (no error)"=w1484, "Y"=0.0, "X"=0.0, "RobotDriveDevRef"=w1485) -> ()  [unwired: 4 in, 3 out]
            n746 = call <vilib>:"CTRE_Phoenix_MotorControl_RefNumRegistryGet.vi"("refnum name"="Intake") -> ("error out"=w1468:errorcluster, "PhoenixMotorControlDevRef"=w1467:T7)  [unwired: 9 in]
            n747 = call <vilib>:"WPI_DigitalInputRefNum Registry Get.vi"("refnum name"="BB1") -> ("error out"=w1425:errorcluster, "DigitalInputDevRef"=w1424:T5)  [unwired: 9 in]
            n748 = call <vilib>:"WPI_SolenoidRefNum Registry Get.vi"("refnum name"="Intake") -> ("error out"=w1462:errorcluster, "SolenoidDevRef"=w1461:T19)  [unwired: 9 in]
            n749 = call-poly <vilib>:"WPI_SolenoidSet.vi"("error in (no error)"=w1462, "Value"=WPI_SolenoidValue."Reverse", "SolenoidDevRef"=w1461) -> ()  [unwired: 7 in, 2 out]
            n750 = call <vilib>:"WPI_DigitalInputGetValue.vi"("error in (no error)"=w1425, "DigitalInputDevRef"=w1424) -> ("Value"=w1423:bool)  [unwired: 7 in, 2 out]
            n751 = call <vilib>:"CTRE_Phoenix_MotorControl_Set.vi"("error in (no error)"=w1468, "Output"=-1.0, "Control Mode"=w1466, "PhoenixMotorControlDevRef"=w1467) -> ()  [unwired: 6 in, 2 out]
            n752 = Compound Arithmetic op=AND(w1436, w1427) -> (w1435:bool)
            n753 = Not(x=w1423) -> (.not. x?=w1422:bool)
            n754 = Select(t=Auto_State_Machine."Pigeon Shoot 1", s=w1422, f=Auto_State_Machine."Pigeon Shoot 2") -> (s? t:f=w1432:T2)
            n755 = Select(t=w1432, s=w1435, f=Auto_State_Machine."Pigeon Rotate") -> (s? t:f=w1428:T2)
          }
          frame "Pigeon Shoot 1" {
            w1523 = T16 0 items=["PercentOutput"=0, "Position"=1, "Velocity"=2, "Current"=3, "Follower"=5, "MotionProfile"=6, "MotionMagic"=7, "MotionProfileArc"=10, "Disabled"=15] ("Control Mode")
            w1533 = T16 2 items=["PercentOutput"=0, "Position"=1, "Velocity"=2, "Current"=3, "Follower"=5, "MotionProfile"=6, "MotionMagic"=7, "MotionProfileArc"=10, "Disabled"=15] ("Control Mode")
            n756 = call <vilib>:"CTRE_PigeonIMU_RefNumRegistryGet.vi"("refnum name"="Pigeon") -> ("error out"=w1501:errorcluster, "PigeonIMUDevRef"=w1502:T11)  [unwired: 9 in]
            n757 = call-poly <vilib>:"CTRE_PigeonIMU_GetData.vi"("error in (no error)"=w1501, "PigeonIMUDevRef"=w1502) -> ("Yaw Pitch Roll"=w1499:cluster{"Yaw":dbl, "Pitch":dbl, "Roll":dbl})  [unwired: 7 in, 2 out]
            n758 = global write "Lime.vi" "Timer Reset"(FALSE ("RPM Good")) -> ()
            n759 = Negate(x=3400.0) -> (-x=w1519:dbl)
            n760 = call <vilib>:"CTRE_Phoenix_MotorControl_RefNumRegistryGet.vi"("refnum name"="Shooter") -> ("error out"=w1539:errorcluster, "PhoenixMotorControlDevRef"=w1540:T7)  [unwired: 9 in]
            n761 = Unbundle(w1499) -> ("Yaw"=w1494:dbl)  [unwired: 2 out]
            "Yaw 8" <- w1494
            n762 = global read "Lime.vi" "Timer Good"() -> (w1508:bool)
            n763 = call-poly <vilib>:"PID.vi"("output range"=cluster{"output high":dbl, "output low":dbl} {"output high"=100.0, "output low"=-100.0}, "PID gains"="PID gains 8", "process variable"=w1494, "setpoint"="setpoint 7") -> ("output"=w1496:dbl)  [unwired: 6 in, 1 out]
            n764 = call <vilib>:"CTRE_Phoenix_MotorControl_ConfigClosedLoopConstants.vi"("PhoenixMotorControlDevRef"=w1540, "slotIdx"=3, "P"=0.1, "I"=0.001, "D"=0.0, "error in (no error)"=w1539) -> ("PhoenixMotorControlDevRef"=w1536:T7, "error out"=w1537:errorcluster)  [unwired: 8 in]
            n765 = Multiply(x=3.413, y=w1519) -> (x*y=w1527:dbl)
            n766 = call <vilib>:"CTRE_Phoenix_MotorControl_SelectProfile Slot.vi"("error in (no error)"=w1537, "slotIdx"=3, "PhoenixMotorControlDevRef"=w1536) -> ("error out"=w1535:errorcluster, "PhoenixMotorControlDevRef"=w1534:T7)  [unwired: 7 in]
            n767 = Divide(x=w1496, y=100.0) -> (x/y=w1487:dbl)
            n768 = Negate(x=w1487) -> (-x=w1486:dbl)
            n769 = case shown="True" w1508 {
              tunnel: [FALSE w1542] -> w1520
              frame False {
              }
              frame True {
                n770 = call <vilib>:"WPI_DigitalInputRefNum Registry Get.vi"("refnum name"="Mag Limit") -> ("error out"=w1546:errorcluster, "DigitalInputDevRef"=w1545:T5)  [unwired: 9 in]
                n771 = call <vilib>:"WPI_DigitalInputGetValue.vi"("error in (no error)"=w1546, "DigitalInputDevRef"=w1545) -> ("Value"=w1543:bool)  [unwired: 7 in, 2 out]
                n772 = Not(x=w1543) -> (.not. x?=w1542:bool)
              }
            }
            n773 = call <vilib>:"CTRE_Phoenix_MotorControl_Set.vi"("error in (no error)"=w1535, "Output"=w1527, "Control Mode"=w1533, "PhoenixMotorControlDevRef"=w1534) -> ()  [unwired: 6 in, 2 out]
            n774 = call <vilib>:"WPI_RobotDriveRefNum Registry Get.vi"("refnum name"="Craig") -> ("error out"=w1491:errorcluster, "RobotDriveDevRef"=w1492:T21)  [unwired: 9 in]
            n775 = call <vilib>:"CTRE_Phoenix_MotorControl_RefNumRegistryGet.vi"("refnum name"="Mag") -> ("error out"=w1525:errorcluster, "PhoenixMotorControlDevRef"=w1524:T7)  [unwired: 9 in]
            n776 = call-poly <vilib>:"WPI_RobotDriveHolonomicDrive.vi"("Rotation"=w1486, "error in (no error)"=w1491, "Y"=0.0, "X"=0.0, "RobotDriveDevRef"=w1492) -> ()  [unwired: 4 in, 3 out]
            n777 = call <vilib>:"CTRE_Phoenix_MotorControl_Set.vi"("error in (no error)"=w1525, "Output"=0.9, "Control Mode"=w1523, "PhoenixMotorControlDevRef"=w1524) -> ()  [unwired: 6 in, 2 out]
            n778 = call <vilib>:"CTRE_Phoenix_MotorControl_RefNumRegistryGet.vi"("refnum name"="Mag") -> ("error out"=w1512:errorcluster, "PhoenixMotorControlDevRef"=w1513:T7)  [unwired: 9 in]
            n779 = call-poly <vilib>:"CTRE_Phoenix_MotorController_Get_TalonFX.vi"("PhoenixMotorControlDevRef"=w1513, "error in"=w1512) -> ("Position (Raw Sensor Units)"=w1511:i32)  [unwired: 10 in, 3 out]
            n780 = call-poly <vilib>:"NT Read Value.vi"("Default Value"=140000.0, "Name"="Encoder") -> ("Numeric"=w1509:dbl)  [unwired: 8 in, 1 out]
            n781 = To Long Integer(number=w1509) -> (32bit integer=w1510:i32)
            n782 = Greater?(x=w1511, y=w1510) -> (0:w1517:bool)
            n783 = Or(x=w1520, y=w1517) -> (x .or. y?=w1518:bool)
            n784 = Select(t=Auto_State_Machine."Pigeon Rotate", s=w1518, f=Auto_State_Machine."Pigeon Shoot 1") -> (s? t:f=w1503:T2)
          }
          frame "Pigeon Shoot 2" {
            w1584 = T16 0 items=["PercentOutput"=0, "Position"=1, "Velocity"=2, "Current"=3, "Follower"=5, "MotionProfile"=6, "MotionMagic"=7, "MotionProfileArc"=10, "Disabled"=15] ("Control Mode")
            w1594 = T16 2 items=["PercentOutput"=0, "Position"=1, "Velocity"=2, "Current"=3, "Follower"=5, "MotionProfile"=6, "MotionMagic"=7, "MotionProfileArc"=10, "Disabled"=15] ("Control Mode")
            n785 = call <vilib>:"CTRE_PigeonIMU_RefNumRegistryGet.vi"("refnum name"="Pigeon") -> ("error out"=w1562:errorcluster, "PigeonIMUDevRef"=w1563:T11)  [unwired: 9 in]
            n786 = call-poly <vilib>:"CTRE_PigeonIMU_GetData.vi"("error in (no error)"=w1562, "PigeonIMUDevRef"=w1563) -> ("Yaw Pitch Roll"=w1560:cluster{"Yaw":dbl, "Pitch":dbl, "Roll":dbl})  [unwired: 7 in, 2 out]
            n787 = Unbundle(w1560) -> ("Yaw"=w1554:dbl)  [unwired: 2 out]
            "Yaw 9" <- w1554
            n788 = global write "Lime.vi" "Timer Reset"(FALSE ("RPM Good")) -> ()
            n789 = Negate(x=3400.0) -> (-x=w1580:dbl)
            n790 = call <vilib>:"CTRE_Phoenix_MotorControl_RefNumRegistryGet.vi"("refnum name"="Shooter") -> ("error out"=w1600:errorcluster, "PhoenixMotorControlDevRef"=w1601:T7)  [unwired: 9 in]
            n791 = call-poly <vilib>:"PID.vi"("output range"=cluster{"output high":dbl, "output low":dbl} {"output high"=100.0, "output low"=-100.0}, "PID gains"="PID gains 9", "process variable"=w1554, "setpoint"="setpoint 8") -> ("output"=w1556:dbl)  [unwired: 6 in, 1 out]
            n792 = global read "Lime.vi" "Timer Good"() -> (w1569:bool)
            n793 = call <vilib>:"CTRE_Phoenix_MotorControl_ConfigClosedLoopConstants.vi"("PhoenixMotorControlDevRef"=w1601, "slotIdx"=3, "P"=0.1, "I"=0.001, "D"=0.0, "error in (no error)"=w1600) -> ("PhoenixMotorControlDevRef"=w1597:T7, "error out"=w1598:errorcluster)  [unwired: 8 in]
            n794 = Multiply(x=3.413, y=w1580) -> (x*y=w1588:dbl)
            n795 = Divide(x=w1556, y=100.0) -> (x/y=w1557:dbl)
            n796 = Negate(x=w1557) -> (-x=w1547:dbl)
            n797 = call <vilib>:"CTRE_Phoenix_MotorControl_SelectProfile Slot.vi"("error in (no error)"=w1598, "slotIdx"=3, "PhoenixMotorControlDevRef"=w1597) -> ("error out"=w1596:errorcluster, "PhoenixMotorControlDevRef"=w1595:T7)  [unwired: 7 in]
            n798 = case shown="True" w1569 {
              tunnel: [FALSE w1603] -> w1581
              frame False {
              }
              frame True {
                n799 = disable-structure shown="Disabled" {
                  disable-tunnel: [w1608 _] -> _
                  frame Disabled {
                    n800 = call <vilib>:"WPI_DigitalInputRefNum Registry Get.vi"("refnum name"="LS2") -> ("error out"=w1615:errorcluster, "DigitalInputDevRef"=w1616:T5)  [unwired: 9 in]
                    n801 = call <vilib>:"WPI_DigitalInputRefNum Registry Get.vi"("refnum name"="LS1") -> ("error out"=w1611:errorcluster, "DigitalInputDevRef"=w1610:T5)  [unwired: 9 in]
                    n802 = call <vilib>:"WPI_DigitalInputGetValue.vi"("error in (no error)"=w1615, "DigitalInputDevRef"=w1616) -> ("Value"=w1613:bool)  [unwired: 7 in, 2 out]
                    n803 = call <vilib>:"WPI_DigitalInputGetValue.vi"("error in (no error)"=w1611, "DigitalInputDevRef"=w1610) -> ("Value"=w1609:bool)  [unwired: 7 in, 2 out]
                    n804 = Or(x=w1613, y=w1609) -> (x .or. y?=w1608:bool)
                  }
                  frame Enabled {
                  }
                }
                n805 = call <vilib>:"WPI_DigitalInputRefNum Registry Get.vi"("refnum name"="Mag Limit") -> ("error out"=w1607:errorcluster, "DigitalInputDevRef"=w1606:T5)  [unwired: 9 in]
                n806 = call <vilib>:"WPI_DigitalInputGetValue.vi"("error in (no error)"=w1607, "DigitalInputDevRef"=w1606) -> ("Value"=w1604:bool)  [unwired: 7 in, 2 out]
                n807 = Not(x=w1604) -> (.not. x?=w1603:bool)
              }
            }
            n808 = call <vilib>:"CTRE_Phoenix_MotorControl_Set.vi"("error in (no error)"=w1596, "Output"=w1588, "Control Mode"=w1594, "PhoenixMotorControlDevRef"=w1595) -> ()  [unwired: 6 in, 2 out]
            n809 = call <vilib>:"WPI_RobotDriveRefNum Registry Get.vi"("refnum name"="Craig") -> ("error out"=w1551:errorcluster, "RobotDriveDevRef"=w1552:T21)  [unwired: 9 in]
            n810 = call-poly <vilib>:"WPI_RobotDriveHolonomicDrive.vi"("Rotation"=w1547, "error in (no error)"=w1551, "Y"=0.0, "X"=0.0, "RobotDriveDevRef"=w1552) -> ()  [unwired: 4 in, 3 out]
            n811 = call <vilib>:"CTRE_Phoenix_MotorControl_RefNumRegistryGet.vi"("refnum name"="Mag") -> ("error out"=w1586:errorcluster, "PhoenixMotorControlDevRef"=w1585:T7)  [unwired: 9 in]
            n812 = call <vilib>:"CTRE_Phoenix_MotorControl_Set.vi"("error in (no error)"=w1586, "Output"=0.9, "Control Mode"=w1584, "PhoenixMotorControlDevRef"=w1585) -> ()  [unwired: 6 in, 2 out]
            n813 = call <vilib>:"CTRE_Phoenix_MotorControl_RefNumRegistryGet.vi"("refnum name"="Mag") -> ("error out"=w1573:errorcluster, "PhoenixMotorControlDevRef"=w1574:T7)  [unwired: 9 in]
            n814 = call-poly <vilib>:"CTRE_Phoenix_MotorController_Get_TalonFX.vi"("PhoenixMotorControlDevRef"=w1574, "error in"=w1573) -> ("Position (Raw Sensor Units)"=w1572:i32)  [unwired: 10 in, 3 out]
            n815 = call-poly <vilib>:"NT Read Value.vi"("Default Value"=140000.0, "Name"="Encoder") -> ("Numeric"=w1570:dbl)  [unwired: 8 in, 1 out]
            n816 = To Long Integer(number=w1570) -> (32bit integer=w1571:i32)
            n817 = Greater?(x=w1572, y=w1571) -> (0:w1578:bool)
            n818 = Or(x=w1581, y=w1578) -> (x .or. y?=w1579:bool)
            n819 = Select(t=Auto_State_Machine."Reverse", s=w1579, f=Auto_State_Machine."Pigeon Shoot 2") -> (s? t:f=w1564:T2)
          }
          frame "Reverse" {
            w1631 = T16 0 items=["PercentOutput"=0, "Position"=1, "Velocity"=2, "Current"=3, "Follower"=5, "MotionProfile"=6, "MotionMagic"=7, "MotionProfileArc"=10, "Disabled"=15] ("Control Mode")
            w1643 = T16 0 items=["PercentOutput"=0, "Position"=1, "Velocity"=2, "Current"=3, "Follower"=5, "MotionProfile"=6, "MotionMagic"=7, "MotionProfileArc"=10, "Disabled"=15] ("Control Mode")
            w1647 = T16 0 items=["PercentOutput"=0, "Position"=1, "Velocity"=2, "Current"=3, "Follower"=5, "MotionProfile"=6, "MotionMagic"=7, "MotionProfileArc"=10, "Disabled"=15] ("Control Mode")
            n820 = call <vilib>:"WPI_SolenoidRefNum Registry Get.vi"("refnum name"="Intake") -> ("error out"=w1628:errorcluster, "SolenoidDevRef"=w1627:T19)  [unwired: 9 in]
            n821 = call-poly <vilib>:"WPI_SolenoidSet.vi"("error in (no error)"=w1628, "Value"=WPI_SolenoidValue."Reverse", "SolenoidDevRef"=w1627) -> ()  [unwired: 7 in, 2 out]
            n822 = call <vilib>:"CTRE_Phoenix_MotorControl_RefNumRegistryGet.vi"("refnum name"="Shooter") -> ("error out"=w1645:errorcluster, "PhoenixMotorControlDevRef"=w1644:T7)  [unwired: 9 in]
            n823 = call <vilib>:"CTRE_Phoenix_MotorControl_RefNumRegistryGet.vi"("refnum name"="Intake") -> ("error out"=w1633:errorcluster, "PhoenixMotorControlDevRef"=w1632:T7)  [unwired: 9 in]
            n824 = call <vilib>:"CTRE_Phoenix_MotorControl_Set.vi"("error in (no error)"=w1645, "Output"=0.0, "Control Mode"=w1643, "PhoenixMotorControlDevRef"=w1644) -> ()  [unwired: 6 in, 2 out]
            n825 = call <vilib>:"CTRE_Phoenix_MotorControl_RefNumRegistryGet.vi"("refnum name"="Mag") -> ("error out"=w1649:errorcluster, "PhoenixMotorControlDevRef"=w1648:T7)  [unwired: 9 in]
            n826 = call <vilib>:"CTRE_Phoenix_MotorControl_Set.vi"("error in (no error)"=w1633, "Output"=0.0, "Control Mode"=w1631, "PhoenixMotorControlDevRef"=w1632) -> ()  [unwired: 6 in, 2 out]
            n827 = call <vilib>:"CTRE_Phoenix_MotorControl_Set.vi"("error in (no error)"=w1649, "Output"=0.0, "Control Mode"=w1647, "PhoenixMotorControlDevRef"=w1648) -> ()  [unwired: 6 in, 2 out]
            n828 = call <vilib>:"WPI_RobotDriveRefNum Registry Get.vi"("refnum name"="Craig") -> ("error out"=w1639:errorcluster, "RobotDriveDevRef"=w1640:T21)  [unwired: 9 in]
            n829 = call "Elapsed Time12"("Time Target (s)"=0.2, "Reset"=FALSE, "Auto Reset"=FALSE, "Set Start Time (s)"=0.0) -> ("Time has Elapsed"=w1617:bool)  [unwired: 8 in, 7 out]
            n830 = call-poly <vilib>:"WPI_RobotDriveHolonomicDrive.vi"("Rotation"=0.0, "error in (no error)"=w1639, "Y"=0.2, "X"=0.0, "RobotDriveDevRef"=w1640) -> ()  [unwired: 4 in, 3 out]
            n831 = Select(t=Auto_State_Machine."Stop", s=w1617, f=Auto_State_Machine."Reverse") -> (s? t:f=w1620:T2)
          }
          frame "Stop" {
            w1667 = T16 0 items=["PercentOutput"=0, "Position"=1, "Velocity"=2, "Current"=3, "Follower"=5, "MotionProfile"=6, "MotionMagic"=7, "MotionProfileArc"=10, "Disabled"=15] ("Control Mode")
            w1679 = T16 0 items=["PercentOutput"=0, "Position"=1, "Velocity"=2, "Current"=3, "Follower"=5, "MotionProfile"=6, "MotionMagic"=7, "MotionProfileArc"=10, "Disabled"=15] ("Control Mode")
            # "Toggle Buttons"
            n832 = call <vilib>:"WPI_DigitalInputRefNum Registry Get.vi"("refnum name"="Mag Limit") -> ("error out"=w1659:errorcluster, "DigitalInputDevRef"=w1660:T5)  [unwired: 9 in]
            n833 = call <vilib>:"WPI_DigitalInputGetValue.vi"("error in (no error)"=w1659, "DigitalInputDevRef"=w1660) -> ("Value"=w1657:bool)  [unwired: 7 in, 2 out]
            n834 = Not(x=w1657) -> (.not. x?=w1653:bool)
            n835 = feedback #3(FALSE) -> (w1655:bool)
            n836 = feedback-in #3(w1653) -> ()
            n837 = Not(x=w1655) -> (.not. x?=w1656:bool)
            n838 = call <vilib>:"WPI_SolenoidRefNum Registry Get.vi"("refnum name"="Intake") -> ("error out"=w1664:errorcluster, "SolenoidDevRef"=w1663:T19)  [unwired: 9 in]
            n839 = And(x=w1653, y=w1656) -> (x .and. y?=w1651:bool)
            n840 = call-poly <vilib>:"WPI_SolenoidSet.vi"("error in (no error)"=w1664, "Value"=WPI_SolenoidValue."Reverse", "SolenoidDevRef"=w1663) -> ()  [unwired: 7 in, 2 out]
            n841 = feedback #4() -> (w1650:bool)  [unwired: 1 in]
            n842 = case shown="False" w1651 {
              tunnel: [w1682 w1684] -> w1652
              tunnel: w1650 -> [w1682 w1683]
              frame False {
              }
              frame True {
                n843 = Not(x=w1683) -> (.not. x?=w1684:bool)
              }
            }
            n844 = feedback-in #4(w1652) -> ()
            n845 = case shown="True" w1652 {
              frame False {
                w1686 = T16 0 items=["PercentOutput"=0, "Position"=1, "Velocity"=2, "Current"=3, "Follower"=5, "MotionProfile"=6, "MotionMagic"=7, "MotionProfileArc"=10, "Disabled"=15] ("Control Mode")
                w1692 = T16 0 items=["PercentOutput"=0, "Position"=1, "Velocity"=2, "Current"=3, "Follower"=5, "MotionProfile"=6, "MotionMagic"=7, "MotionProfileArc"=10, "Disabled"=15] ("Control Mode")
                n846 = call <vilib>:"CTRE_Phoenix_MotorControl_RefNumRegistryGet.vi"("refnum name"="Mag") -> ("error out"=w1690:errorcluster, "PhoenixMotorControlDevRef"=w1691:T7)  [unwired: 9 in]
                n847 = call <vilib>:"CTRE_Phoenix_MotorControl_Set.vi"("error in (no error)"=w1690, "Output"=0.65, "Control Mode"=w1692, "PhoenixMotorControlDevRef"=w1691) -> ()  [unwired: 6 in, 2 out]
                n848 = call <vilib>:"CTRE_Phoenix_MotorControl_RefNumRegistryGet.vi"("refnum name"="Shooter") -> ("error out"=w1688:errorcluster, "PhoenixMotorControlDevRef"=w1689:T7)  [unwired: 9 in]
                n849 = call <vilib>:"CTRE_Phoenix_MotorControl_Set.vi"("error in (no error)"=w1688, "Output"=0.3, "Control Mode"=w1686, "PhoenixMotorControlDevRef"=w1689) -> ()  [unwired: 6 in, 2 out]
              }
              frame True {
                w1696 = T16 0 items=["PercentOutput"=0, "Position"=1, "Velocity"=2, "Current"=3, "Follower"=5, "MotionProfile"=6, "MotionMagic"=7, "MotionProfileArc"=10, "Disabled"=15] ("Control Mode")
                w1702 = T16 0 items=["PercentOutput"=0, "Position"=1, "Velocity"=2, "Current"=3, "Follower"=5, "MotionProfile"=6, "MotionMagic"=7, "MotionProfileArc"=10, "Disabled"=15] ("Control Mode")
                n850 = call <vilib>:"CTRE_Phoenix_MotorControl_RefNumRegistryGet.vi"("refnum name"="Mag") -> ("error out"=w1700:errorcluster, "PhoenixMotorControlDevRef"=w1701:T7)  [unwired: 9 in]
                n851 = call <vilib>:"CTRE_Phoenix_MotorControl_Set.vi"("error in (no error)"=w1700, "Output"=0.0, "Control Mode"=w1702, "PhoenixMotorControlDevRef"=w1701) -> ()  [unwired: 6 in, 2 out]
                n852 = call <vilib>:"CTRE_Phoenix_MotorControl_RefNumRegistryGet.vi"("refnum name"="Shooter") -> ("error out"=w1698:errorcluster, "PhoenixMotorControlDevRef"=w1699:T7)  [unwired: 9 in]
                n853 = call <vilib>:"CTRE_Phoenix_MotorControl_Set.vi"("error in (no error)"=w1698, "Output"=0.0, "Control Mode"=w1696, "PhoenixMotorControlDevRef"=w1699) -> ()  [unwired: 6 in, 2 out]
              }
            }
            n854 = call <vilib>:"CTRE_Phoenix_MotorControl_RefNumRegistryGet.vi"("refnum name"="Intake") -> ("error out"=w1669:errorcluster, "PhoenixMotorControlDevRef"=w1668:T7)  [unwired: 9 in]
            n855 = call <vilib>:"CTRE_Phoenix_MotorControl_RefNumRegistryGet.vi"("refnum name"="Mag") -> ("error out"=w1681:errorcluster, "PhoenixMotorControlDevRef"=w1680:T7)  [unwired: 9 in]
            n856 = call <vilib>:"CTRE_Phoenix_MotorControl_Set.vi"("error in (no error)"=w1669, "Output"=0.0, "Control Mode"=w1667, "PhoenixMotorControlDevRef"=w1668) -> ()  [unwired: 6 in, 2 out]
            n857 = call <vilib>:"CTRE_Phoenix_MotorControl_Set.vi"("error in (no error)"=w1681, "Output"=0.0, "Control Mode"=w1679, "PhoenixMotorControlDevRef"=w1680) -> ()  [unwired: 6 in, 2 out]
            n858 = call <vilib>:"WPI_RobotDriveRefNum Registry Get.vi"("refnum name"="Craig") -> ("error out"=w1676:errorcluster, "RobotDriveDevRef"=w1677:T21)  [unwired: 9 in]
            n859 = call-poly <vilib>:"WPI_RobotDriveHolonomicDrive.vi"("Rotation"=0.0, "error in (no error)"=w1676, "Y"=0.0, "X"=0.0, "RobotDriveDevRef"=w1677) -> ()  [unwired: 4 in, 3 out]
          }
        }
      }
    }
  }
